vi "Coating Schedule Run Builder.vi"() -> ()   [LabVIEW 2018]
uses:
  <vilib>/Utility/miscctls.llb/LVRowAndColumnTypeDef.ctl
  <vilib>/event_ctls.llb/eventvkey.ctl
  Schedule Control Globals.vi
  <vilib>/Utility/file.llb/Read Delimited Spreadsheet (string).vi
  <vilib>/Utility/file.llb/Write Delimited Spreadsheet (string).vi
panel:
  out "Active File Changed":bool
  out "Transfer was True":bool
  out "Control Cluster was clicked":bool
  out "Track Edit Positions":T1[](array[typedef])
  out "S2 Design # and row":string[](array[string])
  out "S1 Design # and row":string[](array[string])
  out "Part Number Changed":bool
  out "Timer 1 Stpt.":i32=25
  out "Edit Position 2":T1
  out "Return Key was Pressed":bool
  out "Current Table Changed":bool
  out "Substrate Text":string
  out "Coating Que / CTCL (T)?":bool
  out "Reset Substrate Timer Start":u32
  out "Multiple Designs":bool
  out "Lookup Failed":bool
  out "SubstrateStrings":string[](array[string])
  out "Part No Found":bool
  out "Index":i32
  out "Edit Position":T1
  in  "Pick Design was True":bool
  out "Used WO's":string[](array[string])
  out "Sys Select was True":bool
  out "Time Array":string[](array[string])
  out "Part info Row":i32
  out "System No.":string
  out "Worksheet array":string[](array[string])
  out "Wavelengths & Designs":string[][](array[string])
  out "Blank":string
  in  "Diameter":string
  out "Lookup was True":bool
  out "Timer 1":i32
  in  "Tab Control":enum32{"Workcenter Report", "Run Worksheet"}(tab)=enum."Run Worksheet"
  in  "Show Part Info":bool=TRUE
  out "Report Name":string="Coating Que"
  in  "Select Action 2":bool
  in  "Select Action":bool
  out "Total Unused":i32
  out "Un-used WO's":bool caption="Showing Un-used WO's when \"ON\""
  out "last mod":u32 format="%<%m/%d/%Y>T"
  in  "Search Again":bool
  in  "Options":u16(ring) items=["Options", "Sort by Due Date", "Sort By Part Number", "Sort By Part Description", "Un-Sort / Undo", "Show New WO's Only", "Search"]
  in  "Apply to WorkSheet":bool
  out "Converted Data Table":string[][](table)
  in  "Search Text":string caption="Find What"
  in  "System Select Cluster":T2={"Select System"=1, "OK Button"=FALSE, "Cancel Button"=FALSE} {"Select System" items=["10", "20", "25", "120", "100", "41", "61", "90", "70", "160", "140", "150", "180", "190", "130", "200", "210", "220", "230", "240"]}
  in  "Always Sched. w/o OverWrite":bool caption="Always Schedule w/o Overwrite"
  in  "Include WO & PN":bool
  in  "Save Column Widths as Default":bool
  in  "Disable Pop-up":bool caption="Disable \"Design Check\" pop-up"
  in  "Reset Substrate List":bool
  in  "System Cluster 2":T3 {"Select System" items=["190", "190", "190"]}
  in  "Transfer to Schedule":bool
  out "Part Description":string caption="Part Description of Last Searched"
  in  "Control Cluster":T4
  in  "Add to Worksheet":bool
  in  "Pick Design":bool
  in  "Other Options":u16(ring) items=["Other Options", "Update Substrate List", "Print This Worksheet", "Print All Worksheets", "Open New Part Number Designs program"]
  in  "Wavelength":u16(ring) caption="Select Wavelength" items=["-"]
  in  "Substrate":u16(ring) caption="Select Substrate" items=[".55in. Quartz crystals", "AMTIR", "Al", "Aluminum", "Aluminum Tubes", "Amtir#1", "Any", "BK-7", "BK-7 Glass", "BaF2", "Be", "Bk7", "CSI", "CaF2", "CaF4", "CdS", "CdTe", "Copper", "Cu", "Cu Button", "Cu-x", "Diamond", "ER:YAG", "Fused Silica", "Fusedsilica", "GASIR-1", "GaAs", "GaAs Wafer", "Ge", "Ge Doublets", "Ge Wafers", "Glass", "Infrasil", "KBr (Salt)", "KCl", "MgO", "None", "Other", "Quartz", "SF-11", "Sapphire", "Si", "Si OG", "SiC", "Silicon Carbide", "Tool", "YAG", "YSGG", "ZnS", "ZnS (Cleartran)", "ZnS (Multispectral)", "ZnSe"]
  in  "Coating Type":u16(ring) caption="Select Coating Type / Description" items=["5 MHz Cu/Ag Crystals - side 1", "5 MHz Cu/Ag Crystals - side 1 - auto", "5 MHz Cu/Ag Crystals - side 2", "5 MHz Cu/Ag Crystals - side 2 - auto", "6 MHz Au/Ag Crystals - side 2", "6 MHz Cu/Ag Crystals - side 1"]
  in  "Design# Match/es":u16(ring) caption="Select Design#" items=["XTAL5mhzCuAgNiCrS1", "XTAL5mhzCuAgNiCrS1-auto", "Xtal17 -5mhzCuAgNiCrS1Auto"]
  in  "System Select":u16(ring) caption="Select System" items=["10", "20", "25", "120", "100", "41", "61", "90", "70", "160", "140", "150", "180", "190", "130", "200", "210", "220", "230", "240"]
  in  "Run Worksheet":string[][](table)
  out "Work Order":string
  out "Qty":string
  out "Part Number":string
  in  "Not Scheduled":bool caption="Set as Not Scheduled"
  in  "Transfer to Other Worksheet":bool caption="Move Selected Row to Different System"
  out "Coating, Wavel, Design":string[][](array[string])
  out "Build Substr":string
  out "Substrates 2":string[](array[string])
  out "Design No.":string
  in  "Data Trigger":string="f2 "
  out "Wavelength F":string
  out "Possible Designs":string[](array[string])
  out "Substrate 2":string
  out "Wavelength 2":string
  out "Coating Type 2":string
  out "Wavelengths":string[](array[string])
  in  "X-Position Array":string[](array[string])=["336", "1500", "2136", "2976", "3696", "4176", "4896", "6336", "10056", "10896", "12336", "13056", "0", "0", "0", "0", "0", "0", "0", "0", "0"]
  in  "Start Data String":string="Wavelength"
  in  "No of Columns":i32=12
  # "Coating Schedule Run Builder"
  # "Run Worksheet"
  # "Select System to Copy to"
  # "The part number was found on the system's listed.  Select one of the system's designs by selecting the system number.  Then click the desired button."
  # "Insert\n Row"
  # "Delete\nRow"
  # "Move\nUp"
  # "Move\nDown"
  # "New\nRun"
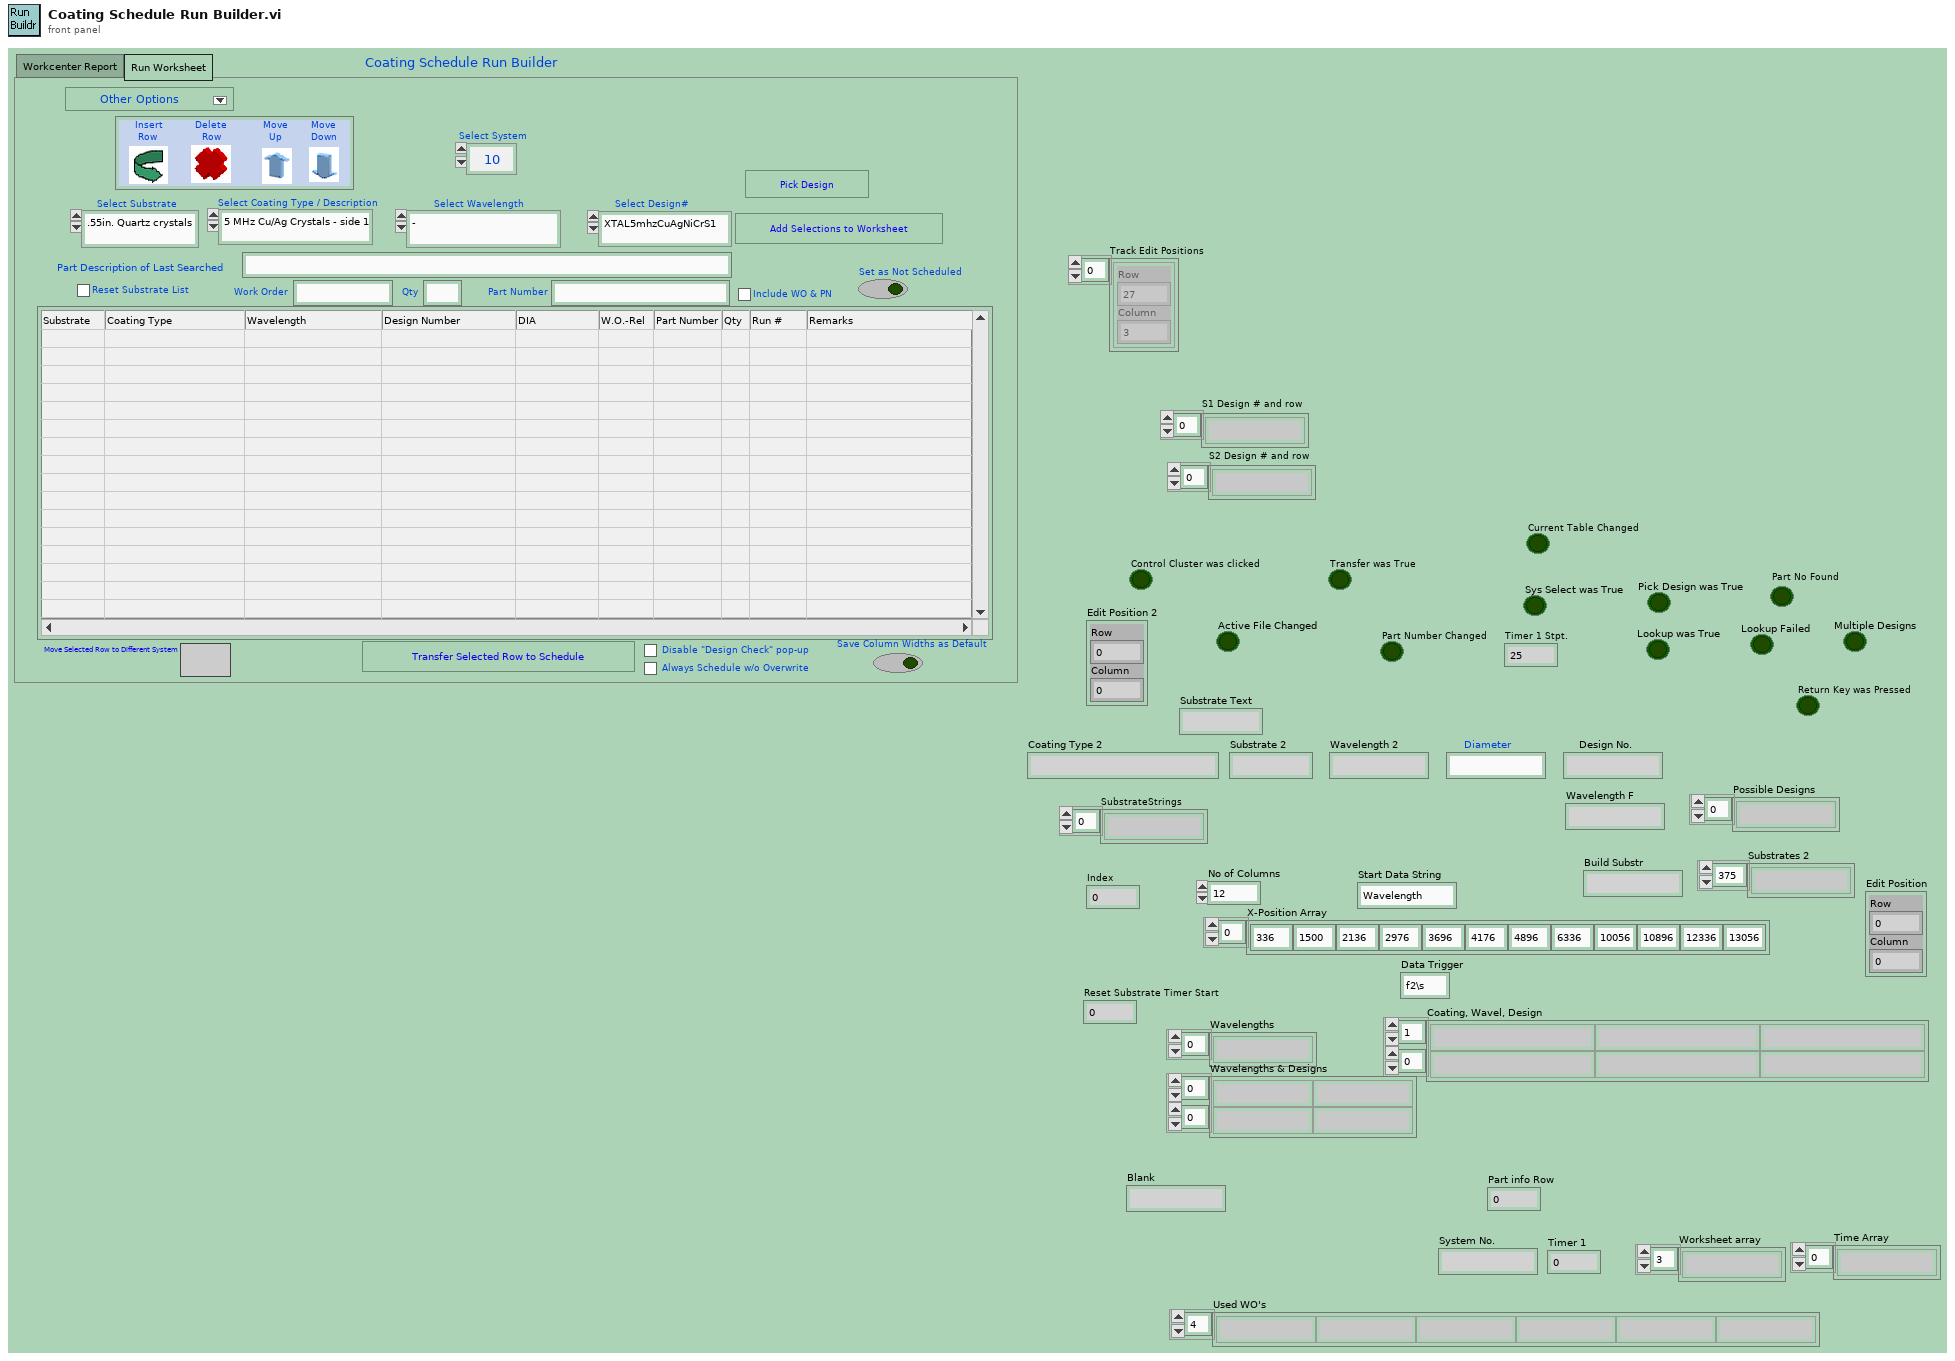
[diagram p1: front panel]
types:
  T1 = typedef "LVRowAndColumnTypeDef.ctl" = cluster{"Row":i32, "Column":i32}
  T2 = cluster{"Select System":u16, "OK Button":bool, "Cancel Button":bool}
  T3 = cluster{"Select System":u16, "OK Button":bool, "Cancel":bool, "Design #":string, "Side#":string}
  T4 = cluster{"Insert Row":bool, "Delete Row":bool, "Move Up":bool, "Move Down":bool, "New Run":bool, "Add Delay":bool}
  T5 = enum8{"Enabled", "Disabled", "Disabled and Grayed Out"}
  T6 = enum16{"Sort by Number", "Sort By Name", "Sort by Date"}
  T7 = typedef "eventvkey.ctl" = enum16{"ASCII", "Enter", "Return", "Shift", "Ctrl", "Alt", "Cmd", "Opt", "Caps", "NumLock", "Clear", "Break", "Up", "Down", "Left", "Right", "Insert", "Delete", "Home", "End", "PageUp", "PageDown", "Escape", "Help", "Pause", "ScrollLock", "F1", "F2", "F3", "F4", "F5", "F6", "F7", "F8", "F9", "F10", "F11", "F12", "F13", "F14", "F15", "F16", "F17", "F18", "F19", "F20", "F21", "F22", "F23", "F24", "Play", "VolumeUp", "VolumeDown", "Mute", "Two Byte Char"}
  T8 = cluster{"Insert Row":bool, "Insert Row":bool, "Insert Row":bool, "Insert Row":bool, "Insert Row":bool, "Insert Row":bool}
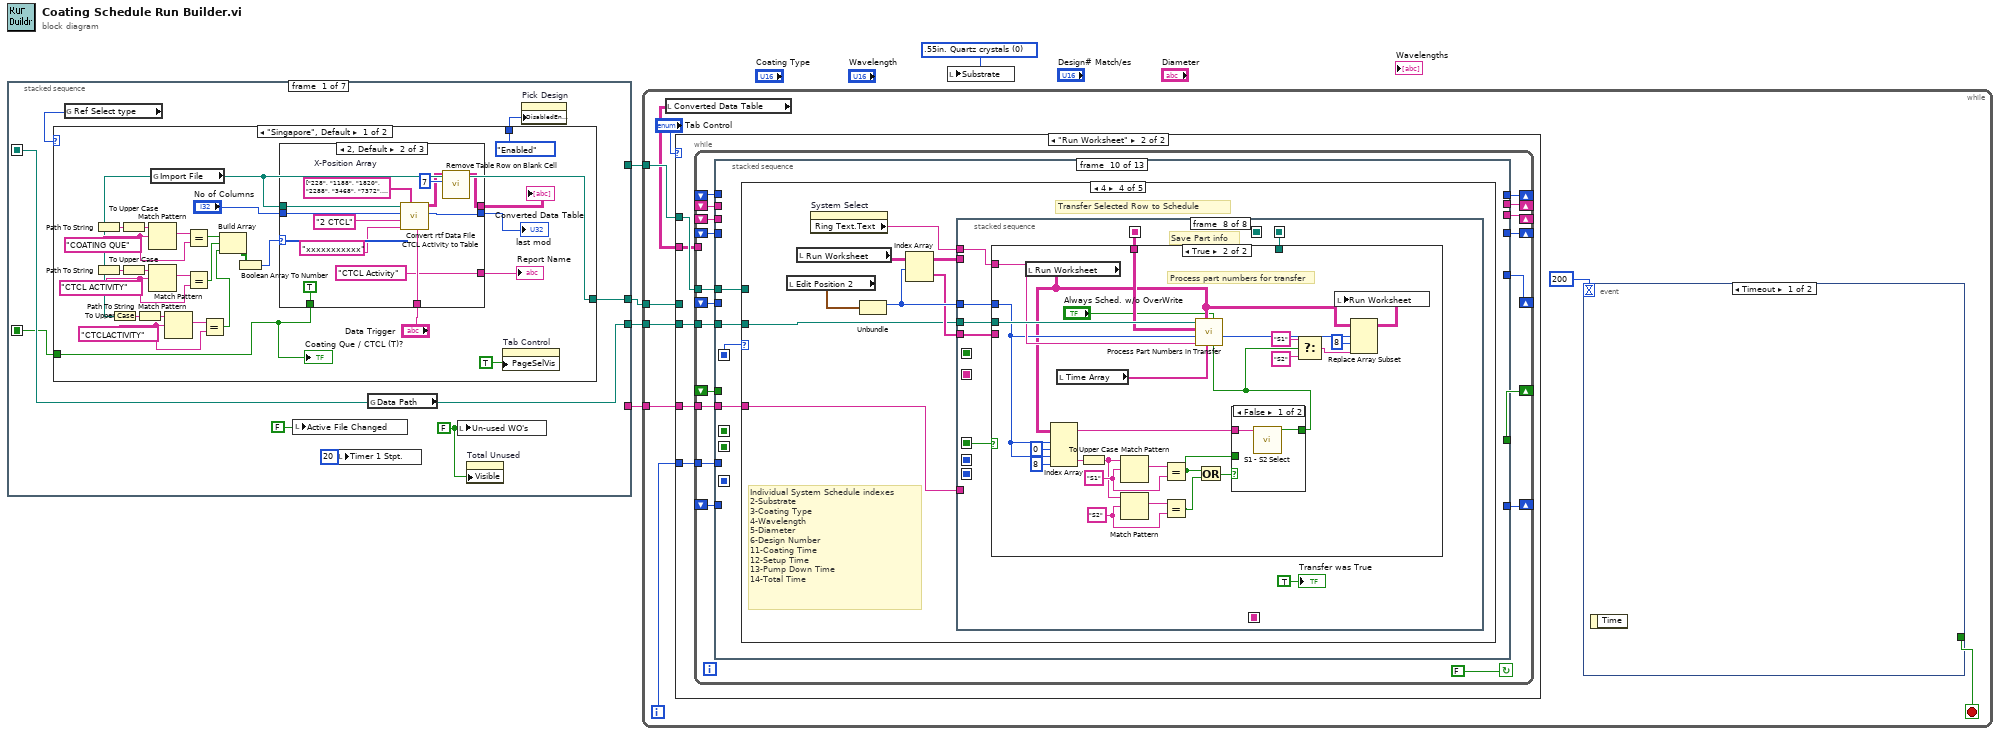
[diagram p0: block diagram]
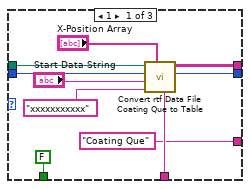
[diagram p2: hidden frame]
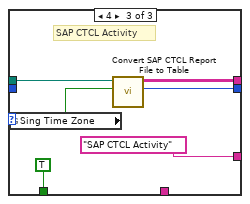
[diagram p3: hidden frame]
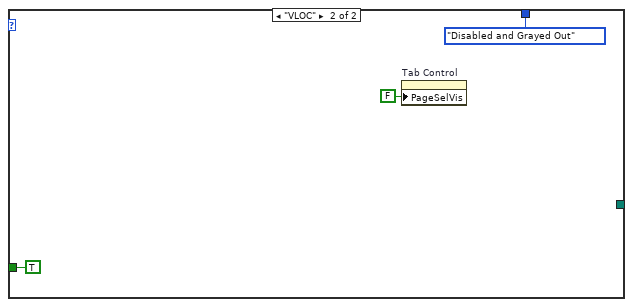
[diagram p4: hidden frame]
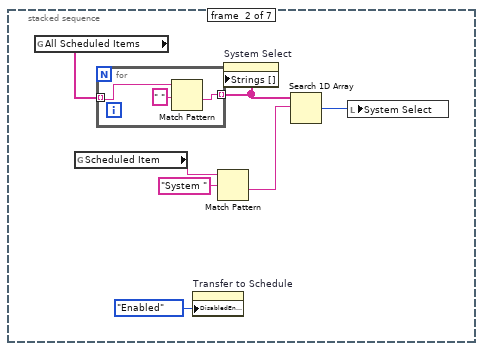
[diagram p5: hidden frame]
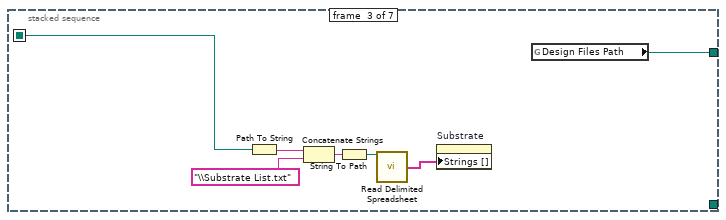
[diagram p6: hidden frame]
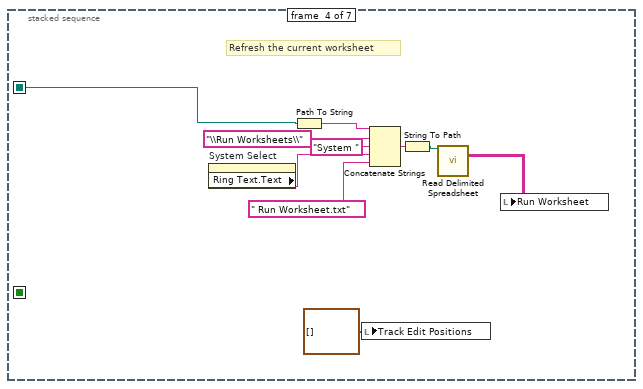
[diagram p7: hidden frame]
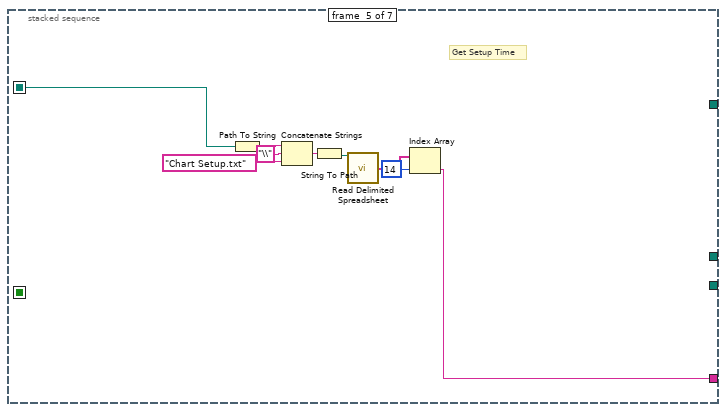
[diagram p8: hidden frame]
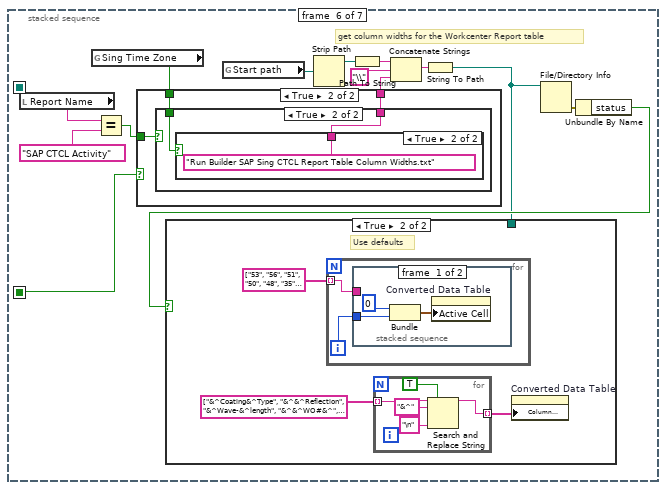
[diagram p9: hidden frame]
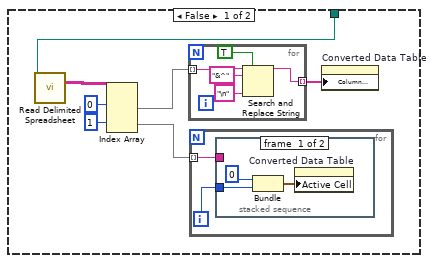
[diagram p10: hidden frame]
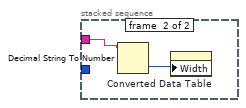
[diagram p11: hidden frame]
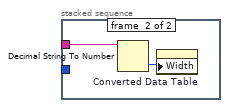
[diagram p12: hidden frame]
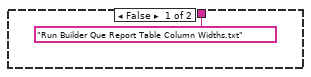
[diagram p13: hidden frame]
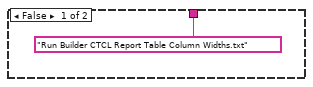
[diagram p14: hidden frame]
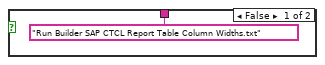
[diagram p15: hidden frame]
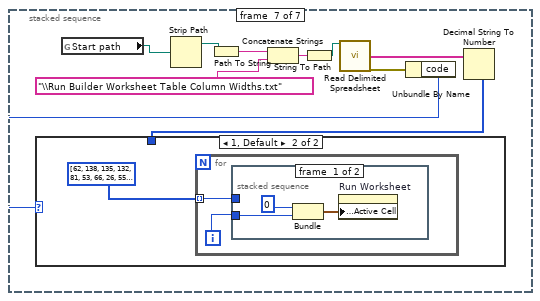
[diagram p16: hidden frame]
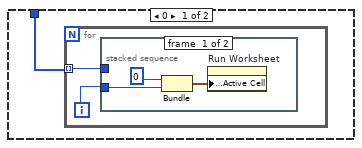
[diagram p17: hidden frame]
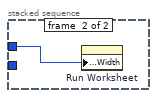
[diagram p18: hidden frame]
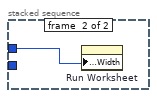
[diagram p19: hidden frame]
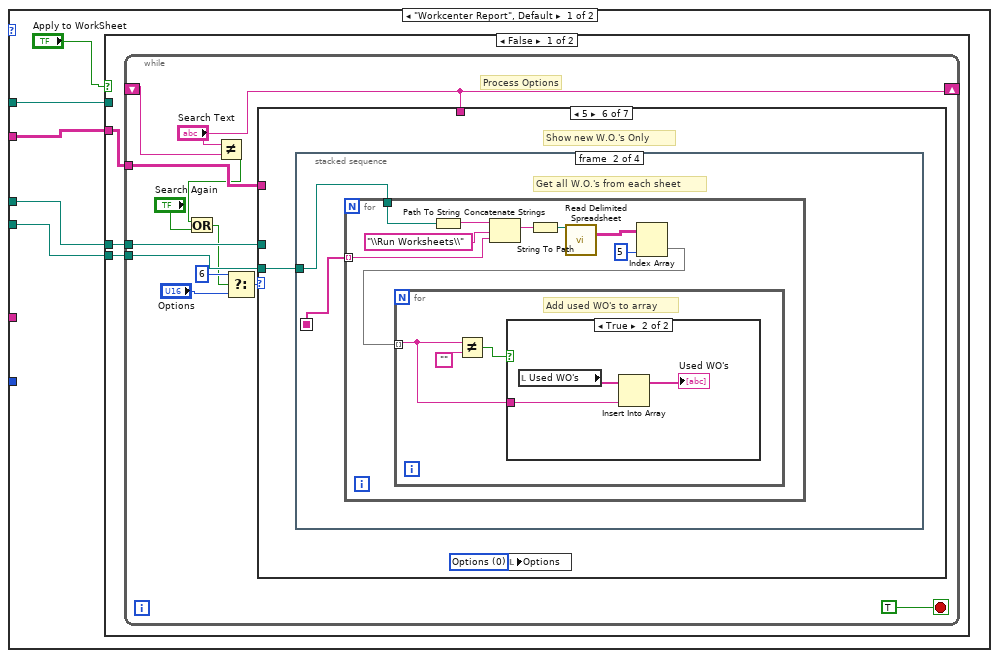
[diagram p20: hidden frame]
diagram:
  w3 = u16 0 items=[".55in. Quartz crystals", "AMTIR", "Al", "Aluminum Tubes", "Amtir#1", "Any", "Any(NT)", "BK-7", "BaF2", "Be", "Bk7", "CSI", "CaF2", "CaF4", "CdS", "CdTe", "Cu", "Diamond", "ER:YAG", "Fused Silica", "GASIR-1", "GLASS", "GaAs", "GaAs Wafer", "Ge", "Ge Doublets", "Ge Wafers", "Glass", "Infrasil", "KBr (Salt)", "KCl", "MgO", "None", "Other", "Quartz", "SF-11", "Sapphire", "Si", "Si OG", "SiC", "Tool", "YAG", "YSGG", "ZnS", "ZnS (Cleartran)", "ZnS (Multispectral)", "ZnSe"] ("Substrate")
  n1 = stacked-sequence {
    seq-local: [w13 _ _ _ _ _ _] -> [_ _ w83 w91 w102 _ _]
    seq-local: [w8 _ _ _ _ _ _] -> [_ _ _ _ _ w111 _]
    tunnel: [w13 _ _ _ _ _ _] -> w5
    tunnel: [_ _ w87 _ _ _ _] -> w4
    tunnel: [w11 _ _ _ _ _ _] -> w2
    tunnel: [_ _ _ _ w100 _ _] -> w1
    frame #0 {
      w12 = FALSE ("Un-used WO's")
      n2 = global read "Schedule Control Globals.vi" "Ref Select type"() -> (w10:enum32{"Singapore", "VLOC"})
      n3 = case shown="\"Singapore\", Default" w10 {
        tunnel: [w20 _] -> w11
        tunnel: [T5."Enabled" ("Disabled") T5."Disabled and Grayed Out" ("Disabled")] -> w9
        tunnel: [w15 TRUE] -> w8
        frame "Singapore", Default {
          w19 = "CTCLACTIVITY" ("regular expression")
          w26 = "CTCL ACTIVITY" ("regular expression")
          w31 = "COATING QUE" ("regular expression")
          n4 = global read "Schedule Control Globals.vi" "Import File"() -> (w20:path)
          n5 = Path To String(path=w20) -> (string=w34:string)
          n6 = Path To String(path=w20) -> (string=w29:string)
          n7 = Path To String(path=w20) -> (string=w23:string)
          n8 = To Upper Case(1:w34) -> (0:w33:string)
          n9 = To Upper Case(1:w29) -> (0:w28:string)
          n10 = To Upper Case(1:w23) -> (0:w22:string)
          n11 = Match Pattern(string=w33, regular expression=w31) -> (match substring=w32:string)  [unwired: 1 in, 3 out]
          n12 = Match Pattern(string=w28, regular expression=w26) -> (match substring=w27:string)  [unwired: 1 in, 3 out]
          n13 = Match Pattern(string=w22, regular expression=w19) -> (match substring=w21:string)  [unwired: 1 in, 3 out]
          n14 = Equal?(x=w32, y=w31) -> (x = y?=w25:bool)
          n15 = Equal?(x=w27, y=w26) -> (x = y?=w24:bool)
          n16 = Equal?(x=w21, y=w19) -> (x = y?=w18:bool)
          n17 = Build Array(w25, w24, w18) -> (w17:bool[])
          n18 = Boolean Array To Number(Boolean array=w17) -> (number=w16:u32)
          n19 = case shown="2, Default" w16 {
            tunnel: "No of Columns" -> [w49 w61 _]
            tunnel: "Data Trigger" -> [w48 w58 _]
            tunnel: [w47 w51 w66] -> w14
            tunnel: [w46 w60 w65] -> w37
            tunnel: w20 -> [w45 w59 w67]
            tunnel: ["Coating Que" ("Report Name") "CTCL Activity" ("Report Name") "SAP CTCL Activity" ("Report Name")] -> w30
            tunnel: [FALSE TRUE TRUE] -> w15
            frame 1 {
              n20 = call "Convert rtf Data File Coating Que to Table.vi"("File Path"=w45, "No of Columns"=w49, "Start Data String"="Start Data String", "End of Data String"="xxxxxxxxxxx", "X-Position Array"="X-Position Array", "Data Trigger"=w48) -> ("Converted Data Table"=w47:string[][], "last mod"=w46:u32)  [unwired: 3 in]
            }
            frame 2, Default {
              w56 = string[] ["228", "1188", "1820", "2288", "3468", "7372", "7788", "8212", "11028", "13668", "0", "0", "0", "0", "0", "0", "0", "0", "0", "0", "0"]  # X-Position Array
              n21 = call "Convert rtf Data File CTCL Activity to Table.vi"("File Path"=w59, "No of Columns"=w61, "Start Data String"="2 CTCL", "End of Data String"="xxxxxxxxxxx", "X-Position Array"=w56, "Data Trigger"=w58) -> ("Converted Data Table"=w52:string[][], "last mod"=w60:u32)  [unwired: 3 in]
              n22 = call "Remove Table Row on Blank Cell.vi"("Column"=7, "Table In"=w52) -> ("Table Out"=w51:string[][])  [unwired: 9 in]
            }
            frame 4 {
              # "SAP CTCL Activity"
              n23 = global read "Schedule Control Globals.vi" "Sing Time Zone"() -> (w62:bool)
              n24 = call "Convert SAP CTCL Report File to Table.vi"("File Path"=w67, "Sing Time Zone"=w62) -> ("Converted Data Table"=w66:string[][], "last mod"=w65:u32)  [unwired: 7 in]
            }
          }
          "last mod" <- w37
          "Report Name" <- w30
          "Coating Que / CTCL (T)?" <- w15
          "Converted Data Table" <- w14
          n25 = property on="Tab Control" class="TabCtl (strict)"("PageSelVis"=TRUE ("Page Selector Visible")) -> ()  [unwired: 2 in, 2 out]
        }
        frame "VLOC" {
          n26 = property on="Tab Control" class="TabCtl (strict)"("PageSelVis"=FALSE ("Page Selector Visible")) -> ()  [unwired: 2 in, 2 out]
        }
      }
      n27 = local write "Active File Changed"(FALSE ("Active File Changed")) -> ()
      n28 = local write "Timer 1 Stpt."(20 ("Timer Stpt.")) -> ()
      n29 = global read "Schedule Control Globals.vi" "Data Path"() -> (w13:path)
      n30 = local write "Un-used WO's"(w12) -> ()
      n31 = property on="Total Unused" class="DigNum (strict)"("Visible"=w12) -> ()  [unwired: 2 in, 2 out]
      n32 = property on="Pick Design" class="Bool"("DisabledEnum"=w9) -> ()  [unwired: 2 in, 2 out]
    }
    frame #1 {
      n33 = global read "Schedule Control Globals.vi" "All Scheduled Items"() -> (w73:string[])
      n34 = global read "Schedule Control Globals.vi" "Scheduled Item"() -> (w72:string)
      n35 = for {
        tunnel: w73 -> [w80] mode=indexing
        tunnel: [w78] -> w77 mode=indexing
        n36 = Match Pattern(string=w80, regular expression=" ") -> (after substring=w78:string)  [unwired: 1 in, 3 out]
      }
      n37 = property on="Transfer to Schedule" class="Bool"("DisabledEnum"=T5."Enabled" ("Disabled")) -> ()  [unwired: 2 in, 2 out]
      n38 = Match Pattern(string=w72, regular expression="System ") -> (after substring=w75:string)  [unwired: 1 in, 3 out]
      n39 = property on="System Select" class="Ring (strict)"("Strings []"=w77) -> ()  [unwired: 2 in, 2 out]
      n40 = Search 1D Array(1D array=w77, element=w75) -> (index of element=w76:i32)  [unwired: 1 in]
      n41 = local write "System Select"(w76) -> ()
    }
    frame #2 {
      n42 = Path To String(path=w83) -> (string=w85:string)
      n43 = Concatenate Strings(w85, "\\Substrate List.txt" ("string")) -> (w86:string)
      n44 = String To Path(string=w86) -> (path=w82:path)
      n45 = call-poly <vilib>:"Read Delimited Spreadsheet.vi"("file path (dialog if empty)"=w82) -> ("first row"=w81:string[])  [unwired: 9 in, 5 out]
      n46 = property on="Substrate" class="Ring (strict)"("Strings []"=w81) -> ()  [unwired: 2 in, 2 out]
      n47 = global read "Schedule Control Globals.vi" "Design Files Path"() -> (w87:path)
    }
    frame #3 {
      # "Refresh the current worksheet"
      n48 = property on="System Select" class="Ring (strict)"() -> ("Ring Text.Text"=w96:string)  [unwired: 2 in, 2 out]
      n49 = Path To String(path=w91) -> (string=w94:string)
      n50 = local write "Track Edit Positions"(T1[] [] ("Track Edit Positions")) -> ()
      n51 = Concatenate Strings(w94, "\\Run Worksheets\\" ("string"), "System " ("string"), w96, " Run Worksheet.txt" ("string")) -> (w92:string)
      n52 = String To Path(string=w92) -> (path=w90:path)
      n53 = call-poly <vilib>:"Read Delimited Spreadsheet.vi"("file path (dialog if empty)"=w90) -> ("all rows"=w89:string[][])  [unwired: 9 in, 5 out]
      n54 = local write "Run Worksheet"(w89) -> ()
    }
    frame #4 {
      # "Get Setup Time"
      n55 = Path To String(path=w102) -> (string=w106:string)
      n56 = Concatenate Strings(w106, "\\" ("string"), "Chart Setup.txt" ("string")) -> (w104:string)
      n57 = String To Path(string=w104) -> (path=w99:path)
      n58 = call-poly <vilib>:"Read Delimited Spreadsheet.vi"("file path (dialog if empty)"=w99) -> ("first row"=w98:string[])  [unwired: 9 in, 5 out]
      n59 = Index Array(array=w98, index=14) -> (element=w100:string)
    }
    frame #5 {
      # "get column widths for the Workcenter Report table"
      n60 = local read "Report Name"() -> (w110:string)
      n61 = global read "Schedule Control Globals.vi" "Sing Time Zone"() -> (w107:bool)
      n62 = Equal?(x=w110, y="SAP CTCL Activity" ("Report Name")) -> (x = y?=w108:bool)
      n63 = case shown="True" w111 {
        tunnel: ["Run Builder Que Report Table Column Widths.txt" ("text") w157] -> w112
        tunnel: w108 -> [_ w158]
        tunnel: w107 -> [_ w156]
        frame False {
        }
        frame True {
          n64 = case shown="True" w158 {
            tunnel: ["Run Builder CTCL Report Table Column Widths.txt" ("text") w161] -> w157
            tunnel: w156 -> [_ w160]
            frame False {
            }
            frame True {
              n65 = case shown="True" w160 {
                tunnel: ["Run Builder SAP CTCL Report Table Column Widths.txt" ("text") "Run Builder SAP Sing CTCL Report Table Column Widths.txt" ("text")] -> w161
                frame False {
                }
                frame True {
                }
              }
            }
          }
        }
      }
      n66 = global read "Schedule Control Globals.vi" "Start path"() -> (w120:path)
      n67 = Strip Path(path=w120) -> (stripped path=w119:path)  [unwired: 1 out]
      n68 = Path To String(path=w119) -> (string=w118:string)
      n69 = Concatenate Strings(w118, "\\" ("string"), w112) -> (w116:string)
      n70 = String To Path(string=w116) -> (path=w113:path)
      n71 = File/Directory Info(path=w113) -> (error out=w115:errorcluster)  [unwired: 1 in, 6 out]
      n72 = Unbundle By Name(w115) -> ("status"=w114:bool)
      n73 = case shown="True" w114 {
        tunnel: w113 -> [w122 _]
        frame False {
          n74 = call-poly <vilib>:"Read Delimited Spreadsheet.vi"("file path (dialog if empty)"=w122) -> ("all rows"=w121:string[][])  [unwired: 9 in, 5 out]
          n75 = Index Array(array=w121, index (row) #1=0 ("index (row)"), index (row) #2=1 ("index (row)")) -> (element #1=w124:string[], element #2=w125:string[])  [unwired: 2 in]
          n76 = for {
            tunnel: w124 -> [w132] mode=indexing
            tunnel: [w128] -> w123 mode=indexing
            n77 = Search and Replace String(replace all?=TRUE ("replace all? (F)"), input string=w132, search string="&^", replace string="\n" ("replace string (\"\")")) -> (result string=w128:string)  [unwired: 4 in, 3 out]
          }
          n78 = for {
            tunnel: w125 -> [w133] mode=indexing
            i -> [w134]
            n79 = stacked-sequence {
              tunnel: w134 -> [w137 _]
              tunnel: w133 -> [_ w139]
              frame #0 {
                n80 = Bundle(0, w137) -> (w135:cluster{i32, i32})  [unwired: 1 in]
                n81 = property on="Converted Data Table" class="Tbl (strict)"("Active Cell"=w135) -> ()  [unwired: 2 in, 2 out]
              }
              frame #1 {
                n82 = Decimal String To Number(string=w139) -> (number=w138:i32)  [unwired: 2 in, 1 out]
                n83 = property on="Converted Data Table" class="Tbl (strict)"("Width"=w138) -> ()  [unwired: 2 in, 2 out]
              }
            }
          }
          n84 = property on="Converted Data Table" class="Tbl (strict)"("Column Headers[]"=w123) -> ()  [unwired: 2 in, 2 out]
        }
        frame True {
          # "Use defaults"
          n85 = for {
            tunnel: string[] ["53", "56", "51", "50", "48", "35", "63", "360", "52", "138", "45", "48", "50", "50", "50", "50", "44", "47", "44", "50", "282"] ("decimal integer string") -> [w148] mode=indexing
            i -> [w149]
            n86 = stacked-sequence {
              tunnel: w149 -> [w152 _]
              tunnel: w148 -> [_ w154]
              frame #0 {
                n87 = Bundle(0, w152) -> (w150:cluster{i32, i32})  [unwired: 1 in]
                n88 = property on="Converted Data Table" class="Tbl (strict)"("Active Cell"=w150) -> ()  [unwired: 2 in, 2 out]
              }
              frame #1 {
                n89 = Decimal String To Number(string=w154) -> (number=w153:i32)  [unwired: 2 in, 1 out]
                n90 = property on="Converted Data Table" class="Tbl (strict)"("Width"=w153) -> ()  [unwired: 2 in, 2 out]
              }
            }
          }
          n91 = for {
            tunnel: string[] ["&^Coating&^Type", "&^&^Reflection", "&^Wave-&^length", "&^&^WO#&^", "&^&^Release", "&^Open&^Qty", "&^Part&^Number", "&^Part&^Description", "&^Due&^Date", "&^&^Customer", "&^&^SO#", "&^Lab&^Hours", "", "", "", "", "", "", "&^&^", "&^&^", "&^&^"] ("Array") -> [w147] mode=indexing
            tunnel: [w143] -> w140 mode=indexing
            n92 = Search and Replace String(replace all?=TRUE ("replace all? (F)"), input string=w147, search string="&^", replace string="\n" ("replace string (\"\")")) -> (result string=w143:string)  [unwired: 4 in, 3 out]
          }
          n93 = property on="Converted Data Table" class="Tbl (strict)"("Column Headers[]"=w140) -> ()  [unwired: 2 in, 2 out]
        }
      }
    }
    frame #6 {
      n94 = global read "Schedule Control Globals.vi" "Start path"() -> (w169:path)
      n95 = Strip Path(path=w169) -> (stripped path=w171:path)  [unwired: 1 out]
      n96 = Path To String(path=w171) -> (string=w170:string)
      n97 = Concatenate Strings(w170, "\\Run Builder Worksheet Table Column Widths.txt" ("string")) -> (w173:string)
      n98 = String To Path(string=w173) -> (path=w167:path)
      n99 = call-poly <vilib>:"Read Delimited Spreadsheet.vi"("file path (dialog if empty)"=w167) -> ("first row"=w166:string[], "error out"=w165:errorcluster)  [unwired: 9 in, 4 out]
      n100 = Unbundle By Name(w165) -> ("code"=w164:i32)
      n101 = Decimal String To Number(string=w166) -> (number=w172:i32[])  [unwired: 2 in, 1 out]
      n102 = case shown="1, Default" w164 {
        tunnel: w172 -> [w174 _]
        frame 0 {
          n103 = for {
            tunnel: w174 -> [w175] mode=indexing
            i -> [w176]
            n104 = stacked-sequence {
              tunnel: w176 -> [w179 _]
              tunnel: w175 -> [_ w180]
              frame #0 {
                n105 = Bundle(0, w179) -> (w177:cluster{i32, i32})  [unwired: 1 in]
                n106 = property on="Run Worksheet" class="Tbl (strict)"("Active Cell:Active Cell"=w177) -> ()  [unwired: 2 in, 2 out]
              }
              frame #1 {
                n107 = property on="Run Worksheet" class="Tbl (strict)"("Active Cell:Cell Size:Width"=w180) -> ()  [unwired: 2 in, 2 out]
              }
            }
          }
        }
        frame 1, Default {
          n108 = for {
            tunnel: u32[] [62, 138, 135, 132, 81, 53, 66, 26, 55, 173, 80, 63] ("Array") -> [w182] mode=indexing
            i -> [w183]
            n109 = stacked-sequence {
              tunnel: w183 -> [w186 _]
              tunnel: w182 -> [_ w187]
              frame #0 {
                n110 = Bundle(0, w186) -> (w184:cluster{i32, i32})  [unwired: 1 in]
                n111 = property on="Run Worksheet" class="Tbl (strict)"("Active Cell:Active Cell"=w184) -> ()  [unwired: 2 in, 2 out]
              }
              frame #1 {
                n112 = property on="Run Worksheet" class="Tbl (strict)"("Active Cell:Cell Size:Width"=w187) -> ()  [unwired: 2 in, 2 out]
              }
            }
          }
        }
      }
    }
  }
  n113 = while {
    tunnel: w5 -> [w196]
    tunnel: w4 -> [w195]
    tunnel: w2 -> [w190]
    tunnel: w1 -> [w189]
    i -> [w191]
    stop <- w193 stop-if-true
    n114 = local read "Converted Data Table"() -> (w188:string[][])
    n115 = case shown="\"Run Worksheet\"" "Tab Control" {
      tunnel: w196 -> [w201 w1124]
      tunnel: w188 -> [w200 w1125]
      tunnel: w195 -> [w199 w1126]
      tunnel: w191 -> [_ w1123]
      tunnel: w190 -> [w198 _]
      tunnel: w189 -> [_ w1122]
      frame "Workcenter Report", Default {
        n116 = case shown="False" "Apply to WorkSheet" {
          tunnel: w201 -> [w203 w434]
          tunnel: w200 -> [w204 w436]
          tunnel: w199 -> [_ w435]
          tunnel: w198 -> [w202 _]
          frame False {
            n117 = while {
              tunnel: w204 -> [w216]
              tunnel: w203 -> [w215]
              tunnel: w202 -> [w214]
              shift-right: ["Search Text"] -> _
              shift-left: _ -> [w212]
              stop <- TRUE stop-if-true
              # "Process Options"
              n118 = Not Equal?(x="Search Text", y=w212) -> (x != y?=w205:bool)
              n119 = Or(x=w205, y="Search Again") -> (x .or. y?=w207:bool)
              n120 = Select(t=u16 6, s=w207, f="Options") -> (s? t:f=w208:u16)
              n121 = case shown="5" w208 {
                tunnel: w216 -> [_ w263 w279 w298 _ _ w423]
                tunnel: w215 -> [_ _ _ _ _ w347 _]
                tunnel: w214 -> [_ _ _ _ w318 _ _]
                tunnel: "Search Text" -> [_ _ _ _ _ _ w419]
                frame 0, Default {
                  n122 = local read "Select Action"() -> (w220:bool)
                  n123 = property on="Converted Data Table" class="Tbl (strict)"() -> ("EditPos"=w222:T1)  [unwired: 2 in, 2 out]
                  n124 = local write "Lookup was True"(FALSE ("Lookup was True")) -> ()
                  n125 = Unbundle(w222) -> ("Row"=w224:i32)  [unwired: 1 out]
                  n126 = local read "Pick Design was True"() -> (w219:bool)
                  n127 = property on="Select Action 2" class="Bool (strict)"("Visible"=w220) -> ()  [unwired: 2 in, 2 out]
                  n128 = Not Equal?(x=w224, y=-2) -> (x != y?=w221:bool)
                  n129 = case shown="True" w221 {
                    tunnel: w222 -> [_ w227]
                    tunnel: "Show Part Info" -> [_ w226]
                    frame False {
                    }
                    frame True {
                      # "Look up Part info for select row"
                      n130 = case shown="True" w226 {
                        tunnel: w227 -> [_ w228]
                        frame False {
                        }
                        frame True {
                          n131 = stacked-sequence {
                            seq-local: [w229 _] -> [_ w235]
                            tunnel: w228 -> [_ w237]
                            frame #0 {
                              n132 = global read "Schedule Control Globals.vi" "Data Path"() -> (w233:path)
                              n133 = Path To String(path=w233) -> (string=w232:string)
                              n134 = Concatenate Strings(w232, "\\Part Number Info.txt" ("string")) -> (w231:string)
                              n135 = String To Path(string=w231) -> (path=w234:path)
                              n136 = call-poly <vilib>:"Read Delimited Spreadsheet.vi"("file path (dialog if empty)"=w234) -> ("all rows"=w229:string[][])  [unwired: 9 in, 5 out]
                            }
                            frame #1 {
                              # "Part Number Info table"
                              n137 = Index Array(array=w235, index (col)=0 ("disabled index (col)")) -> (element=w243:string[])  [unwired: 1 in]
                              n138 = local read "Converted Data Table"() -> (w238:string[][])
                              n139 = Unbundle By Name(w237) -> ("Row"=w239:i32)
                              n140 = Index Array(array=w238, index (row)=w239, index (col)=3 ("disabled index (col)")) -> (element=w242:string)
                              n141 = for {
                                shift-right: [w246] -> w236
                                shift-left: string[][] [] ("Sorted Table") -> [w247]
                                tunnel: w242 -> [w250]
                                tunnel: w243 -> [w249] mode=indexing
                                tunnel: w235 -> [w245] mode=indexing
                                n142 = Equal?(x=w249, y=w250) -> (x = y?=w248:bool)
                                n143 = case shown="True" w248 {
                                tunnel: w247 -> [w251 w256]
                                tunnel: [w251 w255] -> w246
                                tunnel: w245 -> [_ w254]
                                frame False {
                                }
                                frame True {
                                n144 = Array Subset(array=w254, length=10) -> (w252:string[])  [unwired: 1 in]
                                n145 = Insert Into Array(array=w256, new element=w252) -> (w255:string[][])  [unwired: 2 in]
                                }
                                }
                              }
                              n146 = call "Show Part Info.vi"("Part Info"=w236) -> ()  [unwired: 11 in]
                            }
                          }
                        }
                      }
                      "Edit Position" <- w227
                    }
                  }
                  n147 = case shown="True" w219 {
                    frame False {
                    }
                    frame True {
                      # "Reset substate list after pick design."
                      n148 = local read "SubstrateStrings"() -> (w225:string[])
                      n149 = property on="Substrate" class="Ring (strict)"("Strings []"=w225) -> ()  [unwired: 2 in, 2 out]
                    }
                  }
                }
                frame 1 {
                  w258 = FALSE ("Visible")
                  w261 = 8 ("Column to Sort")
                  w264 = u16 0 items=["SORT BY", "Due Date", "No Sort"] ("Sort")
                  # "Sort by Due Date"
                  n150 = for {
                    tunnel: w263 -> [w271] mode=indexing
                    tunnel: w261 -> [w266]
                    tunnel: [w265] -> w260 mode=indexing
                    # "Fill Blanks"
                    n151 = Index Array(array=w271, index=w266) -> (element=w268:string)
                    n152 = Not Equal?(x=w268, y="") -> (x != y?=w269:bool)
                    n153 = case shown="True" w269 {
                      tunnel: w268 -> [_ w273]
                      tunnel: [w272 w273] -> w267
                      frame False {
                        n154 = local read "Blank"() -> (w272:string)
                      }
                      frame True {
                        "Blank" <- w273
                      }
                    }
                    n155 = Replace Array Subset(array=w271, new element=w267, index=w266) -> (w265:string[])
                  }
                  n156 = local write "Options"(w264) -> ()
                  n157 = global read "Schedule Control Globals.vi" "Sing Time Zone"() -> (w257:bool)
                  n158 = call "Sort List - Sched.vi"("Table In"=w260, "Column to Sort"=w261, "Sort Select"=T6."Sort by Date", "Asc (T) - Desc"=w257) -> ("Sorted Table"=w259:string[][])  [unwired: 4 in]
                  n159 = local write "Converted Data Table"(w259) -> ()
                  n160 = property on="Search Text" class="Str"("Visible"=w258) -> ()  [unwired: 2 in, 2 out]
                  n161 = property on="Search Again" class="Bool"("Visible"=w258) -> ()  [unwired: 2 in, 2 out]
                }
                frame 2 {
                  w278 = FALSE ("Visible")
                  w283 = u16 0 items=["Options", "Sort by Due Date", "Sort By Part Number", "Un-Sort / Undo", "Show New WO's Only"] ("Options")
                  # "Sort by Part Number"
                  n162 = local read "Coating Que / CTCL (T)?"() -> (w274:bool)
                  n163 = Select(t=3, s=w274, f=6 ("Column to Sort")) -> (s? t:f=w275:i32)
                  n164 = property on="Search Again" class="Bool"("Visible"=w278) -> ()  [unwired: 2 in, 2 out]
                  n165 = property on="Search Text" class="Str"("Visible"=w278) -> ()  [unwired: 2 in, 2 out]
                  n166 = for {
                    tunnel: w279 -> [w290] mode=indexing
                    tunnel: w275 -> [w285]
                    tunnel: [w284] -> w281 mode=indexing
                    # "Fill Blanks"
                    n167 = Index Array(array=w290, index=w285) -> (element=w287:string)
                    n168 = Not Equal?(x=w287, y="") -> (x != y?=w288:bool)
                    n169 = case shown="True" w288 {
                      tunnel: w287 -> [_ w292]
                      tunnel: [w291 w292] -> w286
                      frame False {
                        n170 = local read "Blank"() -> (w291:string)
                      }
                      frame True {
                        n171 = local write "Blank"(w292) -> ()
                      }
                    }
                    n172 = Replace Array Subset(array=w290, new element=w286, index=w285) -> (w284:string[])
                  }
                  n173 = local write "Options"(w283) -> ()
                  n174 = call "Sort List - Sched.vi"("Table In"=w281, "Column to Sort"=w275, "Sort Select"=T6."Sort by Number") -> ("Sorted Table"=w280:string[][])  [unwired: 5 in]
                  n175 = local write "Converted Data Table"(w280) -> ()
                }
                frame 3 {
                  w297 = FALSE ("Visible")
                  w302 = u16 0 items=["Options", "Sort by Due Date", "Sort By Part Number", "Un-Sort / Undo", "Show New WO's Only"] ("Options")
                  # "Sort by Part Description"
                  n176 = local read "Coating Que / CTCL (T)?"() -> (w295:bool)
                  n177 = Select(t=4, s=w295, f=7 ("Column to Sort")) -> (s? t:f=w293:i32)
                  n178 = property on="Search Again" class="Bool"("Visible"=w297) -> ()  [unwired: 2 in, 2 out]
                  n179 = property on="Search Text" class="Str"("Visible"=w297) -> ()  [unwired: 2 in, 2 out]
                  n180 = for {
                    tunnel: w298 -> [w309] mode=indexing
                    tunnel: w293 -> [w304]
                    tunnel: [w303] -> w300 mode=indexing
                    # "get rid of blank part descriptions"
                    n181 = Index Array(array=w309, index=w304) -> (element=w306:string)
                    n182 = Not Equal?(x=w306, y="") -> (x != y?=w307:bool)
                    n183 = case shown="False" w307 {
                      tunnel: w306 -> [_ w311]
                      tunnel: [w310 w311] -> w305
                      frame False {
                        n184 = local read "Blank"() -> (w310:string)
                      }
                      frame True {
                        n185 = local write "Blank"(w311) -> ()
                      }
                    }
                    n186 = Replace Array Subset(array=w309, new element=w305, index=w304) -> (w303:string[])
                  }
                  n187 = local write "Options"(w302) -> ()
                  n188 = call "Sort List - Sched.vi"("Table In"=w300, "Column to Sort"=w293, "Sort Select"=T6."Sort By Name") -> ("Sorted Table"=w299:string[][])  [unwired: 5 in]
                  n189 = local write "Converted Data Table"(w299) -> ()
                }
                frame 4 {
                  w316 = FALSE ("Visible")
                  w317 = FALSE ("Un-used WO's")
                  w319 = u16 0 items=["SORT BY", "Due Date", "No Sort"] ("Sort")
                  # "Un Sort"
                  n190 = local read "Coating Que / CTCL (T)?"() -> (w315:bool)
                  n191 = local read "No of Columns"() -> (w314:i32)
                  n192 = local write "Options"(w319) -> ()
                  n193 = local read "Data Trigger"() -> (w312:string)
                  n194 = case shown="True" w315 {
                    tunnel: [w325 w332] -> w320
                    tunnel: w318 -> [w324 w337]
                    tunnel: w314 -> [w323 w336]
                    tunnel: "xxxxxxxxxxx" ("End of Data String") -> [w322 w335]
                    tunnel: w312 -> [w321 w334]
                    frame False {
                      n195 = local read "Start Data String"() -> (w326:string)
                      n196 = local read "X-Position Array"() -> (w327:string[])
                      n197 = call "Convert rtf Data File Coating Que to Table.vi"("File Path"=w324, "No of Columns"=w323, "Start Data String"=w326, "End of Data String"=w322, "X-Position Array"=w327, "Data Trigger"=w321) -> ("Converted Data Table"=w325:string[][])  [unwired: 3 in, 1 out]
                    }
                    frame True {
                      # "Show only rows with Qty > 0\nfor column 7"
                      n198 = local read "Report Name"() -> (w330:string)
                      n199 = Equal?(x=w330, y="CTCL Activity" ("Report Name")) -> (x = y?=w328:bool)
                      n200 = case shown="True" w328 {
                        tunnel: w337 -> [w339 w344]
                        tunnel: w336 -> [_ w343]
                        tunnel: w335 -> [_ w342]
                        tunnel: w334 -> [_ w341]
                        tunnel: [w338 w340] -> w333
                        frame False {
                          n201 = call "Convert SAP CTCL Report File to Table.vi"("File Path"=w339) -> ("Converted Data Table"=w338:string[][])  [unwired: 8 in, 1 out]
                        }
                        frame True {
                          w346 = string[] ["228", "1188", "1820", "2288", "3468", "7372", "7788", "8212", "11028", "13668", "0", "0", "0", "0", "0", "0", "0", "0", "0", "0", "0"]  # X-Position Array
                          n202 = call "Convert rtf Data File CTCL Activity to Table.vi"("File Path"=w344, "No of Columns"=w343, "Start Data String"="2 CTCL", "End of Data String"=w342, "X-Position Array"=w346, "Data Trigger"=w341) -> ("Converted Data Table"=w340:string[][])  [unwired: 3 in, 1 out]
                        }
                      }
                      n203 = call "Remove Table Row on Blank Cell.vi"("Column"=7, "Table In"=w333) -> ("Table Out"=w332:string[][])  [unwired: 9 in]
                    }
                  }
                  n204 = property on="Search Again" class="Bool"("Visible"=w316) -> ()  [unwired: 2 in, 2 out]
                  n205 = property on="Search Text" class="Str"("Visible"=w316) -> ()  [unwired: 2 in, 2 out]
                  n206 = local write "Un-used WO's"(w317) -> ()
                  n207 = local write "Converted Data Table"(w320) -> ()
                  n208 = property on="Total Unused" class="DigNum (strict)"("Visible"=w317) -> ()  [unwired: 2 in, 2 out]
                }
                frame 5 {
                  w348 = u16 0 items=["Options", "Sort by Due Date", "Un-Sort", "Show New WO's Only"] ("Options")
                  # "Show new W.O.'s Only"
                  n209 = stacked-sequence {
                    seq-local: [w350 _ _ _] -> [_ w358 _ _]
                    tunnel: w347 -> [w352 w357 _ _]
                    frame #0 {
                      w349 = FALSE ("Visible")
                      # "Read in all used work orders from the worksheets."
                      n210 = Path To String(path=w352) -> (string=w356:string)
                      n211 = Concatenate Strings(w356, "\\Run Worksheets" ("string")) -> (w353:string)
                      n212 = property on="Search Again" class="Bool"("Visible"=w349) -> ()  [unwired: 2 in, 2 out]
                      n213 = property on="Search Text" class="Str"("Visible"=w349) -> ()  [unwired: 2 in, 2 out]
                      n214 = String To Path(string=w353) -> (path=w355:path)
                      n215 = List Folder(path=w355, pattern="* Run Worksheet.txt*") -> (filenames=w350:string[])  [unwired: 2 in, 3 out]
                    }
                    frame #1 {
                      # "Get all W.O.'s from each sheet"
                      n216 = for {
                        tunnel: w358 -> [w363] mode=indexing
                        tunnel: w357 -> [w364]
                        n217 = Path To String(path=w364) -> (string=w367:string)
                        n218 = Concatenate Strings(w367, "\\Run Worksheets\\" ("string"), w363) -> (w366:string)
                        n219 = String To Path(string=w366) -> (path=w360:path)
                        n220 = call-poly <vilib>:"Read Delimited Spreadsheet.vi"("file path (dialog if empty)"=w360) -> ("all rows"=w359:string[][])  [unwired: 9 in, 5 out]
                        n221 = Index Array(array=w359, index (col)=5 ("disabled index (col)")) -> (element=w361:string[])  [unwired: 1 in]
                        n222 = for {
                          tunnel: w361 -> [w368] mode=indexing
                          # "Add used WO's to array"
                          n223 = Not Equal?(x=w368, y="") -> (x != y?=w369:bool)
                          n224 = case shown="True" w369 {
                            tunnel: w368 -> [_ w371]
                            frame False {
                            }
                            frame True {
                              n225 = local read "Used WO's"() -> (w373:string[])
                              n226 = Insert Into Array(array=w373, new element=w371) -> (→"Used WO's":string[])  [unwired: 1 in]
                            }
                          }
                        }
                      }
                    }
                    frame #2 {
                      # "Compare used WO's to Workcenter Report and remove from the Que table"
                      n227 = local read "Used WO's"() -> (w375:string[])
                      n228 = call "Delete Duplicates.vi"("Array In"=w375) -> ("Array w/dup Deleted"=w374:string[])  [unwired: 1 in]
                      n229 = for {
                        tunnel: w374 -> [w385] mode=indexing
                        n230 = local read "Coating Que / CTCL (T)?"() -> (w377:bool)
                        n231 = local read "Converted Data Table"() -> (w380:string[][])
                        n232 = Select(t=1, s=w377, f=3 ("disabled index (col)")) -> (s? t:f=w376:i32)
                        n233 = Index Array(array=w380, index (col)=w376) -> (element=w381:string[])  [unwired: 1 in]
                        n234 = Search 1D Array(1D array=w381, element=w385) -> (index of element=w382:i32)  [unwired: 1 in]
                        n235 = Not Equal?(x=w382, y=-1) -> (x != y?=w384:bool)
                        n236 = case shown="True" w384 {
                          tunnel: w382 -> [_ w391]
                          tunnel: w380 -> [_ w392]
                          tunnel: w376 -> [_ w386]
                          frame False {
                          }
                          frame True {
                            n237 = Increment(x=w391) -> (x+1=w390:i32)
                            n238 = Index Array(array=w392, index (row)=w390, index (col)=w386) -> (element=w389:string)
                            n239 = Equal?(x=w389, y="") -> (x = y?=w387:bool)
                            n240 = stacked-sequence {
                              seq-local: [w393 _ _] -> [_ w398 _]
                              seq-local: [_ w396 _] -> [_ _ w404]
                              tunnel: w392 -> [w395 _ _]
                              tunnel: w391 -> [w394 w397 _]
                              tunnel: w387 -> [_ w399 _]
                              frame #0 {
                                n241 = Delete From Array(array=w395, index (row)=w394) -> (array with subset deleted=w393:string[][])  [unwired: 2 in, 1 out]
                                n242 = local write "Converted Data Table"(w393) -> ()
                              }
                              frame #1 {
                                n243 = case shown="False" w399 {
                                tunnel: w398 -> [_ w403]
                                tunnel: w397 -> [_ w402]
                                tunnel: [w400 w401] -> w396
                                frame False {
                                n244 = local read "Converted Data Table"() -> (w400:string[][])
                                }
                                frame True {
                                # "Delete second row"
                                n245 = Delete From Array(array=w403, index (row)=w402) -> (array with subset deleted=w401:string[][])  [unwired: 2 in, 1 out]
                                }
                                }
                              }
                              frame #2 {
                                n246 = local write "Converted Data Table"(w404) -> ()
                              }
                            }
                          }
                        }
                      }
                      n247 = local write "Used WO's"(w374) -> ()
                    }
                    frame #3 {
                      w412 = TRUE ("Un-used WO's")
                      n248 = local read "Coating Que / CTCL (T)?"() -> (w408:bool)
                      n249 = local read "Converted Data Table"() -> (w411:string[][])
                      n250 = Select(t=1, s=w408, f=3 ("disabled index (col)")) -> (s? t:f=w405:i32)
                      n251 = Index Array(array=w411, index (col)=w405) -> (element=w410:string[])  [unwired: 1 in]
                      n252 = for {
                        tunnel: w410 -> [w415] mode=indexing
                        n253 = Not Equal?(x=w415, y="") -> (x != y?=w413:bool)
                        n254 = case shown="True" w413 {
                          frame False {
                          }
                          frame True {
                            n255 = local read "Total Unused"() -> (w417:i32)
                            n256 = Increment(x=w417) -> (x+1=→"Total Unused":i32)
                          }
                        }
                      }
                      n257 = local write "Total Unused"(0 ("Total Unused")) -> ()
                      n258 = property on="Total Unused" class="DigNum (strict)"("Visible"=w412) -> ()  [unwired: 2 in, 2 out]
                      "Un-used WO's" <- w412
                    }
                  }
                  n259 = local write "Options"(w348) -> ()
                }
                frame 6 {
                  # "Search"
                  n260 = property on="Search Text" class="Str"("Visible"=TRUE) -> ()  [unwired: 2 in, 2 out]
                  n261 = Equal?(x=w419, y="") -> (x = y?=w421:bool)
                  n262 = case shown="False" w421 {
                    tunnel: w423 -> [w429 _]
                    tunnel: w419 -> [w428 _]
                    tunnel: [u16 0 ("Options") u16 6 ("Options")] -> w420
                    frame False {
                      n263 = call "Search Table for Text 2.vi"("Search Table"=w429, "Search Text"=w428, "Search Ctrl"=TRUE) -> ("Row Found"=w426:i32, "Text Found"=w424:bool)  [unwired: 2 out]
                      n264 = case shown="False" w424 {
                        frame False {
                          n265 = One Button Dialog(message="Part Number not Found...") -> ()  [unwired: 1 in, 1 out]
                        }
                        frame True {
                        }
                      }
                      n266 = property on="Search Again" class="Bool"("Visible"=w424) -> ()  [unwired: 2 in, 2 out]
                      n267 = Bundle("Row Found"=w426, "Row Found"=0) -> (w431:cluster{"Row Found":i32, "Row Found":i32})  [unwired: 1 in]
                      n268 = property on="Converted Data Table" class="Tbl (strict)"("Index Values"=w431) -> ()  [unwired: 2 in, 2 out]
                    }
                    frame True {
                    }
                  }
                  n269 = local write "Options"(w420) -> ()
                }
              }
            }
          }
          frame True {
            # "Apply Data to Run Worksheet"
            n270 = stacked-sequence {
              seq-local: [_ w459 _] -> [_ _ w754]
              seq-local: [_ w464 _] -> [_ _ w752]
              seq-local: [_ w457 _] -> [_ _ w751]
              seq-local: [w438 _ _] -> [_ w444 w750]
              tunnel: w436 -> [_ w462 w755]
              tunnel: w435 -> [_ _ w753]
              tunnel: w434 -> [w437 w463 _]
              frame #0 {
                # "Read in Design Info Table"
                n271 = Path To String(path=w437) -> (string=w441:string)
                n272 = Concatenate Strings(w441, "\\" ("string"), "Design Info.txt" ("string")) -> (w442:string)
                n273 = String To Path(string=w442) -> (path=w443:path)
                n274 = call-poly <vilib>:"Read Delimited Spreadsheet.vi"("file path (dialog if empty)"=w443) -> ("all rows"=w438:string[][])  [unwired: 9 in, 5 out]
              }
              frame #1 {
                w451 = TRUE ("replace all? (F)")
                # "Lookup Part # to get info from it."
                n275 = local read "Coating Que / CTCL (T)?"() -> (w457:bool)
                n276 = local read "Edit Position"() -> (w461:T1)
                n277 = Unbundle(w461) -> ("Row"=w459:i32)  [unwired: 1 out]
                n278 = case shown="True" w457 {
                  tunnel: [w477 w482] -> w455
                  tunnel: w462 -> [w476 w483]
                  tunnel: [w474 w481] -> w450
                  tunnel: w459 -> [w473 w479]
                  tunnel: [w471 w480] -> w448
                  frame False {
                    n279 = Index Array(array=w476, index (row) #1=w473, index (col) #1=6 ("disabled index (col)"), index (row) #2=w473, index (col) #2=3 ("disabled index (col)"), index (row) #3=w473, index (col) #3=5 ("disabled index (col)")) -> (element #1=w477:string, element #2=w474:string, element #3=w471:string)
                  }
                  frame True {
                    n280 = Index Array(array=w483, index (row) #1=w479, index (col) #1=3 ("disabled index (col)"), index (row) #2=w479, index (col) #2=1 ("disabled index (col)"), index (row) #3=w479, index (col) #3=7 ("disabled index (col)")) -> (element #1=w482:string, element #2=w481:string, element #3=w480:string)
                  }
                }
                n281 = Path To String(path=w463) -> (string=w470:string)
                n282 = Concatenate Strings(w470, "\\Part Number Info.txt" ("string")) -> (w468:string)
                n283 = Search and Replace String(replace all?=w451, input string=w455, search string=" ") -> (result string=w456:string)  [unwired: 5 in, 3 out]
                "Part Number" <- w456
                n284 = String To Path(string=w468) -> (path=w446:path)
                n285 = call-poly <vilib>:"Read Delimited Spreadsheet.vi"("file path (dialog if empty)"=w446) -> ("all rows"=w445:string[][])  [unwired: 9 in, 5 out]
                n286 = Search and Replace String(replace all?=w451, input string=w450, search string=" ") -> (result string=→"Work Order":string)  [unwired: 5 in, 3 out]
                n287 = Index Array(array=w445, index (col)=0 ("disabled index (col)")) -> (element=w460:string[])  [unwired: 1 in]
                n288 = Search and Replace String(replace all?=w451, input string=w448, search string=" ") -> (result string=→"Qty":string)  [unwired: 5 in, 3 out]
                n289 = Search 1D Array(1D array=w460, element=w456) -> (index of element=w465:i32)  [unwired: 1 in]
                n290 = Not Equal?(x=w465, y=-1) -> (x != y?=w464:bool)
                n291 = case shown="False" w464 {
                  tunnel: w465 -> [_ w489]
                  tunnel: w463 -> [_ w496]
                  tunnel: w445 -> [_ w495]
                  tunnel: w456 -> [_ w494]
                  tunnel: w444 -> [_ w493]
                  tunnel: w462 -> [_ w492]
                  tunnel: w459 -> [_ w491]
                  tunnel: w460 -> [_ w490]
                  tunnel: w457 -> [_ w488]
                  frame False {
                    n292 = One Button Dialog(message="The Part Number was not found in the Part Number Info table and not added to the current worksheet...") -> ()  [unwired: 1 in, 1 out]
                  }
                  frame True {
                    # "Part Number Found"
                    n293 = stacked-sequence {
                      seq-local: [_ _ _ w709 _ _] -> [_ _ _ _ w725 _]
                      seq-local: [_ _ w689 _ _ _] -> [_ _ _ _ _ _]
                      seq-local: [_ _ w691 _ _ _] -> [_ _ _ w704 _ _]
                      seq-local: [_ _ w690 _ _ _] -> [_ _ _ w707 _ _]
                      seq-local: [w501 _ _ _ _ _] -> [_ w541 _ _ _ _]
                      seq-local: [_ w540 _ _ _ _] -> [_ _ w686 w701 w717 _]
                      seq-local: [w504 _ _ _ _ _] -> [_ w538 _ _ _ _]
                      seq-local: [w500 _ _ _ _ _] -> [_ w528 _ _ _ _]
                      seq-local: [_ w527 _ _ _ _] -> [_ _ _ _ w713 _]
                      tunnel: w496 -> [_ _ _ _ _ _]
                      tunnel: w495 -> [w508 _ w700 w708 w720 _]
                      tunnel: w494 -> [w506 _ _ _ _ _]
                      tunnel: w493 -> [_ _ w699 _ _ _]
                      tunnel: w492 -> [_ _ _ _ w726 _]
                      tunnel: w491 -> [_ _ _ _ w721 _]
                      tunnel: w490 -> [w507 _ _ _ _ _]
                      tunnel: w489 -> [_ w539 _ _ _ _]
                      tunnel: w488 -> [_ _ _ _ w718 _]
                      frame #0 {
                        w505 = 0 ("Index")
                        # "Row #\nSide #'\nDesign #\nSys #"
                        # "Get all matching part numbers, side #'s, design numbers, and sys #'s"
                        n294 = property on="System Select" class="Ring (strict)"() -> ("RingText.Text"=w500:string)  [unwired: 2 in, 2 out]
                        n295 = local write "Index"(w505) -> ()
                        n296 = while {
                          tunnel: w508 -> [w525]
                          tunnel: w507 -> [w524]
                          tunnel: w506 -> [w523]
                          tunnel: [w512] -> w499 mode=indexing
                          tunnel: [w515] -> w504 mode=indexing
                          tunnel: w505 -> [_]
                          tunnel: w500 -> [w511]
                          tunnel: [w510] -> w503 mode=indexing
                          stop <- w520 stop-if-true
                          n297 = local read "Index"() -> (w521:i32)
                          n298 = Search 1D Array(1D array=w524, element=w523, start index (0)=w521) -> (index of element=w513:i32)
                          n299 = Increment(x=w513) -> (x+1=→"Index":i32)
                          n300 = Equal?(x=w513, y=-1) -> (x = y?=w520:bool)
                          n301 = Index Array(array=w525, index (row) #1=w513, index (col) #1=6 ("disabled index (col)"), index (row) #2=w513, index (col) #2=3 ("index (col)"), index (row) #3=w513, index (col) #3=1 ("disabled index (col)")) -> (element #1=w512:string, element #2=w516:string, element #3=w517:string)
                          n302 = Number To Decimal String(number=w513) -> (decimal integer string=w509:string)  [unwired: 1 in]
                          n303 = Build Array(w509, w517, w516, w512) -> (w515:string[])
                          n304 = Equal?(x=w512, y=w511) -> (x = y?=w510:bool)
                        }
                        n305 = Delete From Array(array=w499, length=1) -> (array with subset deleted=w498:string[])  [unwired: 1 in, 1 out]
                        n306 = Boolean Array To Number(Boolean array=w503) -> (number=w502:u32)
                        n307 = Greater Than 0?(x=w502) -> (x > 0?=w501:bool)
                        n308 = property on="Select System" class="Ring (strict)"("Strings []"=w498) -> ()  [unwired: 2 in, 2 out]
                      }
                      frame #1 {
                        w531 = string[] [] ("S1 Design # and row")
                        # "Row #"
                        # "Row #\nSide #\nDesign #\nSys #"
                        n309 = local write "S2 Design # and row"(w531) -> ()
                        n310 = local write "S1 Design # and row"(w531) -> ()
                        n311 = Index Array(array=w538, index (col) #1=0 ("disabled index (col)"), index (col) #2=1 ("index (col)"), index (col) #3=2 ("disabled index (col)"), index (col) #4=3 ("index (col)")) -> (element #1=w536:string[], element #2=w532:string[], element #3=w533:string[], element #4=w529:string[])  [unwired: 4 in]
                        n312 = case shown="True" w541 {
                          tunnel: w533 -> [w547 w603]
                          tunnel: [w546 w601] -> w540
                          tunnel: w539 -> [w545 _]
                          tunnel: w536 -> [w544 w602]
                          tunnel: w532 -> [w542 w604]
                          tunnel: w531 -> [_ _]
                          tunnel: w529 -> [_ w600]
                          tunnel: w528 -> [_ w599]
                          tunnel: [w543 w598] -> w527
                          frame False {
                            # "Part number found but used in another system"
                            n313 = stacked-sequence {
                              seq-local: [_ _ w567 _ _] -> [_ _ _ _ w588]
                              seq-local: [w549 _ _ _ _] -> [_ _ w563 _ _]
                              seq-local: [w548 _ _ _ _] -> [_ _ w562 _ _]
                              tunnel: w547 -> [w558 _ w566 _ _]
                              tunnel: [_ _ _ _ w587] -> w546
                              tunnel: w545 -> [_ _ _ _ w586]
                              tunnel: w544 -> [_ _ _ _ w585]
                              tunnel: [_ _ w565 _ _] -> w543
                              tunnel: w542 -> [_ _ w564 _ _]
                              frame #0 {
                                w548 = "\nWorksheet" ("string")
                                w549 = "Put in Sys " ("Boolean Text.Text")
                                # "Initialize cluster indicators"
                                n314 = Index Array(array=w558) -> (element=w557:string)  [unwired: 1 in]
                                n315 = Bundle By Name(cluster="System Cluster 2", "Select System"=u16 0, "Design #"=w557, "OK Button"=FALSE, "Cancel"=FALSE, "Side#"="") -> (w555:T3)
                                n316 = property on="System Select" class="Ring (strict)"() -> ("RingText.Text"=w551:string)  [unwired: 2 in, 2 out]
                                n317 = local write "System Cluster 2"(w555) -> ()
                                n318 = Concatenate Strings(w549, w551, w548) -> (w550:string)
                                n319 = property on="Cancel" class="Bool (strict)"("BoolText.Text"=w550) -> ()  [unwired: 2 in, 2 out]
                              }
                              frame #1 {
                                # "Show cluster on Run Worksheet"
                                n320 = property on="System Cluster 2" class="Clust (strict)"("Visible"=TRUE) -> ()  [unwired: 2 in, 2 out]
                                n321 = local write "Tab Control"(enum32{"Workcenter Report", "Run Worksheet"}."Run Worksheet" ("Tab Control")) -> ()
                              }
                              frame #2 {
                                # "Wait for User"
                                n322 = while {
                                tunnel: [w578] -> w567
                                tunnel: w566 -> [w581]
                                tunnel: [w575] -> w565
                                tunnel: w564 -> [w574]
                                tunnel: w563 -> [w571]
                                tunnel: w562 -> [w570]
                                stop <- w582 stop-if-true
                                n323 = local read "System Cluster 2"() -> (w576:T3)
                                n324 = Unbundle By Name(w576) -> ("Select System"=w573:u16)
                                n325 = Index Array(array=w574, index=w573) -> (element=w572:string)
                                n326 = Wait (ms)(milliseconds to wait=u32 100) -> ()  [unwired: 1 out]
                                n327 = Index Array(array=w581, index=w573) -> (element=w580:string)
                                n328 = property on="Select System" class="Ring (strict)"() -> ("RingText.Text"=w569:string)  [unwired: 2 in, 2 out]
                                n329 = Bundle By Name(cluster=w576, "Side#"=w572, "Design #"=w580) -> (w577:T3)
                                n330 = Unbundle By Name(w577) -> ("OK Button"=w578:bool, "Cancel"=w579:bool, "Side#"=w575:string)
                                n331 = Concatenate Strings(w571, w569, w570) -> (w568:string)
                                n332 = local write "System Cluster 2"(w577) -> ()
                                n333 = property on="OK Button" class="Bool (strict)"("BoolText.Text"=w568) -> ()  [unwired: 2 in, 2 out]
                                n334 = Or(x=w578, y=w579) -> (x .or. y?=w582:bool)
                                }
                              }
                              frame #3 {
                                n335 = property on="System Cluster 2" class="Clust (strict)"("Visible"=FALSE) -> ()  [unwired: 2 in, 2 out]
                              }
                              frame #4 {
                                n336 = case shown="True" w588 {
                                tunnel: [w589 w595] -> w587
                                tunnel: w586 -> [w589 _]
                                tunnel: w585 -> [_ w591]
                                frame False {
                                # "User Cancelled"
                                }
                                frame True {
                                # "Row #"
                                # "Use selected design number"
                                n337 = local read "System Cluster 2"() -> (w597:T3)
                                n338 = property on="System Select" class="Ring (strict)"() -> ("Strings []"=w593:string[])  [unwired: 2 in, 2 out]
                                n339 = Decimal String To Number(string=w591) -> (number=w590:i32[])  [unwired: 2 in, 1 out]
                                n340 = property on="Select System" class="Ring (strict)"() -> ("RingText.Text"=w594:string)  [unwired: 2 in, 2 out]
                                n341 = Unbundle By Name(w597) -> ("Select System"=w596:u16)
                                n342 = Search 1D Array(1D array=w593, element=w594) -> (index of element=w592:i32)  [unwired: 1 in]
                                n343 = Index Array(array=w590, index=w596) -> (element=w595:i32)
                                n344 = local write "System Select"(w592) -> ()
                                }
                                }
                              }
                            }
                          }
                          frame True {
                            # "Part number found for current system selected, prompt user for Side # if S1 and S2 found with different design numbers."
                            n345 = stacked-sequence {
                              seq-local: [w608 _ _ _] -> [_ w635 _ _]
                              seq-local: [_ w633 _ _] -> [_ _ w647 w655]
                              seq-local: [_ _ w646 _] -> [_ _ _ w654]
                              tunnel: w604 -> [w610 _ _ _]
                              tunnel: w603 -> [w609 _ _ _]
                              tunnel: w602 -> [w607 _ _ _]
                              tunnel: [_ _ _ w653] -> w601
                              tunnel: w600 -> [w606 _ _ _]
                              tunnel: w599 -> [w605 _ _ _]
                              tunnel: [_ _ _ w652] -> w598
                              frame #0 {
                                n346 = for {
                                tunnel: w610 -> [w626] mode=indexing
                                tunnel: w609 -> [w621] mode=indexing
                                tunnel: [w620] -> w608 mode=indexing
                                tunnel: w607 -> [w619] mode=indexing
                                tunnel: w606 -> [w617] mode=indexing
                                tunnel: w605 -> [w616]
                                w618 = "S2" ("regular expression")
                                w624 = "S1" ("regular expression")
                                n347 = Equal?(x=w617, y=w616) -> (x = y?=w613:bool)
                                n348 = Match Pattern(string=w626, regular expression=w624) -> (match substring=w625:string)  [unwired: 1 in, 3 out]
                                n349 = Match Pattern(string=w626, regular expression=w618) -> (match substring=w623:string)  [unwired: 1 in, 3 out]
                                n350 = Equal?(x=w623, y=w618) -> (x = y?=w614:bool)
                                n351 = Equal?(x=w625, y=w624) -> (x = y?=w615:bool)
                                n352 = And(x=w614, y=w613) -> (x .and. y?=w612:bool)
                                n353 = And(x=w615, y=w613) -> (x .and. y?=w611:bool)
                                n354 = Build Array(w611, w612) -> (w622:bool[])
                                n355 = Boolean Array To Number(Boolean array=w622) -> (number=w620:u32)
                                n356 = case shown="0, Default" w620 {
                                tunnel: w621 -> [_ w628 w631]
                                tunnel: w619 -> [_ w627 w630]
                                frame 0, Default {
                                }
                                frame 1 {
                                # "Side 1 found, save design #"
                                n357 = Build Array(w628, w627) -> (→"S1 Design # and row":string[])
                                }
                                frame 2 {
                                # "Side 2 found, save design #"
                                n358 = Build Array(w631, w630) -> (→"S2 Design # and row":string[])
                                }
                                }
                                }
                              }
                              frame #1 {
                                n359 = Add Array Elements(numeric array=w635) -> (sum=w634:u32)
                                n360 = case shown="0, Default" w634 {
                                tunnel: [_ w641] -> w633
                                frame 0, Default {
                                # "Only one design and side #"
                                }
                                frame 3 {
                                w638 = 0 ("index")
                                w642 = ""
                                # "S1 and S2 found, compare design numbers"
                                n361 = local read "S1 Design # and row"() -> (w640:string[])
                                n362 = local read "S2 Design # and row"() -> (w639:string[])
                                n363 = Index Array(array=w640, index=w638) -> (element=w637:string)
                                n364 = Index Array(array=w639, index=w638) -> (element=w636:string)
                                n365 = Not Equal?(x=w637, y=w636) -> (x != y?=w645:bool)
                                n366 = Not Equal?(x=w637, y=w642) -> (x != y?=w644:bool)
                                n367 = Not Equal?(x=w636, y=w642) -> (x != y?=w643:bool)
                                n368 = Compound Arithmetic op=AND(w645, w644, w643) -> (w641:bool)
                                }
                                }
                              }
                              frame #2 {
                                n369 = case shown="True" w647 {
                                tunnel: [_ w648] -> w646
                                frame False {
                                # "Only one design and side #"
                                }
                                frame True {
                                n370 = Two Button Dialog(message="The part number found has different design numbers for S1 and S2.  Please select the side number to use for this run build.  If this part number should have the same design number for side 1 and 2, please fix in the part number info table...", 1:"SIDE 2" ("F button name (\"Cancel\")"), 2:"SIDE 1" ("T button name (\"OK\")")) -> (T button?=w648:bool)
                                }
                                }
                              }
                              frame #3 {
                                n371 = case shown="False" w655 {
                                tunnel: w654 -> [_ w680]
                                tunnel: [w666 w676] -> w653
                                tunnel: [w656 w675] -> w652
                                frame False {
                                w663 = ""
                                # "Get row of one of them not blank"
                                n372 = local read "S2 Design # and row"() -> (w664:string[])
                                n373 = local read "S1 Design # and row"() -> (w667:string[])
                                n374 = Index Array(array=w667, index=1) -> (element=w658:string)
                                n375 = Index Array(array=w664, index=1) -> (element=w657:string)
                                n376 = Not Equal?(x=w658, y=w663) -> (x != y?=w661:bool)
                                n377 = Not Equal?(x=w657, y=w663) -> (x != y?=w662:bool)
                                n378 = Build Array(w661, w662) -> (w659:bool[])
                                n379 = Boolean Array To Number(Boolean array=w659) -> (number=w660:u32)
                                n380 = case shown="1, Default" w660 {
                                tunnel: [w671 w674] -> w666
                                tunnel: w658 -> [w670 _]
                                tunnel: w657 -> [_ w673]
                                tunnel: ["S1" ("element") "S2" ("element")] -> w656
                                frame 1, Default {
                                n381 = Decimal String To Number(string=w670) -> (number=w671:i32)  [unwired: 2 in, 1 out]
                                }
                                frame 2 {
                                n382 = Decimal String To Number(string=w673) -> (number=w674:i32)  [unwired: 2 in, 1 out]
                                }
                                }
                                }
                                frame True {
                                # "User selected S1 or S2"
                                n383 = case shown="False" w680 {
                                tunnel: [w682 w684] -> w677
                                tunnel: ["S2" ("element") "S1" ("element")] -> w675
                                frame False {
                                # "S2"
                                n384 = local read "S2 Design # and row"() -> (w682:string[])
                                }
                                frame True {
                                # "S1"
                                n385 = local read "S1 Design # and row"() -> (w684:string[])
                                }
                                }
                                n386 = Index Array(array=w677, index=1) -> (element=w678:string)
                                n387 = Decimal String To Number(string=w678) -> (number=w676:i32)  [unwired: 2 in, 1 out]
                                }
                                }
                              }
                            }
                          }
                        }
                      }
                      frame #2 {
                        # "Design Number"
                        # "Lookup Coating type and wavelength"
                        n388 = Index Array(array=w699, index (col)=3 ("disabled index (col)")) -> (element=w697:string[])  [unwired: 1 in]
                        n389 = Index Array(array=w700, index (row) #1=w686, index (col) #1=3 ("f"), index (row) #2=w686, index (col) #2=6 ("disabled index (col)")) -> (element #1=w696:string, element #2=→"System No.":string)
                        n390 = To Upper Case(1:w696) -> (0:w694:string)
                        n391 = To Upper Case(1:w697) -> (0:w695:string[])
                        n392 = Search 1D Array(1D array=w695, element=w694) -> (index of element=w689:i32)  [unwired: 1 in]
                        n393 = Index Array(array=w699, index (row) #1=w689, index (col) #1=0 ("disabled index (col)"), index (row) #2=w689, index (col) #2=2 ("disabled index (col)")) -> (element #1=w691:string, element #2=w690:string)
                        "Part info Row" <- w686
                      }
                      frame #3 {
                        # "Build transfer array part 1"
                        n394 = Index Array(array=w708, index (row) #1=w701, index (col) #1=3 ("disabled index (col)"), index (row) #2=w701, index (col) #2=4 ("index (col)"), index (row) #3=w701, index (col) #3=5 ("index (col)")) -> (element #1=w703:string, element #2=w705:string, element #3=w702:string)
                        "Design No." <- w703
                        n395 = local write "Diameter"(w702) -> ()
                        n396 = local write "Wavelength 2"(w707) -> ()
                        n397 = local write "Coating Type 2"(w704) -> ()
                        n398 = local write "Substrate 2"(w705) -> ()
                        n399 = Build Array(w705, w704, w707, w703, w702) -> (w709:string[])
                      }
                      frame #4 {
                        # "Opr. Start Date"
                        # "Due Date"
                        # "Side #"
                        # "Engineering notes from Part Info"
                        # "Qty"
                        # "Apply to Worksheet"
                        # "Part Number"
                        # "W.O. #"
                        n400 = case shown="True" w718 {
                          tunnel: w726 -> [w736 w745]
                          tunnel: [w734 w744] -> w724
                          tunnel: [w732 w743] -> w723
                          tunnel: [w730 w742] -> w722
                          tunnel: w721 -> [w729 w739]
                          tunnel: [w728 w740] -> w716
                          tunnel: [w728 w737] -> w712
                          frame False {
                            w728 = ""
                            n401 = Index Array(array=w736, index (row) #1=w729, index (col) #1=3 ("disabled index (col)"), index (row) #2=w729, index (col) #2=6 ("disabled index (col)"), index (row) #3=w729, index (col) #3=5 ("disabled index (col)")) -> (element #1=w734:string, element #2=w732:string, element #3=w730:string)
                          }
                          frame True {
                            n402 = Index Array(array=w745, index (row) #1=w739, index (col) #1=1 ("disabled index (col)"), index (row) #2=w739, index (col) #2=3 ("disabled index (col)"), index (row) #3=w739, index (col) #3=7 ("disabled index (col)"), index (row) #4=w739, index (col) #4=8 ("index (col)"), index (row) #5=w739, index (col) #5=0 ("disabled index (col)")) -> (element #1=w744:string, element #2=w743:string, element #3=w742:string, element #4=w740:string, element #5=w737:string)
                          }
                        }
                        n403 = Index Array(array=w720, index (row)=w717, index (col)=7 ("disabled index (col)")) -> (element=w715:string)
                        n404 = Build Array (concatenate)(w725, w724, w723, w722, w713, w715, "", w716, w712) -> (→"Worksheet array":string[])
                      }
                      frame #5 {
                        w749 = TRUE ("Add to Worksheet")
                        n405 = local write "Add to Worksheet"(w749) -> ()
                        n406 = local write "Lookup was True"(w749) -> ()
                        "Part No Found" <- w749
                      }
                    }
                  }
                }
                n407 = local write "Part No Found"(FALSE ("Part No Found")) -> ()
              }
              frame #2 {
                n408 = case shown="False" w752 {
                  tunnel: w755 -> [w760 w1119]
                  tunnel: w754 -> [w759 w1121]
                  tunnel: w753 -> [w758 _]
                  tunnel: w750 -> [w757 _]
                  tunnel: w751 -> [w756 _]
                  frame False {
                    # "Part Number Not Found on Disk"
                    n409 = stacked-sequence {
                      seq-local: [w773 _ _ _ _ _ _ _ _ _] -> [_ w858 _ _ _ _ _ _ _ _]
                      seq-local: [w762 _ _ _ _ _ _ _ _ _] -> [_ w859 _ _ _ _ _ _ _ _]
                      seq-local: [_ _ _ _ _ _ w1046 _ _ _] -> [_ _ _ _ _ _ _ w1071 _ _]
                      seq-local: [w769 _ _ _ _ _ _ _ _ _] -> [_ _ w955 _ w1021 _ _ _ _ _]
                      seq-local: [_ _ _ _ _ w1038 _ _ _ _] -> [_ _ _ _ _ _ w1045 _ _ _]
                      seq-local: [_ _ _ _ _ w1041 _ _ _ _] -> [_ _ _ _ _ _ _ w1068 _ _]
                      seq-local: [_ _ w953 _ _ _ _ _ _ _] -> [_ _ _ w963 _ _ _ _ _ _]
                      seq-local: [_ _ w952 _ _ _ _ _ _ _] -> [_ _ _ w962 _ _ _ _ _ _]
                      tunnel: w759 -> [w770 _ _ _ _ _ _ _ _ _]
                      tunnel: w760 -> [w772 _ _ _ _ _ _ _ _ _]
                      tunnel: w758 -> [_ _ _ _ _ _ _ _ _ _]
                      tunnel: w757 -> [_ _ _ w965 _ _ _ _ _ _]
                      tunnel: w756 -> [w768 _ w948 _ _ _ _ _ w1082 _]
                      frame #0 {
                        w765 = "\"" ("regular expression")
                        # "Coating type"
                        # "get Coating Type and Substrate"
                        n410 = property on="Substrate" class="Ring (strict)"() -> ("Strings []"=w780:string[])  [unwired: 2 in, 2 out]
                        n411 = To Upper Case(1:w780) -> (0:w774:string[])
                        n412 = case shown="True" w768 {
                          tunnel: [w781 w793] -> w779
                          tunnel: w772 -> [w784 w789]
                          tunnel: [w781 w788] -> w771
                          tunnel: w770 -> [w783 w787]
                          tunnel: [w782 w786] -> w762
                          frame True {
                            w781 = ""
                            n413 = Index Array(array=w784, index (row)=w783, index (col)=4 ("disabled index (col)")) -> (element=w782:string)
                          }
                          frame False {
                            n414 = Index Array(array=w789, index (row) #1=w787, index (col) #1=7 ("disabled index (col)"), index (row) #2=w787, index (col) #2=0 ("disabled index (col)"), index (row) #3=w787, index (col) #3=2 ("disabled index (col)")) -> (element #1=w786:string, element #2=w788:string, element #3=w793:string)
                          }
                        }
                        "Part Description" <- w762
                        n415 = To Upper Case(1:w762) -> (0:w767:string)
                        n416 = To Upper Case(1:w771) -> (0:w769:string)
                        n417 = Match Pattern(string=w767, regular expression=w765) -> (before substring=w764:string, match substring=w766:string)  [unwired: 1 in, 2 out]
                        n418 = Equal?(x=w766, y=w765) -> (x = y?=w763:bool)
                        n419 = Select(t=w764, s=w763, f=w762) -> (s? t:f=w761:string)
                        n420 = stacked-sequence {
                          seq-local: [_ w810 _ _] -> [_ _ w823 _]
                          seq-local: [_ _ w822 _] -> [_ _ _ w830]
                          seq-local: [_ w809 _ _] -> [_ _ w817 w829]
                          tunnel: w761 -> [w795 _ _ _]
                          tunnel: w774 -> [_ w812 _ w831]
                          frame #0 {
                            # "Check for non-substrate text."
                            n421 = for {
                              tunnel: w795 -> [w797]
                              tunnel: string[] ["RWK ", "REWORK ", "RWK CS ", "REWORK CS ", "DT CS "] ("Array") -> [w800] mode=indexing
                              n422 = Match Pattern(string=w797, regular expression=w800) -> (match substring=w801:string, after substring=w798:string)  [unwired: 1 in, 2 out]
                              n423 = Equal?(x=w801, y=w800) -> (x = y?=w799:bool)
                              n424 = case shown="False" w799 {
                                tunnel: w798 -> [_ w806]
                                tunnel: w797 -> [w802 _]
                                frame False {
                                n425 = local write "Substrate Text"(w802) -> ()
                                }
                                frame True {
                                w805 = "CS" ("regular expression")
                                n426 = Match Pattern(string=w806, regular expression=w805) -> (match substring=w807:string, after substring=w803:string)  [unwired: 1 in, 2 out]
                                n427 = Equal?(x=w807, y=w805) -> (x = y?=w804:bool)
                                n428 = case shown="True" w804 {
                                tunnel: w803 -> [_ w808]
                                frame False {
                                }
                                frame True {
                                "Substrate Text" <- w808
                                }
                                }
                                }
                              }
                            }
                            "Substrate 2" <- ""
                          }
                          frame #1 {
                            # "Match Substrate.  If Exact match use that, if not check if partial match"
                            n429 = local read "Substrate Text"() -> (w809:string)
                            n430 = Search 1D Array(1D array=w812, element=w809) -> (index of element=w811:i32)  [unwired: 1 in]
                            n431 = Not Equal?(x=w811, y=-1) -> (x != y?=w810:bool)
                            n432 = case shown="False" w810 {
                              tunnel: w812 -> [_ w816]
                              tunnel: w811 -> [_ w815]
                              frame False {
                              }
                              frame True {
                                n433 = Index Array(array=w816, index=w815) -> (element=w814:string)
                                n434 = local write "Substrate 2"(w814) -> ()
                              }
                            }
                          }
                          frame #2 {
                            # "Check for 2 part substrate"
                            n435 = for {
                              tunnel: string[] ["ALUMINUM TUBES", ".55IN. QUARTZ CRYSTALS", "ZNS (MULTISPECTRAL)", "ZNS (CLEARTRAN)", "FUSED SILICA", "GAAS WAFER", "GE DOUBLETS", "GE WAFERS", "KBR (SALT)", "SI OG"] -> [w825] mode=indexing
                              tunnel: w817 -> [w826]
                              tunnel: [w824] -> w820 mode=indexing
                              n436 = Match Pattern(string=w826, regular expression=w825) -> (match substring=w827:string)  [unwired: 1 in, 3 out]
                              n437 = Equal?(x=w827, y=w825) -> (x = y?=w824:bool)
                              n438 = case shown="False" w824 {
                                tunnel: w825 -> [_ w828]
                                frame False {
                                }
                                frame True {
                                n439 = local write "Substrate 2"(w828) -> ()
                                }
                              }
                            }
                            n440 = Boolean Array To Number(Boolean array=w820) -> (number=w819:u32)
                            n441 = Greater Than 0?(x=w819) -> (x > 0?=w818:bool)
                            n442 = Or(x=w818, y=w823) -> (x .or. y?=w822:bool)
                          }
                          frame #3 {
                            n443 = case shown="False" w830 {
                              tunnel: w831 -> [w832 _]
                              tunnel: w829 -> [w833 _]
                              frame False {
                                # "Match Substrate Partial"
                                n444 = for {
                                tunnel: w833 -> [w838]
                                tunnel: w832 -> [w835] mode=indexing
                                n445 = Search/Split String(string=w838, search string/char (-)=w835) -> (match + rest of string=w836:string)  [unwired: 1 in, 2 out]
                                n446 = Not Equal?(x=w836, y="") -> (x != y?=w837:bool)
                                n447 = case shown="True" w837 {
                                tunnel: w836 -> [_ w852]
                                frame False {
                                }
                                frame True {
                                w847 = "(" ("regular expression")
                                w849 = "/" ("regular expression")
                                n448 = Match Pattern(string=w852, regular expression=" ") -> (before substring=w842:string)  [unwired: 1 in, 3 out]
                                n449 = Match Pattern(string=w842, regular expression=w849) -> (before substring=w841:string, match substring=w850:string)  [unwired: 1 in, 2 out]
                                n450 = Match Pattern(string=w842, regular expression=w847) -> (before substring=w840:string, match substring=w848:string)  [unwired: 1 in, 2 out]
                                n451 = Equal?(x=w850, y=w849) -> (x = y?=w845:bool)
                                n452 = Equal?(x=w848, y=w847) -> (x = y?=w846:bool)
                                n453 = Build Array(w845, w846) -> (w844:bool[])
                                n454 = Boolean Array To Number(Boolean array=w844) -> (number=w843:u32)
                                n455 = case shown="0, Default" w843 {
                                tunnel: w842 -> [w853 _ _]
                                tunnel: w841 -> [_ w854 _]
                                tunnel: w840 -> [_ _ w855]
                                tunnel: [w853 w854 w855] -> w839
                                frame 0, Default {
                                }
                                frame 1 {
                                }
                                frame 2 {
                                }
                                }
                                n456 = local write "Substrate 2"(w839) -> ()
                                }
                                }
                                }
                              }
                              frame True {
                              }
                            }
                          }
                        }
                        n457 = Equal?(x=w779, y="") -> (x = y?=w777:bool)
                        n458 = Equal?(x=w779, y="*") -> (x = y?=w778:bool)
                        n459 = Or(x=w777, y=w778) -> (x .or. y?=w773:bool)
                        n460 = case shown="False" w773 {
                          tunnel: w779 -> [w856 _]
                          frame False {
                            n461 = local write "Wavelength 2"(w856) -> ()
                          }
                          frame True {
                          }
                        }
                      }
                      frame #1 {
                        w867 = "DIA " ("regular expression")
                        # "Get Diameter and Wavelength"
                        n462 = To Upper Case(1:w859) -> (0:w860:string)
                        n463 = Match Pattern(string=w860, regular expression=w867) -> (before substring=w862:string, match substring=w866:string, after substring=w857:string)  [unwired: 1 in, 1 out]
                        n464 = case shown="True" w858 {
                          tunnel: w857 -> [_ w886]
                          frame False {
                            # "Wavelength found in column 2 remove extra zeros if found"
                            n465 = local read "Wavelength 2"() -> (w870:string)
                            n466 = String Length(string=w870) -> (length=w871:i32)
                            n467 = while {
                              shift-right: [w873] -> _
                              shift-left: w871 -> [w874]
                              stop <- w876 continue-if-true
                              n468 = local read "Wavelength 2"() -> (w872:string)
                              n469 = Reverse String(1:w872) -> (0:w875:string)
                              n470 = String Subset(string=w875, offset (0)=0, length (rest)=1 ("length (rest)")) -> (substring=w877:string)
                              n471 = Equal?(x=w877, y="0") -> (x = y?=w876:bool)
                              n472 = case shown="False" w876 {
                                tunnel: w874 -> [w881 w884]
                                tunnel: [w881 w883] -> w873
                                frame False {
                                }
                                frame True {
                                n473 = local read "Wavelength 2"() -> (w885:string)
                                n474 = Decrement(x=w884) -> (x-1=w883:i32)
                                n475 = String Subset(string=w885, length (rest)=w883) -> (substring=w882:string)  [unwired: 1 in]
                                n476 = local write "Wavelength 2"(w882) -> ()
                                }
                              }
                            }
                          }
                          frame True {
                            n477 = stacked-sequence {
                              seq-local: [w893 _] -> [_ w913]
                              tunnel: w886 -> [w901 _]
                              frame #0 {
                                w890 = "ET" ("regular expression")
                                w899 = "DT" ("regular expression")
                                w903 = "CT" ("regular expression")
                                # "Wavelength not found in column 2"
                                n478 = Match Pattern(string=w901, regular expression=" ") -> (after substring=w904:string)  [unwired: 1 in, 3 out]
                                n479 = Match Pattern(string=w904, regular expression="@") -> (after substring=w889:string)  [unwired: 1 in, 3 out]
                                n480 = Match Pattern(string=w889, regular expression=w903) -> (before substring=w894:string, match substring=w902:string)  [unwired: 1 in, 2 out]
                                n481 = Match Pattern(string=w889, regular expression=w899) -> (before substring=w892:string, match substring=w900:string)  [unwired: 1 in, 2 out]
                                n482 = Match Pattern(string=w889, regular expression=w890) -> (before substring=w888:string, match substring=w891:string)  [unwired: 1 in, 2 out]
                                n483 = Equal?(x=w900, y=w899) -> (x = y?=w897:bool)
                                n484 = Equal?(x=w891, y=w890) -> (x = y?=w887:bool)
                                n485 = Equal?(x=w903, y=w902) -> (x = y?=w898:bool)
                                n486 = Build Array(w898, w897, w887) -> (w896:bool[])
                                n487 = Boolean Array To Number(Boolean array=w896) -> (number=w895:u32)
                                n488 = case shown="0, Default" w895 {
                                tunnel: w894 -> [_ w908 _ _]
                                tunnel: [w907 w908 w909 w910] -> w893
                                tunnel: w892 -> [_ _ w909 _]
                                tunnel: w889 -> [w907 _ _ _]
                                tunnel: w888 -> [_ _ _ w910]
                                frame 0, Default {
                                }
                                frame 1 {
                                # "CT Found"
                                }
                                frame 2 {
                                # "DT Found"
                                }
                                frame 4 {
                                # "ET Found"
                                }
                                }
                              }
                              frame #1 {
                                w914 = ""
                                n489 = String Length(string=w913) -> (length=w912:i32)
                                n490 = local write "Wavelength 2"(w914) -> ()
                                n491 = for {
                                N: w912 -> [_]
                                tunnel: w913 -> [w919]
                                tunnel: [w916] -> w911
                                tunnel: w914 -> [_]
                                i -> [w915]
                                w921 = string[] ["0", "1", "2", "3", "4", "5", "6", "7", "8", "9", ".", "-", "+", "A", "N", "D"]
                                n492 = String Subset(string=w919, offset (0)=w915, length (rest)=1 ("length (rest)")) -> (substring=w923:string)
                                n493 = Search 1D Array(1D array=w921, element=w923) -> (index of element=w920:i32)  [unwired: 1 in]
                                n494 = Not Equal?(x=w920, y=-1) -> (x != y?=w918:bool)
                                n495 = Index Array(array=w921, index=w920) -> (element=w917:string)
                                n496 = case shown="True" w918 {
                                tunnel: w917 -> [_ w929]
                                tunnel: [w925 w927] -> w916
                                frame False {
                                n497 = local read "Wavelength 2"() -> (w925:string)
                                }
                                frame True {
                                n498 = local read "Wavelength 2"() -> (w926:string)
                                n499 = To Lower Case(string=w929) -> (all lower case string=w928:string)
                                n500 = Concatenate Strings(w926, w928) -> (w927:string)
                                "Wavelength 2" <- w927
                                }
                                }
                                }
                                n501 = local write "Wavelength 2"(w911) -> ()
                              }
                            }
                          }
                        }
                        n502 = Reverse String(1:w862) -> (0:w863:string)
                        n503 = Equal?(x=w866, y=w867) -> (x = y?=w868:bool)
                        n504 = Match Pattern(string=w863, regular expression=" ") -> (before substring=w865:string, after substring=w869:string)  [unwired: 1 in, 2 out]
                        n505 = Reverse String(1:w865) -> (0:w864:string)
                        n506 = case shown="True" w868 {
                          tunnel: w864 -> [_ w932]
                          tunnel: w869 -> [_ w931]
                          frame False {
                            n507 = local write "Diameter"("") -> ()
                          }
                          frame True {
                            n508 = stacked-sequence {
                              seq-local: [w934 _] -> [_ w944]
                              seq-local: [w933 _] -> [_ w943]
                              tunnel: w932 -> [w937 w945]
                              tunnel: w931 -> [w935 _]
                              frame #0 {
                                n509 = Equal?(x=w937, y="") -> (x = y?=w933:bool)
                                n510 = case shown="False" w933 {
                                tunnel: w935 -> [w938 w941]
                                tunnel: [w938 w939] -> w934
                                frame False {
                                }
                                frame True {
                                n511 = Match Pattern(string=w941, regular expression=" ") -> (before substring=w940:string)  [unwired: 1 in, 3 out]
                                n512 = Reverse String(1:w940) -> (0:w939:string)
                                }
                                }
                              }
                              frame #1 {
                                n513 = case shown="False" w943 {
                                tunnel: w945 -> [w946 _]
                                tunnel: w944 -> [_ w947]
                                frame False {
                                n514 = local write "Diameter"(w946) -> ()
                                }
                                frame True {
                                n515 = local write "Diameter"(w947) -> ()
                                }
                                }
                              }
                            }
                          }
                        }
                      }
                      frame #2 {
                        w956 = "BBHR" ("regular expression")
                        # "BBHR is the same as BBPR"
                        # "If wavelength is blank, default to 10.6"
                        n516 = Match Pattern(string=w955, regular expression=w956) -> (match substring=w957:string)  [unwired: 1 in, 3 out]
                        n517 = Equal?(x=w957, y=w956) -> (x = y?=w952:bool)
                        n518 = Select(t="BBPR", s=w952, f=w955) -> (s? t:f=w953:string)
                        "Coating Type 2" <- w953
                        n519 = local read "Wavelength 2"() -> (w959:string)
                        n520 = Equal?(x=w959, y="") -> (x = y?=w951:bool)
                        n521 = Not(x=w948) -> (.not. x?=w949:bool)
                        n522 = And(x=w949, y=w951) -> (x .and. y?=w950:bool)
                        n523 = case shown="False" w950 {
                          frame False {
                          }
                          frame True {
                            n524 = local write "Wavelength 2"("10.6" ("Wavelength 2")) -> ()
                            n525 = One Button Dialog(message="The wavelength was not found and was set at 10.6 µm as default.  Please check the wavelength...") -> ()  [unwired: 1 in, 1 out]
                          }
                        }
                      }
                      frame #3 {
                        # "Coating Type"
                        # "Get Coating Type, Wavelengths, and Design #'s based on the Substrate from teh design info table"
                        n526 = local read "Wavelength 2"() -> (w964:string)
                        n527 = local write "Coating, Wavel, Design"(string[][] [] ("Coating, Wavel, Design")) -> ()
                        n528 = for {
                          tunnel: w965 -> [w1006] mode=indexing
                          tunnel: w963 -> [w981]
                          tunnel: w964 -> [w974]
                          tunnel: w962 -> [w970]
                          # "If BBPR exclude wavelength"
                          n529 = Index Array(array=w1006, index #1=1 ("disabled index (col)"), index #2=0 ("index (col)"), index #3=2 ("index (col)"), index #4=3 ("index (col)")) -> (element #1=w987:string, element #2=w982:string, element #3=w975:string, element #4=w1007:string)
                          n530 = local read "Substrate 2"() -> (w986:string)
                          n531 = To Upper Case(1:w975) -> (0:w977:string)
                          n532 = To Upper Case(1:w987) -> (0:w985:string)
                          n533 = To Upper Case(1:w982) -> (0:w983:string)
                          n534 = Search/Split String(string=w977, search string/char (-)=w974) -> (match + rest of string=w978:string)  [unwired: 1 in, 2 out]
                          n535 = Search/Split String(string=w985, search string/char (-)=w986) -> (match + rest of string=w1000:string)  [unwired: 1 in, 2 out]
                          n536 = Search/Split String(string=w983, search string/char (-)=w981) -> (match + rest of string=w984:string)  [unwired: 1 in, 2 out]
                          n537 = To Upper Case(1:w986) -> (0:w996:string)
                          n538 = Not Equal?(x=w978, y="") -> (x != y?=w969:bool)
                          n539 = Not Equal?(x=w1000, y="") -> (x != y?=w990:bool)
                          n540 = Not Equal?(x=w984, y="") -> (x != y?=w971:bool)
                          n541 = Equal?(x=w996, y="ZNS") -> (x = y?=w995:bool)
                          n542 = String Subset(string=w1000, offset (0)=3, length (rest)=1 ("length (rest)")) -> (substring=w993:string)
                          n543 = To Upper Case(1:w993) -> (0:w991:string)
                          n544 = Equal?(x=w991, y="E") -> (x = y?=w994:bool)
                          n545 = And(x=w995, y=w994) -> (x .and. y?=w989:bool)
                          n546 = Not(x=w989) -> (.not. x?=w988:bool)
                          n547 = Select(t=TRUE, s=w970, f=w969) -> (s? t:f=w967:bool)
                          n548 = And(x=w988, y=w990) -> (x .and. y?=w979:bool)
                          n549 = And(x=w979, y=w971) -> (x .and. y?=w973:bool)
                          n550 = And(x=w973, y=w967) -> (x .and. y?=w972:bool)
                          n551 = case shown="True" w972 {
                            tunnel: w982 -> [_ w1013]
                            tunnel: w975 -> [_ w1012]
                            tunnel: w1007 -> [_ w1011]
                            frame False {
                            }
                            frame True {
                              n552 = local read "Coating, Wavel, Design"() -> (w1010:string[][])
                              n553 = Build Array(w1013, w1012, w1011) -> (w1009:string[])
                              n554 = Insert Into Array(array=w1010, new element=w1009) -> (w1008:string[][])  [unwired: 2 in]
                              n555 = local write "Coating, Wavel, Design"(w1008) -> ()
                            }
                          }
                        }
                      }
                      frame #4 {
                        # "Coating Type"
                        # "Get available wavelengths"
                        n556 = local write "Wavelengths & Designs"(string[][] [] ("subarray")) -> ()
                        n557 = local read "Coating, Wavel, Design"() -> (w1022:string[][])
                        n558 = Index Array(array=w1022, index (col) #1=0 ("disabled index (col)"), index (col) #2=1 ("index (col)"), index (col) #3=2 ("index (col)")) -> (element #1=w1018:string[], element #2=w1023:string[], element #3=w1015:string[])  [unwired: 3 in]
                        n559 = for {
                          tunnel: w1021 -> [w1029]
                          tunnel: w1018 -> [w1031] mode=indexing
                          tunnel: w1023 -> [w1027] mode=indexing
                          tunnel: w1015 -> [w1026] mode=indexing
                          n560 = Search/Split String(string=w1031, search string/char (-)=w1029) -> (match + rest of string=w1030:string)  [unwired: 1 in, 2 out]
                          n561 = Not Equal?(x=w1030, y="") -> (x != y?=w1032:bool)
                          n562 = case shown="True" w1032 {
                            tunnel: w1027 -> [_ w1035]
                            tunnel: w1026 -> [_ w1034]
                            frame False {
                            }
                            frame True {
                              n563 = Build Array(w1035, w1034) -> (w1033:string[])
                              n564 = local read "Wavelengths & Designs"() -> (w1037:string[][])
                              n565 = Insert Into Array(array=w1037, new element=w1033) -> (→"Wavelengths & Designs":string[][])  [unwired: 2 in]
                            }
                          }
                        }
                        n566 = call "Sort Array.vi"("Sort Select"=T6."Sort By Name", "Array In"=w1018) -> ("Sorted Array"=w1019:string[])  [unwired: 4 in]
                        n567 = call "Delete Duplicates.vi"("Array In"=w1019) -> ("Array w/dup Deleted"=w1017:string[])  [unwired: 1 in]
                        n568 = property on="Coating Type" class="Ring (strict)"("Strings []"=w1017) -> ()  [unwired: 2 in, 2 out]
                      }
                      frame #5 {
                        # "Put wavelengths into list for manual selection"
                        n569 = local read "Wavelengths & Designs"() -> (w1041:string[][])
                        n570 = property on="Design# Match/es" class="Ring (strict)"("Strings []"=string[] []) -> ()  [unwired: 2 in, 2 out]
                        n571 = Index Array(array=w1041, index (col)=0 ("disabled index (col)")) -> (element=w1039:string[])  [unwired: 1 in]
                        n572 = call "Sort Array.vi"("Sort Select"=T6."Sort By Name", "Array In"=w1039) -> ("Sorted Array"=w1042:string[])  [unwired: 4 in]
                        n573 = call "Delete Duplicates.vi"("Array In"=w1042) -> ("Array w/dup Deleted"=w1038:string[])  [unwired: 1 in]
                        n574 = property on="Wavelength" class="Ring (strict)"("Strings []"=w1038) -> ()  [unwired: 2 in, 2 out]
                      }
                      frame #6 {
                        # "Format the wavelength column so it is wavelength numbers only."
                        n575 = To Upper Case(1:w1045) -> (0:w1047:string[])
                        n576 = for {
                          tunnel: w1047 -> [w1050] mode=indexing
                          tunnel: [w1048] -> w1046 mode=indexing
                          w1051 = ""
                          n577 = String Length(string=w1050) -> (length=w1049:i32)
                          n578 = for {
                            N: w1049 -> [_]
                            tunnel: [w1060] -> w1048
                            tunnel: w1051 -> [_]
                            tunnel: w1050 -> [w1059]
                            i -> [w1058]
                            w1054 = string[] ["0", "1", "2", "3", "4", "5", "6", "7", "8", "9", ".", "-", "+", "A", "N", "D"]
                            n579 = String Subset(string=w1059, offset (0)=w1058, length (rest)=1 ("length (rest)")) -> (substring=w1056:string)
                            n580 = Search 1D Array(1D array=w1054, element=w1056) -> (index of element=w1053:i32)  [unwired: 1 in]
                            n581 = Not Equal?(x=w1053, y=-1) -> (x != y?=w1061:bool)
                            n582 = Index Array(array=w1054, index=w1053) -> (element=w1052:string)
                            n583 = case shown="True" w1061 {
                              tunnel: w1052 -> [_ w1064]
                              tunnel: [w1062 w1065] -> w1060
                              frame False {
                                n584 = local read "Wavelength F"() -> (w1062:string)
                              }
                              frame True {
                                n585 = local read "Wavelength F"() -> (w1066:string)
                                n586 = To Lower Case(string=w1064) -> (all lower case string=w1063:string)
                                n587 = Concatenate Strings(w1066, w1063) -> (w1065:string)
                                "Wavelength F" <- w1065
                              }
                            }
                          }
                          n588 = local write "Wavelength F"(w1051) -> ()
                        }
                      }
                      frame #7 {
                        # "Search Wavelength array for matching wavelengths"
                        n589 = local read "Wavelength 2"() -> (w1067:string)
                        n590 = Index Array(array=w1068, index (col)=1 ("disabled index (col)")) -> (element=w1069:string[])  [unwired: 1 in]
                        n591 = local write "Possible Designs"(string[] [] ("Possible Designs")) -> ()
                        n592 = for {
                          tunnel: w1071 -> [w1075] mode=indexing
                          tunnel: w1069 -> [w1078] mode=indexing
                          tunnel: w1067 -> [w1073]
                          n593 = Search/Split String(string=w1075, search string/char (-)=w1073) -> (match + rest of string=w1077:string)  [unwired: 1 in, 2 out]
                          n594 = Not Equal?(x=w1077, y="") -> (x != y?=w1074:bool)
                          n595 = case shown="True" w1074 {
                            tunnel: w1078 -> [_ w1080]
                            frame False {
                            }
                            frame True {
                              n596 = local read "Possible Designs"() -> (w1081:string[])
                              n597 = Insert Into Array(array=w1081, new element=w1080) -> (w1079:string[])  [unwired: 1 in]
                              "Possible Designs" <- w1079
                              n598 = property on="Design# Match/es" class="Ring (strict)"("Strings []"=w1079) -> ()  [unwired: 2 in, 2 out]
                            }
                          }
                        }
                      }
                      frame #8 {
                        # "Set to false 8-23-12\nsince not needed any more."
                        n599 = case shown="False" w1082 {
                          tunnel: [w1084 FALSE ("Add to Worksheet")] -> w1083
                          frame False {
                            w1093 = 1 ("y")
                            n600 = property on="Design# Match/es" class="Ring (strict)"() -> ("Strings []"=w1089:string[])  [unwired: 2 in, 2 out]
                            n601 = Array Size(array=w1089) -> (size(s)=w1094:i32)
                            n602 = Index Array(array=w1089, index=0) -> (element=w1086:string)
                            n603 = Equal?(x=w1086, y="") -> (x = y?=w1085:bool)
                            n604 = Greater?(x=w1094, y=w1093) -> (0:w1095:bool)
                            n605 = Equal?(x=w1094, y=w1093) -> (x = y?=w1092:bool)
                            n606 = Build Array(w1095, w1092, w1085) -> (w1091:bool[])
                            n607 = Boolean Array To Number(Boolean array=w1091) -> (number=w1090:u32)
                            n608 = case shown="0, Default" w1090 {
                              tunnel: [FALSE ("Add to Worksheet") FALSE ("Add to Worksheet") FALSE ("Add to Worksheet")] -> w1084
                              frame 0, Default {
                                # "No Designs Found"
                                n609 = One Button Dialog(message="No Designs were found.  Designs can be found using the \"Pick Design\" option or the drop-down menus. If found click \"Add Selections to Worksheet\" button...") -> ()  [unwired: 1 in, 1 out]
                                "Lookup Failed" <- TRUE ("Lookup Failed")
                              }
                              frame 1 {
                                n610 = One Button Dialog(message="The search found more than one design.  Pick the design as needed...") -> ()  [unwired: 1 in, 1 out]
                                "Multiple Designs" <- TRUE ("Multiple Designs")
                              }
                              frame 2 {
                                # "One design, add to worksheet"
                              }
                            }
                            n611 = local write "Add to Worksheet"(w1084) -> ()
                          }
                          frame True {
                          }
                        }
                        "Lookup was True" <- w1083
                      }
                      frame #9 {
                        n612 = local read "Substrate 2"() -> (w1111:string)
                        n613 = property on="Substrate" class="Ring (strict)"() -> ("Strings []"=w1112:string[])  [unwired: 2 in, 2 out]
                        n614 = To Upper Case(1:w1112) -> (0:w1109:string[])
                        n615 = To Upper Case(1:w1111) -> (0:w1110:string)
                        n616 = Search 1D Array(1D array=w1109, element=w1110) -> (index of element=w1106:i32)  [unwired: 1 in]
                        n617 = Not Equal?(x=w1106, y=-1) -> (x != y?=w1104:bool)
                        n618 = case shown="True" w1104 {
                          tunnel: w1106 -> [_ w1113]
                          frame False {
                          }
                          frame True {
                            n619 = local write "Substrate"(w1113) -> ()
                          }
                        }
                        n620 = local write "Tab Control"(enum32{"Workcenter Report", "Run Worksheet"}."Run Worksheet" ("Tab Control")) -> ()
                        n621 = local write "Design# Match/es"(u16 0) -> ()
                      }
                    }
                  }
                  frame True {
                    # "Part number found"
                    n622 = local read "Coating Que / CTCL (T)?"() -> (w1117:bool)
                    n623 = Select(t=4, s=w1117, f=7 ("disabled index (col)")) -> (s? t:f=w1115:i32)
                    n624 = Index Array(array=w1119, index (row)=w1121, index (col)=w1115) -> (element=w1120:string)
                    n625 = local write "Part Description"(w1120) -> ()
                    n626 = local write "Tab Control"(enum32{"Workcenter Report", "Run Worksheet"}."Run Worksheet" ("Tab Control")) -> ()
                  }
                }
              }
            }
          }
        }
      }
      frame "Run Worksheet" {
        n627 = while {
          tunnel: w1126 -> [w1145]
          shift-right: [w1143] -> _
          shift-left: _ -> [w1142]
          shift-right: [w1141] -> _
          shift-left: _ -> [w1140]
          shift-right: [w1139] -> _
          shift-left: _ -> [w1138]
          tunnel: w1125 -> [_]
          shift-right: [w1137] -> _
          shift-left: _ -> [w1135]
          tunnel: w1124 -> [w1136]
          shift-right: [w1134] -> _
          shift-left: _ -> [w1133]
          tunnel: w1123 -> [w1132]
          tunnel: w1122 -> [w1131]
          shift-right: [w1130] -> _
          shift-left: _ -> [w1129]
          shift-right: [w1128] -> _
          shift-left: _ -> [w1127]
          stop <- FALSE continue-if-true
          n628 = stacked-sequence {
            seq-local: [_ _ _ w1808 _ _ _ _ _ _ _ _ _] -> [_ _ _ _ w1862 _ _ _ _ _ _ _ _]
            seq-local: [_ _ _ _ w1858 _ _ _ _ _ _ _ _] -> [_ _ _ _ _ w1900 _ _ _ _ _ _ _]
            seq-local: [_ _ _ _ _ _ _ _ w1997 _ _ _ _] -> [_ _ _ _ _ _ _ _ _ w2016 _ _ _]
            seq-local: [_ _ _ _ _ _ w1936 _ _ _ _ _ _] -> [_ _ _ _ _ _ _ _ w1995 _ _ _ _]
            tunnel: w1145 -> [_ _ _ _ _ _ _ _ _ w2015 _ _ _]
            tunnel: [_ _ _ "Substrate" _ _ _ _ _ _ _ _ _] -> w1143
            tunnel: w1142 -> [_ _ _ w1817 _ _ _ _ _ _ _ _ _]
            tunnel: [_ _ _ _ w1864 _ _ _ _ _ _ _ _] -> w1141
            tunnel: w1140 -> [_ _ _ _ w1863 _ _ _ _ _ _ _ _]
            tunnel: [_ _ _ _ _ w1899 _ _ _ _ _ _ _] -> w1139
            tunnel: w1138 -> [_ _ _ _ _ w1901 _ _ _ _ _ _ _]
            tunnel: [_ "System Select" _ _ _ _ _ _ _ _ _ _ _] -> w1137
            tunnel: w1136 -> [w1157 w1198 w1602 _ _ _ _ _ _ w2014 _ _ _]
            tunnel: w1135 -> [_ w1197 _ _ _ _ _ _ _ _ _ _ _]
            tunnel: [w1156 _ _ _ _ _ _ _ _ _ _ _ _] -> w1134
            tunnel: w1133 -> [w1155 _ _ _ _ _ _ _ _ _ _ _ _]
            tunnel: w1132 -> [w1151 w1193 _ w1813 _ _ _ _ w1994 _ _ _ _]
            tunnel: w1131 -> [_ _ _ _ _ _ _ _ _ w2013 _ _ _]
            tunnel: [_ _ _ _ _ _ _ _ _ _ "Reset Substrate List" _ _] -> w1130
            tunnel: w1129 -> [_ _ _ _ _ _ _ _ _ _ w2549 _ _]
            tunnel: [_ _ _ _ _ _ _ _ _ _ _ _ w2590] -> w1128
            tunnel: w1127 -> [_ _ _ _ _ _ _ _ _ _ _ _ w2589]
            frame #0 {
              w1149 = FALSE ("Visible")
              # "Monitor if active file changes"
              n629 = property on="Run Worksheet" class="Tbl (strict)"() -> ("EditPos"=w1146:T1)  [unwired: 2 in, 2 out]
              n630 = event shown="[0] Timeout" {
                selector: _ -> [_ _]
                dyn-events: _ -> [_ _]
                timeout: 1 -> [_ _]
                tunnel: w1146 -> [w1172 w1180]
                event Timeout {
                  n631 = event-data() -> ()  [unwired: 1 in, 2 out]
                  n632 = Unbundle(w1172) -> ("Row"=w1175:i32)  [unwired: 1 out]
                  n633 = Not Equal?(x=w1175, y=-2) -> (x != y?=w1173:bool)
                  n634 = case shown="True" w1173 {
                    tunnel: w1172 -> [_ w1177]
                    frame False {
                      n635 = local write "Return Key was Pressed"(FALSE ("Return Key was Pressed")) -> ()
                    }
                    frame True {
                      n636 = local read "Return Key was Pressed"() -> (w1178:bool)
                      n637 = case shown="False" w1178 {
                        tunnel: w1177 -> [w1179 _]
                        frame False {
                          "Edit Position 2" <- w1179
                        }
                        frame True {
                        }
                      }
                    }
                  }
                }
                event "Run Worksheet": Key Down {
                  # "Keep row edit position at the row before the return key is pressed."
                  n638 = event-data() -> ("VKey"=w1183:T7)  [unwired: 1 in, 4 out]
                  n639 = Equal?(x=w1183, y=eventvkey."Return") -> (x = y?=w1181:bool)
                  n640 = case shown="True" w1181 {
                    tunnel: w1180 -> [_ w1188]
                    frame False {
                    }
                    frame True {
                      n641 = Unbundle By Name(w1188) -> ("Row"=w1187:i32, "Column"=w1185:i32)
                      n642 = Decrement(x=w1187) -> (x-1=w1186:i32)
                      n643 = Bundle(w1186, "Column"=w1185) -> (w1184:cluster{i32, "Column":i32})  [unwired: 1 in]
                      n644 = local write "Edit Position 2"(w1184) -> ()
                      "Return Key was Pressed" <- TRUE ("Return Key was Pressed")
                    }
                  }
                }
              }
              n645 = property on="Search Text" class="Str"("Visible"=w1149) -> ()  [unwired: 2 in, 2 out]
              n646 = property on="Search Again" class="Bool"("Visible"=w1149) -> ()  [unwired: 2 in, 2 out]
              n647 = property on="System Select" class="Ring (strict)"() -> ("Ring Text.Text"=w1170:string)  [unwired: 2 in, 2 out]
              n648 = Path To String(path=w1157) -> (string=w1168:string)
              n649 = Concatenate Strings(w1168, "\\Run Worksheets\\" ("string"), "System " ("string"), w1170, " Run Worksheet.txt" ("string")) -> (w1166:string)
              n650 = Greater Than 0?(x=w1151) -> (x > 0?=w1152:bool)
              n651 = String To Path(string=w1166) -> (path=w1159:path)
              n652 = File/Directory Info(path=w1159) -> (last mod=w1150:timestamp, error out=w1160:errorcluster)  [unwired: 1 in, 5 out]
              n653 = To Unsigned Long Integer(number=w1150) -> (unsigned 32bit integer=w1156:u32)
              n654 = Not Equal?(x=w1156, y=w1155) -> (x != y?=w1148:bool)
              n655 = Subtract(x=w1156, y=w1155) -> (x-y=w1164:u32)
              n656 = Unbundle By Name(w1160) -> ("status"=w1165:bool)
              n657 = Greater Or Equal?(x=w1164, y=u32 5) -> (x >= y?=w1161:bool)
              n658 = Not(x=w1165) -> (.not. x?=w1162:bool)
              n659 = And(x=w1161, y=w1162) -> (x .and. y?=w1158:bool)
              n660 = And(x=w1158, y=w1148) -> (x .and. y?=w1153:bool)
              n661 = And(x=w1153, y=w1152) -> (x .and. y?=w1154:bool)
              n662 = case shown="True" w1154 {
                tunnel: w1159 -> [_ w1191]
                frame False {
                }
                frame True {
                  n663 = call-poly <vilib>:"Read Delimited Spreadsheet.vi"("file path (dialog if empty)"=w1191) -> ("all rows"=w1190:string[][])  [unwired: 9 in, 5 out]
                  n664 = local write "Run Worksheet"(w1190) -> ()
                  "Active File Changed" <- TRUE ("Active File Changed")
                }
              }
            }
            frame #1 {
              n665 = Not Equal?(x="System Select", y=w1197) -> (x != y?=w1196:bool)
              n666 = Equal To 0?(x=w1193) -> (x = 0?=w1195:bool)
              n667 = Or(x=w1196, y=w1195) -> (x .or. y?=w1194:bool)
              n668 = case shown="False" w1194 {
                tunnel: w1198 -> [w1200 w1547]
                frame False {
                  n669 = stacked-sequence {
                    tunnel: w1200 -> [_ w1274]
                    frame #0 {
                      n670 = while {
                        shift-right: ["Run Worksheet"] -> _
                        shift-left: _ -> [w1204]
                        stop <- TRUE stop-if-true
                        n671 = local read "Control Cluster was clicked"() -> (w1205:bool)
                        n672 = local read "Sys Select was True"() -> (w1206:bool)
                        n673 = case shown="True" w1206 {
                          frame False {
                          }
                          frame True {
                            n674 = local write "Sys Select was True"(FALSE ("Sys Select was True")) -> ()
                          }
                        }
                        n675 = case shown="True" w1205 {
                          frame False {
                          }
                          frame True {
                            n676 = local write "Control Cluster was clicked"(FALSE ("Control Cluster was clicked")) -> ()
                          }
                        }
                        n677 = local read "Transfer was True"() -> (w1202:bool)
                        n678 = Not Equal?(x="Run Worksheet", y=w1204) -> (x != y?=w1208:bool)
                        n679 = Not(x=w1202) -> (.not. x?=w1203:bool)
                        n680 = Not(x=w1206) -> (.not. x?=w1209:bool)
                        n681 = Compound Arithmetic op=AND(w1203, w1208, w1209) -> (w1207:bool)
                        n682 = case shown="False" w1207 {
                          tunnel: w1205 -> [_ w1252]
                          tunnel: w1202 -> [w1214 _]
                          tunnel: "Run Worksheet" -> [w1213 _]
                          frame False {
                            n683 = case shown="True" w1214 {
                              tunnel: w1213 -> [_ w1215]
                              frame False {
                              }
                              frame True {
                                n684 = stacked-sequence {
                                tunnel: w1215 -> [w1218 w1250]
                                frame #0 {
                                # "Transfer was true.  Do not check for design but\nupdate colors"
                                n685 = local read "Edit Position 2"() -> (w1219:T1)
                                n686 = Unbundle(w1219) -> ("Row"=w1216:i32)  [unwired: 1 out]
                                n687 = for {
                                N: 13 -> [_]
                                tunnel: w1216 -> [w1222]
                                tunnel: w1218 -> [w1221]
                                i -> [w1220]
                                # "Columns"
                                n688 = stacked-sequence {
                                seq-local: [_ w1237 _] -> [_ _ _]
                                seq-local: [w1230 _ _] -> [_ _ w1242]
                                seq-local: [w1223 _ _] -> [_ _ w1241]
                                tunnel: w1222 -> [w1227 w1236 _]
                                tunnel: w1220 -> [_ w1237 _]
                                tunnel: w1221 -> [w1235 _ _]
                                frame #0 {
                                w1224 = ""
                                n689 = Index Array(array=w1235, index (row) #1=w1227, index (col) #1=3 ("index"), index (row) #2=w1227, index (col) #2=6 ("index"), index (row) #3=w1227, index (col) #3=10 ("disabled index (col)")) -> (element #1=w1234:string, element #2=w1233:string, element #3=w1225:string)
                                n690 = Equal?(x=w1234, y=w1224) -> (x = y?=w1232:bool)
                                n691 = Equal?(x=w1233, y=w1224) -> (x = y?=w1231:bool)
                                n692 = And(x=w1232, y=w1231) -> (x .and. y?=w1230:bool)
                                n693 = Not Equal?(x=w1225, y=w1224) -> (x != y?=w1223:bool)
                                }
                                frame #1 {
                                n694 = Bundle("Row"=w1236, w1237) -> (w1238:cluster{"Row":i32, i32})  [unwired: 1 in]
                                n695 = property on="Run Worksheet" class="Tbl (strict)"("Active Cell:Active Cell"=w1238) -> ()  [unwired: 2 in, 2 out]
                                }
                                frame #2 {
                                n696 = Build Array(w1242, w1241) -> (w1240:bool[])
                                n697 = Boolean Array To Number(Boolean array=w1240) -> (number=w1239:u32)
                                n698 = case shown="2" w1239 {
                                tunnel: [u32 15790320 u32 16768430 u32 9371528] -> w1243
                                frame 0, Default {
                                }
                                frame 1 {
                                }
                                frame 2 {
                                }
                                }
                                n699 = property on="Run Worksheet" class="Tbl (strict)"("Active Cell:Cell Background Color"=w1243) -> ()  [unwired: 2 in, 2 out]
                                }
                                }
                                }
                                }
                                frame #1 {
                                # "Re-save to capture the new Run ID"
                                n700 = property on="System Select" class="Ring (strict)"() -> ("RingText.Text"=w1249:string)  [unwired: 2 in, 2 out]
                                n701 = local write "Transfer was True"(FALSE ("Transfer was True")) -> ()
                                n702 = call "Save Run Worksheet to 2 Folders.vi"("Message 1"="From Coating Schedule Run Builder - Transfer Row to Schedule: ", "System Select Text"=w1249, "Run Worksheet IN"=w1250) -> ("Run Worksheet Out"=w1248:string[][])  [unwired: 8 in]
                                n703 = local write "Run Worksheet"(w1248) -> ()
                                }
                                }
                              }
                            }
                          }
                          frame True {
                            # "Track changed rows"
                            n704 = case shown="False" w1252 {
                              frame False {
                                n705 = local read "Track Edit Positions"() -> (w1258:T1[])
                                n706 = local read "Edit Position 2"() -> (w1257:T1)
                                n707 = Insert Into Array(array=w1258, new element=w1257) -> (→"Track Edit Positions":T1[])  [unwired: 1 in]
                              }
                              frame True {
                                # "need at least one row all the time."
                                n708 = local read "Track Edit Positions"() -> (w1260:T1[])
                                n709 = local read "Edit Position 2"() -> (w1259:T1)
                                n710 = Array Size(array=w1260) -> (size(s)=w1263:i32)
                                n711 = Equal To 0?(x=w1263) -> (x = 0?=w1262:bool)
                                n712 = case shown="False" w1262 {
                                tunnel: [w1266 w1267] -> w1261
                                tunnel: w1260 -> [w1265 w1269]
                                tunnel: w1259 -> [w1264 w1268]
                                frame False {
                                n713 = Replace Array Subset(array=w1265, new element=w1264) -> (w1266:T1[])  [unwired: 1 in]
                                }
                                frame True {
                                n714 = Insert Into Array(array=w1269, new element=w1268) -> (w1267:T1[])  [unwired: 1 in]
                                }
                                }
                                n715 = local write "Track Edit Positions"(w1261) -> ()
                              }
                            }
                            n716 = local write "Timer 1"(0 ("Timer 1")) -> ()
                            n717 = property on="System Select" class="Ring (strict)"("DisabledEnum"=T5."Disabled and Grayed Out" ("Disabled")) -> ()  [unwired: 2 in, 2 out]
                            "Current Table Changed" <- TRUE ("Current Table Changed")
                          }
                        }
                      }
                    }
                    frame #1 {
                      # "Monitor if table changes every 5 seconds"
                      n718 = local read "Current Table Changed"() -> (w1273:bool)
                      n719 = local read "Timer 1"() -> (w1276:i32)
                      n720 = local read "Timer 1 Stpt."() -> (w1271:i32)
                      n721 = Increment(x=w1276) -> (x+1=w1272:i32)
                      n722 = Greater Or Equal?(x=w1272, y=w1271) -> (x >= y?=w1275:bool)
                      n723 = case shown="True" w1275 {
                        tunnel: w1274 -> [w1280 w1330]
                        tunnel: w1273 -> [_ w1327]
                        tunnel: w1272 -> [w1278 _]
                        tunnel: string[] ["", "Not Scheduled", "", "", "", "", "", "", "", "", "", "", ""] ("Build Schedule Table") -> [w1277 w1326]
                        frame False {
                          # "Clear table and mark as Not Scheduled."
                          n724 = case shown="True" "Not Scheduled" {
                            tunnel: w1280 -> [_ w1282]
                            tunnel: w1277 -> [_ w1281]
                            frame False {
                            }
                            frame True {
                              n725 = stacked-sequence {
                                seq-local: [_ w1286 _ _ _] -> [_ _ w1298 _ _]
                                seq-local: [w1283 _ _ _ _] -> [_ w1285 w1297 _ w1319]
                                seq-local: [_ _ _ w1313 _] -> [_ _ _ _ w1318]
                                seq-local: [_ _ _ w1306 _] -> [_ _ _ _ w1317]
                                tunnel: w1282 -> [_ w1287 _ _ _]
                                tunnel: w1281 -> [_ _ w1296 _ w1316]
                                frame #0 {
                                n726 = Two Button Dialog(message="Are you sure you want to clear the current worksheet?") -> (T button?=w1283:bool)  [unwired: 2 in]
                                }
                                frame #1 {
                                n727 = case shown="True" w1285 {
                                tunnel: w1287 -> [_ w1295]
                                tunnel: [_ w1294] -> w1286
                                frame False {
                                }
                                frame True {
                                # "blank table, resave as not scheduled"
                                n728 = property on="System Select" class="Ring (strict)"() -> ("RingText.Text"=w1289:string)  [unwired: 2 in, 2 out]
                                n729 = Path To String(path=w1295) -> (string=w1288:string)
                                n730 = Concatenate Strings(w1288, "\\Run Worksheets\\" ("string"), "System ", w1289, " Run Worksheet.txt" ("string")) -> (w1290:string)
                                n731 = String To Path(string=w1290) -> (path=w1294:path)
                                }
                                }
                                }
                                frame #2 {
                                n732 = case shown="True" w1297 {
                                tunnel: w1298 -> [_ w1300]
                                tunnel: w1296 -> [_ w1301]
                                frame False {
                                }
                                frame True {
                                # "blank table, resave as not scheduled"
                                n733 = Insert Into Array(array=string[][] [] ("Run Worksheet"), new element=w1301) -> (w1299:string[][])  [unwired: 2 in]
                                n734 = local write "Run Worksheet"(w1299) -> ()
                                n735 = call-poly <vilib>:"Write Delimited Spreadsheet.vi"("file path (dialog if empty)"=w1300, "2D data"=w1299) -> ()  [unwired: 12 in, 2 out]
                                }
                                }
                                }
                                frame #3 {
                                # "Get View Schedule-public path"
                                n736 = global read "Schedule Control Globals.vi" "Start path"() -> (w1304:path)
                                n737 = property on="System Select" class="Ring (strict)"() -> ("RingText.Text"=w1308:string)  [unwired: 2 in, 2 out]
                                n738 = call-poly <vilib>:"Read Delimited Spreadsheet.vi"("file path (dialog if empty)"=w1304) -> ("first row"=w1303:string[])  [unwired: 9 in, 5 out]
                                n739 = Index Array(array=w1303, index=12) -> (element=w1307:string)
                                n740 = Concatenate Strings(w1307, "\\Run Worksheets\\" ("string"), "System ", w1308, " Run Worksheet.txt" ("string")) -> (w1309:string)
                                n741 = String To Path(string=w1307) -> (path=w1312:path)
                                n742 = String To Path(string=w1309) -> (path=w1306:path)
                                n743 = Not Equal?(x=w1312, y=path "") -> (x != y?=w1313:bool)
                                }
                                frame #4 {
                                n744 = And(x=w1318, y=w1319) -> (x .and. y?=w1320:bool)
                                n745 = case shown="True" w1320 {
                                tunnel: w1317 -> [_ w1322]
                                tunnel: w1316 -> [_ w1323]
                                frame False {
                                }
                                frame True {
                                # "blank table, resave to View Schedule-Public as not scheduled"
                                n746 = Insert Into Array(array=string[][] [] ("Run Worksheet"), new element=w1323) -> (w1321:string[][])  [unwired: 2 in]
                                n747 = local write "Run Worksheet"(w1321) -> ()
                                n748 = call-poly <vilib>:"Write Delimited Spreadsheet.vi"("file path (dialog if empty)"=w1322, "2D data"=w1321) -> ()  [unwired: 12 in, 2 out]
                                }
                                }
                                }
                              }
                            }
                          }
                          "Timer 1" <- w1278
                        }
                        frame True {
                          n749 = local read "Track Edit Positions"() -> (w1325:T1[])
                          n750 = local read "Run Worksheet"() -> (w1328:string[][])
                          n751 = for {
                            tunnel: w1330 -> [w1335]
                            tunnel: w1328 -> [w1334]
                            tunnel: w1327 -> [w1333]
                            tunnel: w1326 -> [w1332]
                            tunnel: w1325 -> [w1331] mode=indexing
                            n752 = case shown="True" w1333 {
                              tunnel: w1335 -> [w1338 w1388]
                              tunnel: w1331 -> [_ w1387]
                              tunnel: w1334 -> [w1337 w1386]
                              tunnel: w1332 -> [w1336 _]
                              frame False {
                                n753 = stacked-sequence {
                                seq-local: [w1340 _ _ _ _] -> [_ w1348 w1359 _ w1381]
                                seq-local: [_ w1346 _ _ _] -> [_ _ w1358 _ _]
                                seq-local: [_ _ _ w1367 _] -> [_ _ _ _ w1380]
                                seq-local: [_ _ _ w1366 _] -> [_ _ _ _ w1378]
                                tunnel: w1338 -> [_ w1347 _ _ _]
                                tunnel: w1337 -> [w1339 _ _ _ _]
                                tunnel: w1336 -> [_ _ w1357 _ w1377]
                                frame #0 {
                                # "Check for blank table"
                                n754 = Array Size(array=w1339) -> (size(s)=w1345:i32[])
                                n755 = Index Array(array=w1345) -> (element #1=w1344:i32, element #2=w1343:i32)  [unwired: 2 in]
                                n756 = Equal To 0?(x=w1344) -> (x = 0?=w1342:bool)
                                n757 = Equal To 0?(x=w1343) -> (x = 0?=w1341:bool)
                                n758 = And(x=w1342, y=w1341) -> (x .and. y?=w1340:bool)
                                }
                                frame #1 {
                                n759 = case shown="True" w1348 {
                                tunnel: w1347 -> [_ w1350]
                                tunnel: [_ w1349] -> w1346
                                frame False {
                                }
                                frame True {
                                # "blank table, resave as not scheduled"
                                n760 = property on="System Select" class="Ring (strict)"() -> ("RingText.Text"=w1352:string)  [unwired: 2 in, 2 out]
                                n761 = Path To String(path=w1350) -> (string=w1351:string)
                                n762 = Concatenate Strings(w1351, "\\Run Worksheets\\" ("string"), "System ", w1352, " Run Worksheet.txt" ("string")) -> (w1353:string)
                                n763 = String To Path(string=w1353) -> (path=w1349:path)
                                }
                                }
                                }
                                frame #2 {
                                n764 = case shown="True" w1359 {
                                tunnel: w1358 -> [_ w1361]
                                tunnel: w1357 -> [_ w1362]
                                frame False {
                                }
                                frame True {
                                # "blank table, resave as not scheduled"
                                n765 = local read "Run Worksheet"() -> (w1363:string[][])
                                n766 = Insert Into Array(array=w1363, new element=w1362) -> (w1360:string[][])  [unwired: 2 in]
                                n767 = local write "Run Worksheet"(w1360) -> ()
                                n768 = call-poly <vilib>:"Write Delimited Spreadsheet.vi"("file path (dialog if empty)"=w1361, "2D data"=w1360) -> ()  [unwired: 12 in, 2 out]
                                }
                                }
                                }
                                frame #3 {
                                # "Get View Schedule-public path"
                                n769 = global read "Schedule Control Globals.vi" "Start path"() -> (w1365:path)
                                n770 = property on="System Select" class="Ring (strict)"() -> ("RingText.Text"=w1370:string)  [unwired: 2 in, 2 out]
                                n771 = call-poly <vilib>:"Read Delimited Spreadsheet.vi"("file path (dialog if empty)"=w1365) -> ("first row"=w1364:string[])  [unwired: 9 in, 5 out]
                                n772 = Index Array(array=w1364, index=12) -> (element=w1369:string)
                                n773 = Concatenate Strings(w1369, "\\Run Worksheets\\" ("string"), "System ", w1370, " Run Worksheet.txt" ("string")) -> (w1371:string)
                                n774 = String To Path(string=w1369) -> (path=w1374:path)
                                n775 = String To Path(string=w1371) -> (path=w1366:path)
                                n776 = Not Equal?(x=w1374, y=path "") -> (x != y?=w1367:bool)
                                }
                                frame #4 {
                                n777 = And(x=w1381, y=w1380) -> (x .and. y?=w1379:bool)
                                n778 = case shown="True" w1379 {
                                tunnel: w1378 -> [_ w1383]
                                tunnel: w1377 -> [_ w1384]
                                frame False {
                                }
                                frame True {
                                # "blank table, resave as not scheduled"
                                n779 = local read "Run Worksheet"() -> (w1385:string[][])
                                n780 = Insert Into Array(array=w1385, new element=w1384) -> (w1382:string[][])  [unwired: 2 in]
                                n781 = local write "Run Worksheet"(w1382) -> ()
                                n782 = call-poly <vilib>:"Write Delimited Spreadsheet.vi"("file path (dialog if empty)"=w1383, "2D data"=w1382) -> ()  [unwired: 12 in, 2 out]
                                }
                                }
                                }
                                }
                              }
                              frame True {
                                n783 = stacked-sequence {
                                seq-local: [_ _ _ _ w1439 _ _ _ _ _ _] -> [_ _ _ _ _ w1447 _ w1478 _ _ _]
                                seq-local: [_ _ _ w1427 _ _ _ _ _ _ _] -> [_ _ _ _ _ _ w1464 w1477 _ _ _]
                                seq-local: [_ _ _ w1431 _ _ _ _ _ _ _] -> [_ _ _ _ _ _ w1465 w1476 _ _ _]
                                seq-local: [_ _ w1417 _ _ _ _ _ _ _ _] -> [_ _ _ _ _ _ _ _ w1513 _ _]
                                seq-local: [_ _ w1416 _ _ _ _ _ _ _ _] -> [_ _ _ _ _ _ _ _ w1512 _ _]
                                seq-local: [_ _ w1414 _ _ _ _ _ _ _ _] -> [_ _ _ _ _ _ _ _ _ w1531 _]
                                seq-local: [w1396 _ _ _ _ _ _ _ _ _ _] -> [_ _ w1421 _ w1440 _ _ _ _ _ _]
                                seq-local: [_ w1404 _ _ _ _ _ _ _ _ _] -> [_ _ w1415 _ _ _ _ _ _ _ _]
                                seq-local: [_ w1401 _ _ _ _ _ _ _ _ _] -> [_ _ w1420 _ _ _ _ _ _ _ _]
                                seq-local: [_ w1402 _ _ _ _ _ _ _ _ _] -> [_ _ w1419 _ _ _ _ _ _ _ _]
                                seq-local: [_ w1403 _ _ _ _ _ _ _ _ _] -> [_ _ w1418 _ _ _ _ _ _ _ _]
                                seq-local: [_ _ w1413 _ _ _ _ _ _ _ _] -> [_ _ _ _ _ _ _ _ w1511 _ _]
                                seq-local: [_ _ w1412 _ _ _ _ _ _ _ _] -> [_ _ _ _ w1441 _ _ _ _ _ _]
                                seq-local: [_ _ _ _ w1438 _ _ _ _ _ _] -> [_ _ _ _ _ _ _ _ _ w1525 _]
                                seq-local: [w1389 _ _ _ _ _ _ _ _ _ _] -> [_ _ w1411 _ _ _ _ _ _ _ _]
                                tunnel: w1388 -> [w1390 w1407 _ _ _ _ _ _ _ _ _]
                                tunnel: w1387 -> [_ w1406 _ w1436 _ _ _ _ _ _ _]
                                tunnel: w1386 -> [_ w1405 w1422 w1424 _ _ _ _ _ _ _]
                                frame #0 {
                                w1400 = T5."Disabled and Grayed Out" ("Disabled")
                                n784 = property on="System Select" class="Ring (strict)"() -> ("RingText.Text"=w1396:string)  [unwired: 2 in, 2 out]
                                n785 = Path To String(path=w1390) -> (string=w1393:string)
                                n786 = local write "Current Table Changed"(FALSE ("Current Table Changed")) -> ()
                                n787 = Concatenate Strings(w1393, "\\" ("string"), "Design Info.txt" ("string")) -> (w1394:string)
                                n788 = String To Path(string=w1394) -> (path=w1395:path)
                                n789 = property on="System Select" class="Ring (strict)"("DisabledEnum"=w1400) -> ()  [unwired: 2 in, 2 out]
                                n790 = property on="Control Cluster" class="Clust (strict)"("DisabledEnum"=w1400) -> ()  [unwired: 2 in, 2 out]
                                n791 = call-poly <vilib>:"Read Delimited Spreadsheet.vi"("file path (dialog if empty)"=w1395) -> ("all rows"=w1389:string[][])  [unwired: 9 in, 5 out]
                                n792 = property on="Run Worksheet" class="Tbl (strict)"("DisabledEnum"=w1400) -> ()  [unwired: 2 in, 2 out]
                                n793 = local write "Sys Select was True"(TRUE ("Sys Select was True")) -> ()
                                n794 = property on="System Select" class="Ring (strict)"("DisabledEnum"=T5."Enabled" ("Disabled")) -> ()  [unwired: 2 in, 2 out]
                                }
                                frame #1 {
                                # "Verify Part Info design numbers"
                                n795 = Path To String(path=w1407) -> (string=w1410:string)
                                n796 = Concatenate Strings(w1410, "\\Part Number Info.txt" ("string")) -> (w1408:string)
                                n797 = String To Path(string=w1408) -> (path=w1402:path)
                                n798 = call-poly <vilib>:"Read Delimited Spreadsheet.vi"("file path (dialog if empty)"=w1402) -> ("all rows"=w1401:string[][])  [unwired: 9 in, 5 out]
                                n799 = call "Group Parts.vi"("Edit Position"=w1406, "Part Info"=w1401, "Run Worksheet"=w1405) -> ("Parts w/Info"=w1404:string[][], "to be scheduled row"=w1403:i32)  [unwired: 6 in, 1 out]
                                }
                                frame #2 {
                                # "Design Info"
                                # "Process Design Number from part info table where the top row design is used for the run.  Get all designs from the part info if any.  If there is not a design from the part info table, prompt to add it to the part info when the user picks the design."
                                n800 = call "Process Design Numbers from Part Info Table New.vi"("to be scheduled row"=w1418, "Design Info"=w1411, "Parts w/Info"=w1415, "Path"=w1419, "Part Info Table In"=w1420, "System #"=w1421, "Run Worksheet"=w1422) -> ("System Mismatch Designs"=w1414:string[][], "Highlight Rows"=w1416:i32[], "Design Error"=w1417:bool, "Run Worksheet Out"=w1412:string[][], "Error String"=w1413:string)
                                n801 = local write "Run Worksheet"(w1412) -> ()
                                }
                                frame #3 {
                                w1429 = 5 ("y")
                                # "total rows"
                                # "Setup rows to re-color.\n# of rows = total - current (10 min - current +-5)\nStarting row = current - 5 (min = 0)"
                                n802 = Array Size(array=w1424) -> (size(s)=w1423:i32[])
                                n803 = Unbundle By Name(w1436) -> ("Row"=w1435:i32)
                                n804 = Index Array(array=w1423) -> (element=w1425:i32)  [unwired: 1 in]
                                n805 = Subtract(x=w1425, y=w1435) -> (x-y=w1430:i32)
                                n806 = Subtract(x=w1435, y=w1429) -> (x-y=w1433:i32)
                                n807 = Less Than 0?(x=w1433) -> (x < 0?=w1434:bool)
                                n808 = Add(x=w1430, y=w1429) -> (x+y=w1426:i32)
                                n809 = Select(t=0, s=w1434, f=w1433) -> (s? t:f=w1431:i32)
                                n810 = Greater Or Equal?(x=w1426, y=w1425) -> (x >= y?=w1428:bool)
                                n811 = Select(t=w1425, s=w1428, f=w1426) -> (s? t:f=w1427:i32)
                                }
                                frame #4 {
                                # "Save Changes"
                                n812 = local read "Active File Changed"() -> (w1438:bool)
                                n813 = case shown="False" w1438 {
                                tunnel: w1441 -> [w1445 w1446]
                                tunnel: w1440 -> [w1444 _]
                                tunnel: [w1443 w1446] -> w1439
                                tunnel: "From Coating Schedule Run Builder - User changed item on worksheet: " ("Message 1") -> [w1442 _]
                                frame False {
                                n814 = call "Save Run Worksheet to 2 Folders.vi"("Message 1"=w1442, "System Select Text"=w1444, "Run Worksheet IN"=w1445) -> ("Run Worksheet Out"=w1443:string[][])  [unwired: 8 in]
                                n815 = local write "Run Worksheet"(w1443) -> ()
                                }
                                frame True {
                                # "Do not re-save if the file changed\ndue another user saving it."
                                }
                                }
                                }
                                frame #5 {
                                n816 = Index Array(array=w1447, index (col)=8 ("disabled index (col)")) -> (element=w1450:string[])  [unwired: 1 in]
                                n817 = call "Check for Duplicates.vi"("Data In"=w1450) -> ("Dup Ctrl"=w1448:bool, "Duplicate Text"=w1449:string)  [unwired: 1 in, 1 out]
                                n818 = case shown="True" w1448 {
                                tunnel: w1449 -> [_ w1455]
                                frame False {
                                }
                                frame True {
                                n819 = Equal?(x=w1455, y="S1") -> (x = y?=w1453:bool)
                                n820 = Equal?(x=w1455, y="S2") -> (x = y?=w1454:bool)
                                n821 = Or(x=w1453, y=w1454) -> (x .or. y?=w1452:bool)
                                n822 = Concatenate Strings("Run # " ("message"), w1455, " is a duplicate please fix..." ("string")) -> (w1458:string)
                                n823 = case shown="False" w1452 {
                                tunnel: w1458 -> [w1461 _]
                                frame False {
                                n824 = One Button Dialog(message=w1461) -> ()  [unwired: 1 in, 1 out]
                                }
                                frame True {
                                }
                                }
                                }
                                }
                                }
                                frame #6 {
                                # "Clear out Colors"
                                n825 = Add(x=20, y=w1464) -> (x+y=w1463:i32)
                                n826 = for {
                                N: w1463 -> [_]
                                tunnel: w1465 -> [w1467]
                                i -> [w1468]
                                # "Only clear from active current row"
                                # "Rows"
                                n827 = Add(x=w1467, y=w1468) -> (x+y=w1466:i32)
                                n828 = for {
                                N: 13 -> [_]
                                tunnel: w1466 -> [w1471]
                                i -> [w1470]
                                # "Columns"
                                n829 = stacked-sequence {
                                seq-local: [w1473 _] -> [_ _]
                                tunnel: w1471 -> [w1472 _]
                                tunnel: w1470 -> [w1473 _]
                                frame #0 {
                                n830 = Bundle(w1472, w1473) -> (w1474:cluster{i32, i32})  [unwired: 1 in]
                                n831 = property on="Run Worksheet" class="Tbl (strict)"("Active Cell:Active Cell"=w1474) -> ()  [unwired: 2 in, 2 out]
                                }
                                frame #1 {
                                n832 = property on="Run Worksheet" class="Tbl (strict)"("Active Cell:Cell Background Color"=u32 15790320) -> ()  [unwired: 2 in, 2 out]
                                }
                                }
                                }
                                }
                                }
                                frame #7 {
                                # "Update color on blank lines"
                                n833 = for {
                                N: w1477 -> [_]
                                tunnel: w1478 -> [w1483]
                                tunnel: w1476 -> [w1481]
                                i -> [w1482]
                                # "Rows"
                                n834 = Add(x=w1481, y=w1482) -> (x+y=w1480:i32)
                                n835 = for {
                                N: 13 -> [_]
                                tunnel: w1480 -> [w1486]
                                tunnel: w1483 -> [w1485]
                                i -> [w1484]
                                # "Columns"
                                n836 = stacked-sequence {
                                seq-local: [_ w1501 _] -> [_ _ _]
                                seq-local: [w1494 _ _] -> [_ _ w1506]
                                seq-local: [w1487 _ _] -> [_ _ w1505]
                                tunnel: w1486 -> [w1491 w1500 _]
                                tunnel: w1484 -> [_ w1501 _]
                                tunnel: w1485 -> [w1499 _ _]
                                frame #0 {
                                w1488 = ""
                                n837 = Index Array(array=w1499, index (row) #1=w1491, index (col) #1=3 ("index"), index (row) #2=w1491, index (col) #2=6 ("index"), index (row) #3=w1491, index (col) #3=10 ("disabled index (col)")) -> (element #1=w1498:string, element #2=w1497:string, element #3=w1489:string)
                                n838 = Equal?(x=w1498, y=w1488) -> (x = y?=w1496:bool)
                                n839 = Equal?(x=w1497, y=w1488) -> (x = y?=w1495:bool)
                                n840 = And(x=w1496, y=w1495) -> (x .and. y?=w1494:bool)
                                n841 = Not Equal?(x=w1489, y=w1488) -> (x != y?=w1487:bool)
                                }
                                frame #1 {
                                n842 = Bundle(w1500, w1501) -> (w1502:cluster{i32, i32})  [unwired: 1 in]
                                n843 = property on="Run Worksheet" class="Tbl (strict)"("Active Cell:Active Cell"=w1502) -> ()  [unwired: 2 in, 2 out]
                                }
                                frame #2 {
                                n844 = Build Array(w1506, w1505) -> (w1504:bool[])
                                n845 = Boolean Array To Number(Boolean array=w1504) -> (number=w1503:u32)
                                n846 = case shown="0, Default" w1503 {
                                tunnel: [u32 15790320 u32 16768430 u32 9371528] -> w1507
                                frame 0, Default {
                                }
                                frame 1 {
                                }
                                frame 2 {
                                }
                                }
                                n847 = property on="Run Worksheet" class="Tbl (strict)"("Active Cell:Cell Background Color"=w1507) -> ()  [unwired: 2 in, 2 out]
                                }
                                }
                                }
                                }
                                }
                                frame #8 {
                                n848 = case shown="True" w1513 {
                                tunnel: w1512 -> [_ w1515]
                                tunnel: w1511 -> [_ w1514]
                                frame False {
                                }
                                frame True {
                                n849 = stacked-sequence {
                                tunnel: w1515 -> [_ w1519]
                                tunnel: w1514 -> [w1516 _]
                                frame #0 {
                                n850 = local read "Disable Pop-up"() -> (w1517:bool)
                                n851 = case shown="False" w1517 {
                                tunnel: w1516 -> [w1518 _]
                                frame False {
                                n852 = One Button Dialog(message=w1518) -> ()  [unwired: 1 in, 1 out]
                                }
                                frame True {
                                }
                                }
                                }
                                frame #1 {
                                # "Highlight part numbers of unmatched designs"
                                n853 = for {
                                tunnel: w1519 -> [w1520] mode=indexing
                                n854 = stacked-sequence {
                                seq-local: [w1521 _] -> [_ _]
                                tunnel: w1520 -> [w1522 _]
                                frame #0 {
                                w1521 = 6
                                n855 = Bundle(w1522, w1521) -> (w1523:cluster{i32, i32})  [unwired: 1 in]
                                n856 = property on="Run Worksheet" class="Tbl (strict)"("Active Cell:Active Cell"=w1523) -> ()  [unwired: 2 in, 2 out]
                                }
                                frame #1 {
                                n857 = property on="Run Worksheet" class="Tbl (strict)"("Active Cell:Cell Background Color"=u32 16746639) -> ()  [unwired: 2 in, 2 out]
                                }
                                }
                                }
                                }
                                }
                                }
                                }
                                }
                                frame #9 {
                                n858 = Array Size(array=w1531) -> (size(s)=w1534:i32[])
                                n859 = Or(x="Disable Pop-up", y=w1525) -> (x .or. y?=w1526:bool)
                                n860 = Not(x=w1526) -> (.not. x?=w1529:bool)
                                n861 = case shown="True" w1525 {
                                frame False {
                                }
                                frame True {
                                n862 = local write "Active File Changed"(FALSE ("Active File Changed")) -> ()
                                }
                                }
                                n863 = Index Array(array=w1534, index=0) -> (element=w1532:i32)
                                n864 = Greater Than 0?(x=w1532) -> (x > 0?=w1530:bool)
                                n865 = And(x=w1530, y=w1529) -> (x .and. y?=w1528:bool)
                                n866 = case shown="True" w1528 {
                                tunnel: w1531 -> [_ w1536]
                                frame False {
                                }
                                frame True {
                                n867 = call "Verify part - Other Systems.vi"("System Mismatch Parts"=w1536) -> ()  [unwired: 11 in]
                                }
                                }
                                }
                                frame #10 {
                                w1543 = T5."Enabled" ("Disabled")
                                n868 = local write "Part Number Changed"(FALSE ("Part Number Changed")) -> ()
                                n869 = local write "Timer 1 Stpt."(20 ("Timer 1 Stpt.")) -> ()
                                n870 = property on="Run Worksheet" class="Tbl (strict)"("DisabledEnum"=w1543) -> ()  [unwired: 2 in, 2 out]
                                n871 = property on="System Select" class="Ring (strict)"("DisabledEnum"=w1543) -> ()  [unwired: 2 in, 2 out]
                                n872 = property on="Control Cluster" class="Clust (strict)"("DisabledEnum"=w1543) -> ()  [unwired: 2 in, 2 out]
                                n873 = local read "Track Edit Positions"() -> (w1540:T1[])
                                n874 = Delete From Array "Delete From Array"(array=w1540, length=1, index=0) -> (array with subset deleted=w1539:T1[])  [unwired: 1 out]
                                n875 = local write "Track Edit Positions"(w1539) -> ()
                                }
                                }
                              }
                            }
                          }
                          n876 = local write "Timer 1"(0 ("Timer 1")) -> ()
                        }
                      }
                    }
                  }
                }
                frame True {
                  # "Read in run worksheet"
                  n877 = stacked-sequence {
                    tunnel: w1547 -> [w1553 _ _]
                    frame #0 {
                      n878 = property on="System Select" class="Ring (strict)"() -> ("Ring Text.Text"=w1551:string)  [unwired: 2 in, 2 out]
                      n879 = Path To String(path=w1553) -> (string=w1554:string)
                      n880 = Concatenate Strings(w1554, "\\Run Worksheets\\" ("string"), "System " ("string"), w1551, " Run Worksheet.txt" ("string")) -> (w1556:string)
                      n881 = String To Path(string=w1556) -> (path=w1549:path)
                      n882 = call-poly <vilib>:"Read Delimited Spreadsheet.vi"("file path (dialog if empty)"=w1549) -> ("all rows"=w1548:string[][])  [unwired: 9 in, 5 out]
                      n883 = local write "Run Worksheet"(w1548) -> ()
                    }
                    frame #1 {
                      # "Clear out Colors"
                      n884 = for {
                        N: 50 -> [_]
                        i -> [w1558]
                        # "Rows"
                        n885 = for {
                          N: 13 -> [_]
                          tunnel: w1558 -> [w1561]
                          i -> [w1560]
                          # "Columns"
                          n886 = stacked-sequence {
                            seq-local: [w1563 _] -> [_ _]
                            tunnel: w1561 -> [w1562 _]
                            tunnel: w1560 -> [w1563 _]
                            frame #0 {
                              n887 = Bundle(w1562, w1563) -> (w1564:cluster{i32, i32})  [unwired: 1 in]
                              n888 = property on="Run Worksheet" class="Tbl (strict)"("Active Cell:Active Cell"=w1564) -> ()  [unwired: 2 in, 2 out]
                            }
                            frame #1 {
                              n889 = property on="Run Worksheet" class="Tbl (strict)"("Active Cell:Cell Background Color"=u32 15790320) -> ()  [unwired: 2 in, 2 out]
                            }
                          }
                        }
                      }
                    }
                    frame #2 {
                      # "Update color on blank lines"
                      n890 = local read "Run Worksheet"() -> (w1566:string[][])
                      n891 = for {
                        tunnel: w1566 -> [w1569] mode=indexing
                        tunnel: FALSE ("Sys was Changed") -> [w1568]
                        i -> [w1570]
                        # "Rows"
                        n892 = for {
                          tunnel: w1569 -> [w1575] mode=indexing
                          tunnel: w1570 -> [w1574]
                          tunnel: w1569 -> [w1572]
                          tunnel: w1568 -> [w1571]
                          i -> [w1573]
                          # "Columns"
                          n893 = stacked-sequence {
                            seq-local: [_ w1592 _] -> [_ _ _]
                            seq-local: [w1587 _ _] -> [_ _ w1596]
                            seq-local: [w1576 _ _] -> [_ _ w1597]
                            tunnel: w1575 -> [_ _ _]
                            tunnel: w1574 -> [_ w1591 _]
                            tunnel: w1573 -> [_ w1592 _]
                            tunnel: w1572 -> [w1590 _ _]
                            tunnel: w1571 -> [w1585 _ _]
                            frame #0 {
                              w1577 = ""
                              n894 = Index Array(array=w1590, index #1=3 ("index"), index #2=6 ("index"), index #3=10 ("index")) -> (element #1=w1588:string, element #2=w1580:string, element #3=w1578:string)
                              n895 = Equal?(x=w1588, y=w1577) -> (x = y?=w1583:bool)
                              n896 = Equal?(x=w1580, y=w1577) -> (x = y?=w1582:bool)
                              n897 = Not Equal?(x=w1578, y=w1577) -> (x != y?=w1576:bool)
                              n898 = And(x=w1583, y=w1582) -> (x .and. y?=w1581:bool)
                              n899 = Not(x=w1585) -> (.not. x?=w1586:bool)
                              n900 = And(x=w1586, y=w1581) -> (x .and. y?=w1587:bool)
                            }
                            frame #1 {
                              n901 = Bundle(w1591, w1592) -> (w1593:cluster{i32, i32})  [unwired: 1 in]
                              n902 = property on="Run Worksheet" class="Tbl (strict)"("Active Cell:Active Cell"=w1593) -> ()  [unwired: 2 in, 2 out]
                            }
                            frame #2 {
                              n903 = Build Array(w1596, w1597) -> (w1595:bool[])
                              n904 = Boolean Array To Number(Boolean array=w1595) -> (number=w1594:u32)
                              n905 = case shown="2" w1594 {
                                tunnel: [u32 15790320 u32 16768430 u32 9371528] -> w1598
                                frame 0, Default {
                                }
                                frame 1 {
                                }
                                frame 2 {
                                }
                              }
                              n906 = property on="Run Worksheet" class="Tbl (strict)"("Active Cell:Cell Background Color"=w1598) -> ()  [unwired: 2 in, 2 out]
                            }
                          }
                        }
                      }
                    }
                  }
                  n907 = local write "Part Number Changed"(FALSE ("Part Number Changed")) -> ()
                  n908 = local write "Timer 1 Stpt."(20 ("Timer 1 Stpt.")) -> ()
                  "Sys Select was True" <- TRUE ("Sys Select was True")
                }
              }
            }
            frame #2 {
              # "Other Options"
              n909 = case shown="3" "Other Options" {
                tunnel: w1602 -> [_ w1604 _ w1762 _]
                frame 0, Default {
                }
                frame 1 {
                  # "Update Substrate List"
                  n910 = stacked-sequence {
                    seq-local: [w1612 _ _ _] -> [_ w1615 _ _]
                    tunnel: w1604 -> [w1605 _ w1718 _]
                    frame #0 {
                      # "Read in Design Info Table"
                      n911 = Path To String(path=w1605) -> (string=w1609:string)
                      n912 = local write "Substrates 2"(string[] [] ("output array")) -> ()
                      n913 = Concatenate Strings(w1609, "\\" ("string"), "Design Info.txt" ("string")) -> (w1610:string)
                      n914 = String To Path(string=w1610) -> (path=w1611:path)
                      n915 = call-poly <vilib>:"Read Delimited Spreadsheet.vi"("file path (dialog if empty)"=w1611) -> ("all rows"=w1606:string[][])  [unwired: 9 in, 5 out]
                      n916 = Index Array(array=w1606, index (col)=1 ("disabled index (col)")) -> (element=w1612:string[])  [unwired: 1 in]
                    }
                    frame #1 {
                      n917 = for {
                        tunnel: w1615 -> [w1616] mode=indexing
                        w1620 = "(" ("regular expression")
                        w1627 = TRUE ("replace all? (F)")
                        w1623 = "*" ("replace string (\"\")")
                        # "Convert list to single substrate items only"
                        n918 = Match Pattern(string=w1616, regular expression=w1620) -> (before substring=w1618:string, match substring=w1621:string)  [unwired: 1 in, 2 out]
                        n919 = Equal?(x=w1621, y=w1620) -> (x = y?=w1619:bool)
                        n920 = Select(t=w1618, s=w1619, f=w1616) -> (s? t:f=w1617:string)
                        n921 = Search and Replace String(input string=w1617, search string="\\", replace string=w1623) -> (result string=w1622:string)  [unwired: 5 in, 3 out]
                        n922 = Search and Replace String(input string=w1622, search string="/", replace string=w1623) -> (result string=w1625:string)  [unwired: 5 in, 3 out]
                        n923 = Search and Replace String(replace all?=w1627, input string=w1625, search string=",", replace string=w1623) -> (result string=w1635:string)  [unwired: 4 in, 3 out]
                        n924 = Search and Replace String(input string=w1635, search string="&", replace string=w1623) -> (result string=w1634:string)  [unwired: 5 in, 3 out]
                        n925 = Search and Replace String(replace all?=w1627, input string=w1634, search string="or", replace string=w1623) -> (result string=w1644:string)  [unwired: 4 in, 3 out]
                        n926 = Search and Replace String(replace all?=w1627, input string=w1644, search string=";", replace string=w1623) -> (result string=w1637:string)  [unwired: 4 in, 3 out]
                        n927 = Search and Replace String(replace all?=w1627, input string=w1637, search string="\"") -> (result string=w1632:string)  [unwired: 5 in, 3 out]
                        n928 = Search and Replace String(replace all?=w1627, input string=w1632, search string="and", replace string=w1623) -> (result string=w1630:string)  [unwired: 4 in, 3 out]
                        n929 = Search and Replace String(replace all?=w1627, input string=w1630, search string=" ") -> (result string=w1628:string)  [unwired: 5 in, 3 out]
                        n930 = Match Pattern(string=w1628, regular expression=w1623) -> (before substring=w1640:string, match substring=w1642:string, after substring=w1639:string)  [unwired: 1 in, 1 out]
                        n931 = local write "Build Substr"("") -> ()
                        n932 = Equal?(x=w1642, y=w1623) -> (x = y?=w1641:bool)
                        n933 = case shown="True" w1641 {
                          tunnel: w1640 -> [_ w1674]
                          tunnel: w1639 -> [_ w1686]
                          tunnel: w1616 -> [w1667 _]
                          tunnel: w1616 -> [_ _]
                          frame False {
                            w1666 = " " ("y")
                            # "Remove leading and trailing spaces and put in array"
                            n934 = String Subset(string=w1667, length (rest)=1 ("length (rest)")) -> (substring=w1669:string)  [unwired: 1 in]
                            n935 = Equal?(x=w1669, y=w1666) -> (x = y?=w1668:bool)
                            n936 = Search and Replace String(input string=w1667, search string=w1666) -> (result string=w1665:string)  [unwired: 6 in, 3 out]
                            n937 = Select(t=w1665, s=w1668, f=w1667) -> (s? t:f=w1664:string)
                            n938 = Reverse String(1:w1664) -> (0:w1656:string)
                            n939 = local read "Substrates 2"() -> (w1672:string[])
                            n940 = String Subset(string=w1656, length (rest)=1 ("length (rest)")) -> (substring=w1662:string)  [unwired: 1 in]
                            n941 = Equal?(x=w1662, y=" ") -> (x = y?=w1659:bool)
                            n942 = Search and Replace String(input string=w1656, search string=" ") -> (result string=w1657:string)  [unwired: 6 in, 3 out]
                            n943 = Select(t=w1657, s=w1659, f=w1656) -> (s? t:f=w1660:string)
                            n944 = Reverse String(1:w1660) -> (0:w1648:string)
                            n945 = Equal?(x=w1648, y="FusedSilica") -> (x = y?=w1654:bool)
                            n946 = Select(t="Fused Silica", s=w1654, f=w1648) -> (s? t:f=w1647:string)
                            n947 = Equal?(x=w1647, y="Gewafers") -> (x = y?=w1652:bool)
                            n948 = Select(t="Ge Wafers", s=w1652, f=w1647) -> (s? t:f=w1649:string)
                            n949 = Insert Into Array(array=w1672, new element=w1649) -> (w1671:string[])  [unwired: 1 in]
                            n950 = local write "Substrates 2"(w1671) -> ()
                          }
                          frame True {
                            n951 = String Length(string=w1686) -> (length=w1683:i32)
                            n952 = Equal?(x=w1674, y="FusedSilica") -> (x = y?=w1680:bool)
                            n953 = Increment(x=w1683) -> (x+1=w1682:i32)
                            n954 = Select(t="Fused Silica", s=w1680, f=w1674) -> (s? t:f=w1673:string)
                            n955 = for {
                              N: w1682 -> [_]
                              tunnel: w1686 -> [w1693]
                              tunnel: w1683 -> [w1691]
                              i -> [w1687]
                              n956 = String Subset(string=w1693, offset (0)=w1687, length (rest)=1 ("length (rest)")) -> (substring=w1692:string)
                              n957 = Greater Or Equal?(x=w1687, y=w1691) -> (x >= y?=w1690:bool)
                              n958 = Equal?(x=w1692, y="*") -> (x = y?=w1688:bool)
                              n959 = Or(x=w1688, y=w1690) -> (x .or. y?=w1689:bool)
                              n960 = case shown="True" w1689 {
                                tunnel: w1692 -> [w1696 _]
                                frame False {
                                n961 = local read "Build Substr"() -> (w1698:string)
                                n962 = Concatenate Strings(w1698, w1696) -> (→"Build Substr":string)
                                }
                                frame True {
                                n963 = stacked-sequence {
                                seq-local: [w1699 _ _ _] -> [_ w1701 _ _]
                                seq-local: [_ w1700 _ _] -> [_ _ w1709 _]
                                frame #0 {
                                n964 = local read "Build Substr"() -> (w1699:string)
                                }
                                frame #1 {
                                n965 = Equal?(x=w1701, y="FusedSilica") -> (x = y?=w1707:bool)
                                n966 = Select(t="Fused Silica", s=w1707, f=w1701) -> (s? t:f=w1702:string)
                                n967 = Equal?(x=w1702, y="Gewafers") -> (x = y?=w1705:bool)
                                n968 = Select(t="Ge Wafers", s=w1705, f=w1702) -> (s? t:f=w1700:string)
                                }
                                frame #2 {
                                n969 = local read "Substrates 2"() -> (w1711:string[])
                                n970 = Insert Into Array(array=w1711, new element=w1709) -> (→"Substrates 2":string[])  [unwired: 1 in]
                                }
                                frame #3 {
                                n971 = local write "Build Substr"("") -> ()
                                }
                                }
                                }
                              }
                            }
                            n972 = Equal?(x=w1673, y="Gewafers") -> (x = y?=w1678:bool)
                            n973 = Select(t="Ge Wafers", s=w1678, f=w1673) -> (s? t:f=w1675:string)
                            n974 = local read "Substrates 2"() -> (w1685:string[])
                            n975 = Insert Into Array(array=w1685, new element=w1675) -> (w1684:string[])  [unwired: 1 in]
                            n976 = local write "Substrates 2"(w1684) -> ()
                          }
                        }
                      }
                    }
                    frame #2 {
                      # "Capitalize First Character"
                      # "Update Substrate List"
                      n977 = local read "Substrates 2"() -> (w1721:string[])
                      n978 = call "Delete Duplicates.vi"("Array In"=w1721) -> ("Array w/dup Deleted"=w1716:string[])  [unwired: 1 in]
                      n979 = for {
                        tunnel: w1716 -> [w1732] mode=indexing
                        tunnel: [w1728] -> w1715 mode=indexing
                        n980 = String Subset(string=w1732, length (rest)=1 ("length (rest)")) -> (substring=w1733:string)  [unwired: 1 in]
                        n981 = String Subset(string=w1732, offset (0)=1) -> (substring=w1729:string)  [unwired: 1 in]
                        n982 = To Upper Case(1:w1733) -> (0:w1730:string)
                        n983 = Concatenate Strings(w1730, w1729) -> (w1728:string)
                      }
                      n984 = Path To String(path=w1718) -> (string=w1719:string)
                      n985 = Concatenate Strings(w1719, "\\Substrate List.txt" ("string")) -> (w1720:string)
                      n986 = String To Path(string=w1720) -> (path=w1714:path)
                      n987 = call "Sort Array.vi"("Sort Select"=T6."Sort By Name", "Array In"=w1715) -> ("Sorted Array"=w1722:string[])  [unwired: 4 in]
                      n988 = Index Array(array=w1722, index=0) -> (element=w1725:string)
                      n989 = Equal?(x=w1725, y="") -> (x = y?=w1723:bool)
                      n990 = case shown="True" w1723 {
                        tunnel: w1722 -> [w1735 w1739]
                        tunnel: [w1735 w1736] -> w1713
                        frame False {
                        }
                        frame True {
                          n991 = Delete From Array(array=w1739, length=1, index=0) -> (array with subset deleted=w1736:string[])  [unwired: 1 out]
                        }
                      }
                      n992 = call-poly <vilib>:"Write Delimited Spreadsheet.vi"("file path (dialog if empty)"=w1714, "1D data"=w1713) -> ()  [unwired: 12 in, 2 out]
                      n993 = property on="Substrate" class="Ring (strict)"("Strings []"=w1713) -> ()  [unwired: 2 in, 2 out]
                    }
                    frame #3 {
                      w1740 = u16 0 items=["Other Options", "Update Substrate List"] ("Other Options")
                      n994 = local write "Other Options"(w1740) -> ()
                    }
                  }
                }
                frame 2 {
                  # "Print this worksheet"
                  n995 = stacked-sequence {
                    seq-local: [w1741 _] -> [_ _]
                    frame #0 {
                      # "Get Table info"
                      n996 = for {
                        N: 13 -> [_]
                        tunnel: [w1743] -> w1741 mode=indexing
                        i -> [w1744]
                        n997 = stacked-sequence {
                          tunnel: w1744 -> [w1747 _]
                          tunnel: [_ w1748] -> w1743
                          frame #0 {
                            n998 = Bundle(0, w1747) -> (w1745:cluster{i32, i32})  [unwired: 1 in]
                            n999 = property on="Run Worksheet" class="Tbl (strict)"("Active Cell:Active Cell"=w1745) -> ()  [unwired: 2 in, 2 out]
                          }
                          frame #1 {
                            n1000 = property on="Run Worksheet" class="Tbl (strict)"() -> ("Active Cell:Cell Size:Width"=w1748:u32)  [unwired: 2 in, 2 out]
                          }
                        }
                      }
                    }
                    frame #1 {
                      w1759 = u16 0 items=["Other Options", "Update Substrate List", "Print This Worksheet", "Print All Worksheets"] ("Other Options")
                      n1001 = property on="System Select" class="Ring (strict)"() -> ("Ring Text.Text"=w1757:string)  [unwired: 2 in, 2 out]
                      n1002 = local read "Run Worksheet"() -> (w1760:string[][])
                      n1003 = property on="Run Worksheet" class="Tbl (strict)"() -> ("Column Header Strings[]"=w1761:string[])  [unwired: 2 in, 2 out]
                      n1004 = Get Date/Time String() -> (date string=w1754:string, time string=w1752:string)  [unwired: 3 in]
                      n1005 = Concatenate Strings("System " ("string"), w1757, " Coating Schedule  " ("Heading"), w1754, "  " ("string"), w1752) -> (w1755:string)
                      n1006 = call "Print List (Landscape) color.vi"("Heading"=w1755, "Column Headers[]"=w1761, "Table In"=w1760, "Column Widths"=u32[] [62, 146, 159, 165, 81, 53, 90, 26, 55, 190, 57, 58, 55] ("Array"), "Use Default Printer?"=TRUE, "Hide Page Prompt"=TRUE) -> ()  [unwired: 2 in]
                      n1007 = local write "Other Options"(w1759) -> ()
                    }
                  }
                }
                frame 3 {
                  # "Print all worksheets"
                  n1008 = property on="System Select" class="Ring (strict)"() -> ("Strings []"=w1763:string[])  [unwired: 2 in, 2 out]
                  n1009 = for {
                    tunnel: w1763 -> [w1765] mode=indexing
                    tunnel: w1762 -> [w1764]
                    n1010 = stacked-sequence {
                      seq-local: [_ w1775 _] -> [_ _ w1794]
                      seq-local: [w1766 _ _] -> [_ _ w1785]
                      tunnel: w1765 -> [w1768 _ w1786]
                      tunnel: w1764 -> [w1769 _ _]
                      frame #0 {
                        n1011 = Path To String(path=w1769) -> (string=w1771:string)
                        n1012 = Concatenate Strings(w1771, "\\Run Worksheets\\" ("string"), "System ", w1768, " Run Worksheet.txt" ("string")) -> (w1770:string)
                        n1013 = String To Path(string=w1770) -> (path=w1767:path)
                        n1014 = call-poly <vilib>:"Read Delimited Spreadsheet.vi"("file path (dialog if empty)"=w1767) -> ("all rows"=w1766:string[][])  [unwired: 9 in, 5 out]
                      }
                      frame #1 {
                        # "Get Table info"
                        n1015 = for {
                          N: 13 -> [_]
                          tunnel: [w1777] -> w1775 mode=indexing
                          i -> [w1778]
                          n1016 = stacked-sequence {
                            tunnel: w1778 -> [w1781 _]
                            tunnel: [_ w1782] -> w1777
                            frame #0 {
                              n1017 = Bundle(0, w1781) -> (w1779:cluster{i32, i32})  [unwired: 1 in]
                              n1018 = property on="Run Worksheet" class="Tbl (strict)"("Active Cell:Active Cell"=w1779) -> ()  [unwired: 2 in, 2 out]
                            }
                            frame #1 {
                              n1019 = property on="Run Worksheet" class="Tbl (strict)"() -> ("Active Cell:Cell Size:Width"=w1782:u32)  [unwired: 2 in, 2 out]
                            }
                          }
                        }
                      }
                      frame #2 {
                        w1793 = u16 0 items=["Other Options", "Update Substrate List", "Print This Worksheet", "Print All Worksheets"] ("Other Options")
                        n1020 = property on="Run Worksheet" class="Tbl (strict)"() -> ("Column Header Strings[]"=w1795:string[])  [unwired: 2 in, 2 out]
                        n1021 = Get Date/Time String() -> (date string=w1789:string, time string=w1787:string)  [unwired: 3 in]
                        n1022 = Concatenate Strings("System " ("string"), w1786, " Coating Schedule  " ("Heading"), w1789, "  " ("string"), w1787) -> (w1790:string)
                        n1023 = call "Print List (Landscape) color.vi"("Heading"=w1790, "Column Headers[]"=w1795, "Table In"=w1785, "Column Widths"=w1794, "Use Default Printer?"=TRUE, "Hide Page Prompt"=TRUE) -> ()  [unwired: 2 in]
                        n1024 = local write "Other Options"(w1793) -> ()
                      }
                    }
                  }
                }
                frame 4 {
                  w1796 = u16 0 items=["Other Options", "Update Substrate List", "Print This Worksheet", "Print All Worksheets", "Open New Part Number Designs program"] ("Other Options")
                  # "Open new Part Number designs File"
                  n1025 = global read "Schedule Control Globals.vi" "New Part # File"() -> (w1801:path)
                  n1026 = Strip Path(path=w1801) -> (stripped path=w1803:path, name=w1802:string)
                  n1027 = local write "Other Options"(w1796) -> ()
                  n1028 = Concatenate Strings("Explorer " ("string"), w1802) -> (w1798:string)
                  n1029 = call <vilib>:"System Exec.vi"("wait until completion? (T)"=FALSE, "working directory"=w1803, "command line"=w1798) -> ("error out"=w1800:errorcluster)  [unwired: 5 in, 3 out]
                  n1030 = call <vilib>:"Simple Error Handler.vi"("error in (no error)"=w1800) -> ()  [unwired: 4 in, 5 out]
                }
              }
            }
            frame #3 {
              # "Substrate"
              n1031 = local read "Lookup Failed"() -> (w1810:bool)
              n1032 = local read "Lookup was True"() -> (w1816:bool)
              n1033 = local read "Multiple Designs"() -> (w1805:bool)
              n1034 = Equal To 0?(x=w1813) -> (x = 0?=w1812:bool)
              n1035 = Not(x=w1816) -> (.not. x?=w1815:bool)
              n1036 = Not(x=w1805) -> (.not. x?=w1804:bool)
              n1037 = Not Equal?(x="Substrate", y=w1817) -> (x != y?=w1814:bool)
              n1038 = Or(x=w1814, y=w1812) -> (x .or. y?=w1809:bool)
              n1039 = Or(x=w1810, y=w1809) -> (x .or. y?=w1808:bool)
              n1040 = And(x=w1809, y=w1815) -> (x .and. y?=w1811:bool)
              n1041 = Or(x=w1811, y=w1810) -> (x .or. y?=w1806:bool)
              n1042 = And(x=w1806, y=w1804) -> (x .and. y?=w1807:bool)
              n1043 = case shown="True" w1807 {
                frame False {
                  n1044 = local write "Multiple Designs"(FALSE ("Multiple Designs")) -> ()
                }
                frame True {
                  # "Update Coating Type List For Selected Substrate"
                  n1045 = local read "Pick Design was True"() -> (w1821:bool)
                  n1046 = case shown="False" w1821 {
                    frame False {
                      n1047 = stacked-sequence {
                        seq-local: [w1823 _ _ _] -> [_ w1831 _ _]
                        frame #0 {
                          # "Read in Design Info Table"
                          n1048 = global read "Schedule Control Globals.vi" "Data Path"() -> (w1822:path)
                          n1049 = Path To String(path=w1822) -> (string=w1826:string)
                          n1050 = local write "Coating, Wavel, Design"(string[][] [] ("Coating, Wavel, Design")) -> ()
                          n1051 = Concatenate Strings(w1826, "\\" ("string"), "Design Info.txt" ("string")) -> (w1827:string)
                          n1052 = String To Path(string=w1827) -> (path=w1828:path)
                          n1053 = call-poly <vilib>:"Read Delimited Spreadsheet.vi"("file path (dialog if empty)"=w1828) -> ("all rows"=w1823:string[][])  [unwired: 9 in, 5 out]
                          n1054 = property on="Coating Type" class="Ring (strict)"("Blinking"=TRUE) -> ()  [unwired: 2 in, 2 out]
                        }
                        frame #1 {
                          # "Get Coating Type, Wavelengths, and Design #'s based on the Substrate"
                          n1055 = for {
                            tunnel: w1831 -> [w1840] mode=indexing
                            n1056 = Index Array(array=w1840, index #1=1 ("disabled index (col)"), index #2=0 ("index (col)"), index #3=2 ("index (col)"), index #4=3 ("index (col)")) -> (element #1=w1833:string, element #2=w1842:string, element #3=w1841:string, element #4=w1835:string)
                            n1057 = property on="Substrate" class="Ring (strict)"() -> ("Ring Text.Text"=w1834:string)  [unwired: 2 in, 2 out]
                            n1058 = call "Substrate Search Criteria.vi"("Search String"=w1833, "Substrate"=w1834) -> ("Substrate Found"=w1832:bool)  [unwired: 9 in]
                            n1059 = case shown="True" w1832 {
                              tunnel: w1842 -> [_ w1848]
                              tunnel: w1841 -> [_ w1847]
                              tunnel: w1835 -> [_ w1846]
                              frame False {
                              }
                              frame True {
                                n1060 = local read "Coating, Wavel, Design"() -> (w1844:string[][])
                                n1061 = Build Array(w1848, w1847, w1846) -> (w1843:string[])
                                n1062 = Insert Into Array(array=w1844, new element=w1843) -> (→"Coating, Wavel, Design":string[][])  [unwired: 2 in]
                              }
                            }
                          }
                        }
                        frame #2 {
                          n1063 = local read "Coating, Wavel, Design"() -> (w1853:string[][])
                          n1064 = property on="Substrate" class="Ring (strict)"() -> ("Ring Text.Text"=w1850:string)  [unwired: 2 in, 2 out]
                          n1065 = Index Array(array=w1853, index (col)=0 ("disabled index (col)")) -> (element=w1852:string[])  [unwired: 1 in]
                          n1066 = local write "Substrate 2"(w1850) -> ()
                          n1067 = call "Sort Array.vi"("Sort Select"=T6."Sort By Name", "Array In"=w1852) -> ("Sorted Array"=w1855:string[])  [unwired: 4 in]
                          n1068 = call "Delete Duplicates.vi"("Array In"=w1855) -> ("Array w/dup Deleted"=w1854:string[])  [unwired: 1 in]
                          n1069 = local write "Coating Type"(u16 0) -> ()
                          n1070 = property on="Coating Type" class="Ring (strict)"("Strings []"=w1854) -> ()  [unwired: 2 in, 2 out]
                        }
                        frame #3 {
                          n1071 = property on="Coating Type" class="Ring (strict)"("Blinking"=FALSE) -> ()  [unwired: 2 in, 2 out]
                        }
                      }
                    }
                    frame True {
                      # "Pick Design was True"
                    }
                  }
                  n1072 = local write "Lookup Failed"(FALSE ("Lookup Failed")) -> ()
                }
              }
            }
            frame #4 {
              n1073 = local read "Lookup was True"() -> (w1861:bool)
              n1074 = property on="Coating Type" class="Ring (strict)"() -> ("Ring Text.Text"=w1864:string)  [unwired: 2 in, 2 out]
              n1075 = Not Equal?(x=w1864, y=w1863) -> (x != y?=w1865:bool)
              n1076 = Or(x=w1865, y=w1862) -> (x .or. y?=w1858:bool)
              n1077 = Not(x=w1861) -> (.not. x?=w1859:bool)
              n1078 = And(x=w1858, y=w1859) -> (x .and. y?=w1860:bool)
              n1079 = case shown="False" w1860 {
                tunnel: w1864 -> [_ _]
                tunnel: w1864 -> [_ w1867]
                frame False {
                }
                frame True {
                  n1080 = case shown="False" "Pick Design was True" {
                    tunnel: w1867 -> [w1868 _]
                    frame False {
                      n1081 = stacked-sequence {
                        tunnel: w1868 -> [_ w1870 w1889 _]
                        frame #0 {
                          n1082 = property on="Wavelength" class="Ring (strict)"("Blinking"=TRUE) -> ()  [unwired: 2 in, 2 out]
                        }
                        frame #1 {
                          # "Coating Type"
                          n1083 = local write "Wavelengths"(string[] [] ("subarray")) -> ()
                          n1084 = local read "Coating, Wavel, Design"() -> (w1871:string[][])
                          n1085 = Index Array(array=w1871, index (col) #1=0 ("disabled index (col)"), index (col) #2=1 ("index (col)")) -> (element #1=w1873:string[], element #2=w1872:string[])  [unwired: 2 in]
                          n1086 = for {
                            tunnel: w1870 -> [w1878]
                            tunnel: w1873 -> [w1880] mode=indexing
                            tunnel: w1872 -> [w1882]
                            i -> [w1883]
                            n1087 = Search/Split String(string=w1880, search string/char (-)=w1878) -> (match + rest of string=w1879:string)  [unwired: 1 in, 2 out]
                            n1088 = Index Array(array=w1882, index=w1883) -> (element=w1881:string)
                            n1089 = Not Equal?(x=w1879, y="") -> (x != y?=w1884:bool)
                            n1090 = case shown="True" w1884 {
                              tunnel: w1881 -> [_ w1885]
                              frame False {
                              }
                              frame True {
                                n1091 = local read "Wavelengths"() -> (w1886:string[])
                                n1092 = Insert Into Array(array=w1886, new element=w1885) -> (w1887:string[])  [unwired: 1 in]
                                n1093 = local write "Wavelengths"(w1887) -> ()
                              }
                            }
                          }
                        }
                        frame #2 {
                          n1094 = local read "Wavelengths"() -> (w1892:string[])
                          n1095 = local write "Coating Type 2"(w1889) -> ()
                          n1096 = call "Sort Array.vi"("Sort Select"=T6."Sort By Name", "Array In"=w1892) -> ("Sorted Array"=w1891:string[])  [unwired: 4 in]
                          n1097 = call "Delete Duplicates.vi"("Array In"=w1891) -> ("Array w/dup Deleted"=w1890:string[])  [unwired: 1 in]
                          n1098 = property on="Wavelength" class="Ring (strict)"("Strings []"=w1890) -> ()  [unwired: 2 in, 2 out]
                          n1099 = local write "Wavelength"(u16 0) -> ()
                        }
                        frame #3 {
                          n1100 = property on="Wavelength" class="Ring (strict)"("Blinking"=FALSE) -> ()  [unwired: 2 in, 2 out]
                        }
                      }
                    }
                    frame True {
                      # "Pick Design was True"
                    }
                  }
                }
              }
            }
            frame #5 {
              n1101 = property on="Wavelength" class="Ring (strict)"() -> ("Ring Text.Text"=w1899:string)  [unwired: 2 in, 2 out]
              n1102 = Not Equal?(x=w1899, y=w1901) -> (x != y?=w1902:bool)
              n1103 = Or(x=w1902, y=w1900) -> (x .or. y?=w1895:bool)
              n1104 = local read "Lookup was True"() -> (w1896:bool)
              n1105 = Not(x=w1896) -> (.not. x?=w1898:bool)
              n1106 = And(x=w1898, y=w1895) -> (x .and. y?=w1897:bool)
              n1107 = case shown="True" w1897 {
                tunnel: w1899 -> [_ _]
                tunnel: w1899 -> [_ w1904]
                tunnel: w1896 -> [_ _]
                frame False {
                }
                frame True {
                  n1108 = local read "Pick Design was True"() -> (w1903:bool)
                  n1109 = case shown="False" w1903 {
                    tunnel: w1904 -> [w1905 _]
                    frame False {
                      n1110 = stacked-sequence {
                        tunnel: w1905 -> [_ w1909 w1930 _]
                        frame #0 {
                          n1111 = property on="Design# Match/es" class="Ring (strict)"("Blinking"=TRUE) -> ()  [unwired: 2 in, 2 out]
                        }
                        frame #1 {
                          # "wavelength"
                          n1112 = local write "Possible Designs"(string[] [] ("subarray")) -> ()
                          n1113 = property on="Coating Type" class="Ring (strict)"() -> ("Ring Text.Text"=w1908:string)  [unwired: 2 in, 2 out]
                          n1114 = local read "Coating, Wavel, Design"() -> (w1907:string[][])
                          n1115 = for {
                            tunnel: w1909 -> [w1915]
                            tunnel: w1908 -> [w1912]
                            tunnel: w1907 -> [w1922] mode=indexing
                            w1914 = ""
                            n1116 = Index Array(array=w1922, index #1=1 ("disabled index (col)"), index #2=0 ("index (col)"), index #3=2 ("index (col)")) -> (element #1=w1916:string, element #2=w1913:string, element #3=w1918:string)
                            n1117 = Search/Split String(string=w1913, search string/char (-)=w1912) -> (match + rest of string=w1911:string)  [unwired: 1 in, 2 out]
                            n1118 = Search/Split String(string=w1916, search string/char (-)=w1915) -> (match + rest of string=w1917:string)  [unwired: 1 in, 2 out]
                            n1119 = Not Equal?(x=w1917, y=w1914) -> (x != y?=w1924:bool)
                            n1120 = Not Equal?(x=w1911, y=w1914) -> (x != y?=w1925:bool)
                            n1121 = And(x=w1924, y=w1925) -> (x .and. y?=w1923:bool)
                            n1122 = case shown="False" w1923 {
                              tunnel: w1918 -> [_ w1926]
                              frame False {
                              }
                              frame True {
                                n1123 = local read "Possible Designs"() -> (w1927:string[])
                                n1124 = Insert Into Array(array=w1927, new element=w1926) -> (w1928:string[])  [unwired: 1 in]
                                n1125 = local write "Possible Designs"(w1928) -> ()
                              }
                            }
                          }
                        }
                        frame #2 {
                          n1126 = local write "Wavelength 2"(w1930) -> ()
                          n1127 = local read "Possible Designs"() -> (w1933:string[])
                          n1128 = call "Sort Array.vi"("Sort Select"=T6."Sort By Name", "Array In"=w1933) -> ("Sorted Array"=w1932:string[])  [unwired: 4 in]
                          n1129 = call "Delete Duplicates.vi"("Array In"=w1932) -> ("Array w/dup Deleted"=w1931:string[])  [unwired: 1 in]
                          n1130 = local write "Design# Match/es"(u16 0) -> ()
                          n1131 = property on="Design# Match/es" class="Ring (strict)"("Strings []"=w1931) -> ()  [unwired: 2 in, 2 out]
                        }
                        frame #3 {
                          n1132 = property on="Design# Match/es" class="Ring (strict)"("Blinking"=FALSE) -> ()  [unwired: 2 in, 2 out]
                        }
                      }
                    }
                    frame True {
                    }
                  }
                }
              }
            }
            frame #6 {
              n1133 = while {
                tunnel: [w1937] -> w1936
                stop <- TRUE stop-if-true
                n1134 = Cluster To Array(cluster="Control Cluster") -> (array=w1940:bool[])
                n1135 = Boolean Array To Number(Boolean array=w1940) -> (number=w1937:u32)
                n1136 = case shown="2" w1937 {
                  frame 0, Default {
                  }
                  frame 1 {
                    w1944 = FALSE ("Insert Row")
                    # "Insert Row"
                    n1137 = local read "Edit Position 2"() -> (w1942:T1)
                    n1138 = local read "Run Worksheet"() -> (w1947:string[][])
                    n1139 = Unbundle(w1942) -> ("Row"=w1946:i32)  [unwired: 1 out]
                    n1140 = Bundle("Insert Row"=w1944, "Insert Row"=w1944, "Insert Row"=w1944, "Insert Row"=w1944, "Insert Row"=w1944, "Insert Row"=w1944) -> (w1943:T8)  [unwired: 1 in]
                    n1141 = Insert Into Array(array=w1947, index (row)=w1946, new element=string[] ["", "", "", "", "", "", "", "", "", "", "", ""] ("Build Schedule Table")) -> (w1945:string[][])  [unwired: 1 in]
                    n1142 = local write "Control Cluster"(w1943) -> ()
                    n1143 = local write "Run Worksheet"(w1945) -> ()
                  }
                  frame 2 {
                    w1953 = FALSE ("Insert Row")
                    # "Delete Row"
                    n1144 = local read "Edit Position 2"() -> (w1948:T1)
                    n1145 = local read "Run Worksheet"() -> (w1951:string[][])
                    n1146 = Unbundle(w1948) -> ("Row"=w1949:i32)  [unwired: 1 out]
                    n1147 = Bundle("Insert Row"=w1953, "Insert Row"=w1953, "Insert Row"=w1953, "Insert Row"=w1953, "Insert Row"=w1953, "Insert Row"=w1953) -> (w1952:T8)  [unwired: 1 in]
                    n1148 = Delete From Array(array=w1951, index (row)=w1949) -> (array with subset deleted=w1950:string[][])  [unwired: 2 in, 1 out]
                    n1149 = local write "Control Cluster"(w1952) -> ()
                    n1150 = local write "Run Worksheet"(w1950) -> ()
                  }
                  frame 4 {
                    w1959 = FALSE ("Insert Row")
                    # "Move selected row data up"
                    n1151 = local read "Edit Position 2"() -> (w1954:T1)
                    n1152 = local read "Run Worksheet"() -> (w1960:string[][])
                    n1153 = Bundle("Insert Row"=w1959, "Insert Row"=w1959, "Insert Row"=w1959, "Insert Row"=w1959, "Insert Row"=w1959, "Insert Row"=w1959) -> (w1958:T8)  [unwired: 1 in]
                    n1154 = Unbundle(w1954) -> ("Row"=w1955:i32, "Column"=w1957:i32)
                    n1155 = local write "Control Cluster"(w1958) -> ()
                    n1156 = Greater Than 0?(x=w1955) -> (x > 0?=w1956:bool)
                    n1157 = case shown="True" w1956 {
                      tunnel: w1960 -> [_ w1969]
                      tunnel: w1955 -> [_ w1965]
                      tunnel: w1957 -> [_ w1961]
                      frame False {
                      }
                      frame True {
                        n1158 = Decrement(x=w1965) -> (x-1=w1963:i32)
                        n1159 = Index Array(array=w1969, index (row) #1=w1963, index (row) #2=w1965) -> (element #1=w1967:string[], element #2=w1968:string[])  [unwired: 2 in]
                        n1160 = Bundle(w1963, "Column"=w1961) -> (w1964:cluster{i32, "Column":i32})  [unwired: 1 in]
                        n1161 = property on="Run Worksheet" class="Tbl (strict)"("EditPos"=w1964) -> ()  [unwired: 2 in, 2 out]
                        n1162 = Replace Array Subset(array=w1969, new element #1=w1968, index (row) #1=w1963, new element #2=w1967, index (row) #2=w1965) -> (w1966:string[][])  [unwired: 2 in]
                        n1163 = Bundle(w1963, "Column"=w1961) -> (w1962:cluster{i32, "Column":i32})  [unwired: 1 in]
                        n1164 = property on="Run Worksheet" class="Tbl (strict)"("Active Cell"=w1962) -> ()  [unwired: 2 in, 2 out]
                        n1165 = local write "Edit Position 2"(w1964) -> ()
                        n1166 = local write "Run Worksheet"(w1966) -> ()
                        n1167 = property on="Run Worksheet" class="Tbl (strict)"("Selection Start"=w1962) -> ()  [unwired: 2 in, 2 out]
                      }
                    }
                  }
                  frame 8 {
                    w1980 = FALSE ("Insert Row")
                    # "Move selected row data Down"
                    n1168 = local read "Edit Position 2"() -> (w1970:T1)
                    n1169 = local read "Run Worksheet"() -> (w1977:string[][])
                    n1170 = Unbundle(w1970) -> ("Row"=w1973:i32, "Column"=w1978:i32)
                    n1171 = Bundle("Insert Row"=w1980, "Insert Row"=w1980, "Insert Row"=w1980, "Insert Row"=w1980, "Insert Row"=w1980, "Insert Row"=w1980) -> (w1979:T8)  [unwired: 1 in]
                    n1172 = local write "Control Cluster"(w1979) -> ()
                    n1173 = Array Size(array=w1977) -> (size(s)=w1976:i32[])
                    n1174 = Index Array(array=w1976, index=0) -> (element=w1972:i32)
                    n1175 = Decrement(x=w1972) -> (x-1=w1971:i32)
                    n1176 = Greater Or Equal?(x=w1973, y=w1971) -> (x >= y?=w1974:bool)
                    n1177 = case shown="False" w1974 {
                      tunnel: w1977 -> [w1989 _]
                      tunnel: w1978 -> [w1981 _]
                      tunnel: w1973 -> [w1988 _]
                      frame False {
                        n1178 = Increment(x=w1988) -> (x+1=w1982:i32)
                        n1179 = Index Array(array=w1989, index (row) #1=w1982, index (row) #2=w1988) -> (element #1=w1986:string[], element #2=w1987:string[])  [unwired: 2 in]
                        n1180 = Bundle(w1982, "Column"=w1981) -> (w1984:cluster{i32, "Column":i32})  [unwired: 1 in]
                        n1181 = property on="Run Worksheet" class="Tbl (strict)"("EditPos"=w1984) -> ()  [unwired: 2 in, 2 out]
                        n1182 = Replace Array Subset(array=w1989, new element #1=w1987, index (row) #1=w1982, new element #2=w1986, index (row) #2=w1988) -> (w1985:string[][])  [unwired: 2 in]
                        n1183 = Bundle(w1982, "Column"=w1981) -> (w1983:cluster{i32, "Column":i32})  [unwired: 1 in]
                        n1184 = local write "Edit Position 2"(w1984) -> ()
                        n1185 = local write "Run Worksheet"(w1985) -> ()
                        n1186 = property on="Run Worksheet" class="Tbl (strict)"("Active Cell"=w1983) -> ()  [unwired: 2 in, 2 out]
                        n1187 = property on="Run Worksheet" class="Tbl (strict)"("Selection Start"=w1983) -> ()  [unwired: 2 in, 2 out]
                      }
                      frame True {
                      }
                    }
                  }
                }
              }
            }
            frame #7 {
              # "Prevent control cluster clicks from triggering the \"Track Edits\" action."
              n1188 = event shown="[1] \"Control Cluster\": Mouse Down" {
                selector: _ -> [_ _]
                dyn-events: _ -> [_ _]
                timeout: 1 -> [_ _]
                event Timeout {
                  n1189 = event-data() -> ()  [unwired: 1 in, 2 out]
                }
                event "Control Cluster": Mouse Down {
                  n1190 = event-data() -> ()  [unwired: 1 in, 7 out]
                  "Control Cluster was clicked" <- TRUE ("Control Cluster was clicked")
                }
              }
            }
            frame #8 {
              # "Change timer 1 from 20 to 2 when only the part number changes"
              n1191 = Build Array("Pick Design", "Add to Worksheet", "Transfer to Schedule", "Transfer to Other Worksheet") -> (w1998:bool[])
              n1192 = Boolean Array To Number(Boolean array=w1998) -> (number=w1997:u32)
              n1193 = Not Equal To 0?(x=w1994) -> (x != 0?=w1993:bool)
              n1194 = while {
                shift-right: [w2006] -> _
                shift-left: _ -> [w2008]
                tunnel: w1995 -> [w2004]
                tunnel: w1993 -> [w2001]
                stop <- TRUE stop-if-true
                n1195 = local read "Run Worksheet"() -> (w2009:string[][])
                n1196 = Index Array(array=w2009, index (col)=6 ("disabled index (col)")) -> (element=w2006:string[])  [unwired: 1 in]
                n1197 = Equal To 0?(x=w2004) -> (x = 0?=w2002:bool)
                n1198 = Not Equal?(x=w2006, y=w2008) -> (x != y?=w2005:bool)
                n1199 = Compound Arithmetic op=AND(w2005, w2001, w2002) -> (w2003:bool)
                n1200 = case shown="True" w2003 {
                  frame False {
                  }
                  frame True {
                    "Part Number Changed" <- TRUE ("Part Number Changed")
                    "Timer 1 Stpt." <- 2 ("Timer 1 Stpt.")
                  }
                }
              }
            }
            frame #9 {
              n1201 = case shown="4" w2016 {
                tunnel: w2015 -> [_ w2034 _ _ _]
                tunnel: w2014 -> [_ _ _ w2242 w2468]
                tunnel: w2013 -> [_ _ _ w2240 _]
                frame 0, Default {
                  n1202 = global read "Schedule Control Globals.vi" "Apply to Schedule Saved"() -> (w2017:bool)
                  n1203 = case shown="True" w2017 {
                    frame False {
                    }
                    frame True {
                      n1204 = global write "Schedule Control Globals.vi" "Apply to Schedule Saved"(FALSE ("Apply to Schedule Saved")) -> ()
                      n1205 = property on="Transfer to Schedule" class="Bool"("DisabledEnum"=T5."Enabled" ("Disabled")) -> ()  [unwired: 2 in, 2 out]
                    }
                  }
                }
                frame 1 {
                  w2025 = string[] [] ("Strings []")
                  # "Start timer so reset is delayed so that the\nadd selections to worksheet can be clicked\nmultiple times."
                  # "Pick Design"
                  n1206 = local read "Coating Type 2"() -> (w2035:string)
                  n1207 = property on="Design# Match/es" class="Ring (strict)"() -> ("RingText.Text"=w2033:string)  [unwired: 2 in, 2 out]
                  n1208 = local read "Wavelength 2"() -> (w2037:string)
                  n1209 = local read "Substrate 2"() -> (w2036:string)
                  n1210 = call "Pick Thin Film Design.vi"("Design from Builder"=w2033, "Wavelength"=w2037, "Substrate"=w2036, "Coating Type"=w2035, "Read Path"=w2034) -> ("Cancel Out"=w2022:bool, "Substrate Picked"=w2024:string, "Coating Type Picked"=w2032:string, "Design Number"=w2040:string, "Wavelength Picked"=w2031:string)  [unwired: 1 in]
                  n1211 = property on="Design# Match/es" class="Ring (strict)"() -> ("Strings []"=w2038:string[])  [unwired: 2 in, 2 out]
                  n1212 = property on="Substrate" class="Ring (strict)"() -> ("Strings []"=w2021:string[])  [unwired: 2 in, 2 out]
                  n1213 = case shown="False" w2022 {
                    tunnel: w2040 -> [w2050 _]
                    tunnel: [w2049 w2056] -> w2039
                    tunnel: w2038 -> [w2048 w2056]
                    tunnel: w2032 -> [w2047 _]
                    tunnel: [w2047 w2055] -> w2029
                    tunnel: w2031 -> [w2046 _]
                    tunnel: [w2046 w2054] -> w2028
                    tunnel: w2024 -> [w2045 _]
                    tunnel: [w2045 w2053] -> w2023
                    tunnel: w2021 -> [w2043 _]
                    tunnel: [TRUE ("Pick Design was true") FALSE ("Pick Design was true")] -> w2020
                    frame False {
                      w2044 = u16 0 ("y")
                      n1214 = local write "Design# Match/es"(w2044) -> ()
                      n1215 = local write "Coating Type"(w2044) -> ()
                      n1216 = local write "Wavelength"(w2044) -> ()
                      n1217 = local write "Substrate"(w2044) -> ()
                      n1218 = Insert Into Array(array=w2048, index=0, new element=w2050) -> (w2049:string[])
                      "SubstrateStrings" <- w2043
                    }
                    frame True {
                      # "User cancelled"
                      n1219 = property on="Substrate" class="Ring (strict)"() -> ("RingText.Text"=w2053:string)  [unwired: 2 in, 2 out]
                      n1220 = property on="Coating Type" class="Ring (strict)"() -> ("RingText.Text"=w2055:string)  [unwired: 2 in, 2 out]
                      n1221 = property on="Wavelength" class="Ring (strict)"() -> ("RingText.Text"=w2054:string)  [unwired: 2 in, 2 out]
                    }
                  }
                  n1222 = local write "Pick Design was True"(w2020) -> ()
                  n1223 = case shown="True" w2020 {
                    frame False {
                    }
                    frame True {
                      # "Reset substate list after pick design."
                      n1224 = Tick Count (ms)() -> (millisecond timer value=→"Reset Substrate Timer Start":u32)
                    }
                  }
                  n1225 = property on="Design# Match/es" class="Ring (strict)"("Strings []"=w2039) -> ()  [unwired: 2 in, 2 out]
                  n1226 = Insert Into Array(array=w2025, new element=w2029) -> (w2030:string[])  [unwired: 1 in]
                  n1227 = Insert Into Array(array=w2025, new element=w2023) -> (w2026:string[])  [unwired: 1 in]
                  n1228 = Insert Into Array(array=w2025, new element=w2028) -> (w2027:string[])  [unwired: 1 in]
                  n1229 = property on="Coating Type" class="Ring (strict)"("Strings []"=w2030) -> ()  [unwired: 2 in, 2 out]
                  n1230 = property on="Substrate" class="Ring (strict)"("Strings []"=w2026) -> ()  [unwired: 2 in, 2 out]
                  n1231 = property on="Wavelength" class="Ring (strict)"("Strings []"=w2027) -> ()  [unwired: 2 in, 2 out]
                }
                frame 2 {
                  # "Add to Worksheet"
                  n1232 = local read "Lookup was True"() -> (w2066:bool)
                  n1233 = local read "Part No Found"() -> (w2067:bool)
                  n1234 = local read "Part Number"() -> (w2059:string)
                  n1235 = local read "Work Order"() -> (w2060:string)
                  n1236 = local read "Pick Design was True"() -> (w2062:bool)
                  n1237 = local read "Diameter"() -> (w2061:string)
                  n1238 = local read "Qty"() -> (w2058:string)
                  n1239 = property on="Substrate" class="Ring (strict)"() -> ("Ring Text.Text"=w2068:string)  [unwired: 2 in, 2 out]
                  n1240 = property on="Coating Type" class="Ring (strict)"() -> ("Ring Text.Text"=w2069:string)  [unwired: 2 in, 2 out]
                  n1241 = property on="Wavelength" class="Ring (strict)"() -> ("Ring Text.Text"=w2071:string)  [unwired: 2 in, 2 out]
                  n1242 = property on="Design# Match/es" class="Ring (strict)"() -> ("Ring Text.Text"=w2070:string)  [unwired: 2 in, 2 out]
                  n1243 = Build Array(w2066, w2067, "Select Action") -> (w2065:bool[])
                  n1244 = Build Array(w2061, w2060, w2059, w2058) -> (w2057:string[])
                  n1245 = Boolean Array To Number(Boolean array=w2065) -> (number=w2064:u32)
                  n1246 = case shown="6, 7" w2064 {
                    tunnel: w2068 -> [w2077 w2140 _ w2160 w2205]
                    tunnel: w2069 -> [w2076 w2139 _ w2159 w2204]
                    tunnel: w2070 -> [w2075 w2138 _ w2158 w2203]
                    tunnel: w2071 -> [w2074 _ _ _ _]
                    tunnel: w2062 -> [_ w2136 _ w2156 _]
                    tunnel: w2057 -> [w2073 w2135 _ w2155 _]
                    frame 0, Default {
                      # "Lookup not true, just use manual inputs and replace the selected row"
                      n1247 = stacked-sequence {
                        seq-local: [w2084 _] -> [_ w2103]
                        seq-local: [w2087 _] -> [_ w2102]
                        seq-local: [w2088 _] -> [_ w2101]
                        tunnel: w2077 -> [_ w2107]
                        tunnel: w2076 -> [_ w2106]
                        tunnel: w2075 -> [_ w2105]
                        tunnel: w2074 -> [_ w2104]
                        tunnel: w2073 -> [_ w2100]
                        frame #0 {
                          # "Check if row blank"
                          n1248 = local read "Edit Position 2"() -> (w2078:T1)
                          n1249 = local read "Run Worksheet"() -> (w2087:string[][])
                          n1250 = Array Size(array=w2087) -> (size(s)=w2086:i32[])
                          n1251 = Unbundle(w2078) -> ("Row"=w2084:i32)  [unwired: 1 out]
                          n1252 = Index Array(array=w2086, index=0) -> (element=w2083:i32)
                          n1253 = Index Array(array=w2087, index (row)=w2084) -> (element=w2091:string[])  [unwired: 1 in]
                          n1254 = Greater Or Equal?(x=w2084, y=w2083) -> (x >= y?=w2081:bool)
                          n1255 = Index Array(array=w2091, index=1) -> (element=w2089:string)
                          n1256 = Not Equal?(x=w2089, y="") -> (x != y?=w2082:bool)
                          n1257 = Build Array(w2082, w2081) -> (w2080:bool[])
                          n1258 = Boolean Array To Number(Boolean array=w2080) -> (number=w2079:u32)
                          n1259 = case shown="0, Default" w2079 {
                            tunnel: [TRUE ("T button?") w2094 w2096] -> w2088
                            frame 0, Default {
                            }
                            frame 1 {
                              n1260 = Two Button Dialog(message="Data Exists at this row.  Do you want to over-write?") -> (T button?=w2094:bool)  [unwired: 2 in]
                            }
                            frame 2 {
                              n1261 = One Button Dialog(message="The selected row is past the end of the sheet.  To put data there, insert a new row or rows first...") -> (true=w2097:bool)  [unwired: 1 in]
                              n1262 = Not(x=w2097) -> (.not. x?=w2096:bool)
                            }
                          }
                        }
                        frame #1 {
                          # "Add new selections to the worksheet"
                          n1263 = case shown="True" w2101 {
                            tunnel: w2107 -> [_ w2128]
                            tunnel: w2106 -> [_ w2127]
                            tunnel: w2105 -> [_ w2126]
                            tunnel: w2104 -> [_ w2125]
                            tunnel: w2103 -> [_ w2110]
                            tunnel: w2102 -> [_ w2120]
                            tunnel: w2100 -> [_ w2122]
                            tunnel: "Include WO & PN" -> [_ w2123]
                            frame False {
                              # "User Cancelled or end of sheet error"
                            }
                            frame True {
                              w2124 = ""
                              # "Side #"
                              n1264 = Index Array(array=w2120, index (row) #1=w2110, index (col) #1=4 ("disabled index (col)"), index (row) #2=w2110, index (col) #2=5 ("disabled index (col)"), index (row) #3=w2110, index (col) #3=6 ("disabled index (col)"), index (row) #4=w2110, index (col) #4=7 ("disabled index (col)"), index (row) #5=w2110, index (col) #5=8 ("disabled index (col)")) -> (element #1=w2115:string, element #2=w2114:string, element #3=w2113:string, element #4=w2112:string, element #5=w2108:string)
                              n1265 = Build Array(w2115, w2114, w2113, w2112) -> (w2111:string[])
                              n1266 = case shown="True" w2123 {
                                tunnel: w2122 -> [_ w2133]
                                tunnel: [w2131 w2133] -> w2121
                                tunnel: w2111 -> [w2131 _]
                                frame False {
                                }
                                frame True {
                                n1267 = local write "Include WO & PN"(FALSE ("Include WO & PN")) -> ()
                                }
                              }
                              n1268 = Build Array (concatenate)(w2128, w2127, w2125, w2126, w2121, w2108, w2124, w2124, w2124) -> (w2129:string[])
                              n1269 = Replace Array Subset(array=w2120, new element=w2129, index (row)=w2110) -> (w2130:string[][])  [unwired: 1 in]
                              n1270 = local write "Run Worksheet"(w2130) -> ()
                            }
                          }
                        }
                      }
                    }
                    frame 1 {
                      w2134 = ""
                      # "Lookup was true but part number not found.  Take whatever data can be used from the Workcenter Report and insert at the end of the worksheet."
                      n1271 = local read "Wavelength 2"() -> (w2144:string)
                      n1272 = Concatenate Strings(w2144, " µm" ("string")) -> (w2145:string)
                      n1273 = local write "Lookup was True"(FALSE ("Lookup was True")) -> ()
                      n1274 = Build Array (concatenate)(w2140, w2139, w2145, w2138, w2135, w2134, w2134, w2134, w2134) -> (w2141:string[])
                      n1275 = case shown="True" w2136 {
                        frame False {
                        }
                        frame True {
                          # "Reset substate list after pick design."
                          n1276 = local read "SubstrateStrings"() -> (w2148:string[])
                          n1277 = local write "Pick Design was True"(FALSE ("Pick Design was true")) -> ()
                          n1278 = property on="Substrate" class="Ring (strict)"("Strings []"=w2148) -> ()  [unwired: 2 in, 2 out]
                        }
                      }
                      n1279 = local read "Run Worksheet"() -> (w2142:string[][])
                      n1280 = Insert Into Array(array=w2142, new element=w2141) -> (w2143:string[][])  [unwired: 2 in]
                      n1281 = local write "Run Worksheet"(w2143) -> ()
                    }
                    frame 2, 3 {
                      w2152 = FALSE ("Lookup was True")
                      # "Part number was found, lookup Don't care.  get part history data and add to the worksheet at the end"
                      n1282 = local read "Worksheet array"() -> (w2151:string[])
                      n1283 = Array Subset(array=w2151, length=13) -> (w2149:string[])  [unwired: 1 in]
                      n1284 = local read "Run Worksheet"() -> (w2154:string[][])
                      n1285 = local write "Lookup was True"(w2152) -> ()
                      n1286 = local write "Part No Found"(w2152) -> ()
                      n1287 = Insert Into Array(array=w2154, new element=w2149) -> (w2153:string[][])  [unwired: 2 in]
                      n1288 = local write "Run Worksheet"(w2153) -> ()
                    }
                    frame 5 {
                      # "Lookup was true but part number not found.  Select Action = True.  Take whatever data can be used from the Workcenter Report and insert one row down from the current edit position."
                      n1289 = stacked-sequence {
                        seq-local: [_ _ w2177 _] -> [_ _ _ w2189]
                        seq-local: [w2163 _ _ _] -> [_ w2172 w2175 _]
                        seq-local: [w2162 _ _ _] -> [_ w2171 _ _]
                        tunnel: w2160 -> [_ _ _ w2184]
                        tunnel: w2159 -> [_ _ _ w2186]
                        tunnel: w2158 -> [_ _ _ w2188]
                        tunnel: w2156 -> [_ _ _ w2181]
                        tunnel: w2155 -> [_ _ _ w2180]
                        frame #0 {
                          # "Check if valid row"
                          n1290 = local read "Run Worksheet"() -> (w2162:string[][])
                          n1291 = local read "Edit Position 2"() -> (w2164:T1)
                          n1292 = Array Size(array=w2162) -> (size(s)=w2167:i32[])
                          n1293 = Unbundle(w2164) -> ("Row"=w2163:i32)  [unwired: 1 out]
                          n1294 = Index Array(array=w2167, index=0) -> (element=w2165:i32)
                          n1295 = Greater Or Equal?(x=w2163, y=w2165) -> (x >= y?=w2161:bool)
                          n1296 = case shown="True" w2161 {
                            frame False {
                            }
                            frame True {
                              n1297 = stacked-sequence {
                                frame #0 {
                                n1298 = One Button Dialog(message="The selected row is past the end of the sheet.  To put data there, uncheck the \"Select Action\" box on the Workcenter Report tab.") -> ()  [unwired: 1 in, 1 out]
                                }
                                frame #1 {
                                n1299 = local write "Tab Control"(enum32{"Workcenter Report", "Run Worksheet"}."Workcenter Report" ("Tab Control")) -> ()
                                }
                              }
                            }
                          }
                        }
                        frame #1 {
                          # "insert a row after the current edit position"
                          n1300 = Increment(x=w2172) -> (x+1=w2173:i32)
                          n1301 = Insert Into Array(array=w2171, index (row)=w2173, new element=string[] ["", "", "", "", "", "", "", "", "", "", "", ""] ("Build Schedule Table")) -> (w2174:string[][])  [unwired: 1 in]
                          n1302 = local write "Run Worksheet"(w2174) -> ()
                        }
                        frame #2 {
                          # "increment Edit Position"
                          n1303 = Increment(x=w2175) -> (x+1=w2177:i32)
                          n1304 = Bundle(w2177, "x+1"=3) -> (w2176:cluster{i32, "x+1":i32})  [unwired: 1 in]
                          n1305 = local write "Edit Position 2"(w2176) -> ()
                          n1306 = property on="Run Worksheet" class="Tbl (strict)"("EditPos"=w2176) -> ()  [unwired: 2 in, 2 out]
                        }
                        frame #3 {
                          w2179 = ""
                          # "Place data one row down"
                          n1307 = local read "Select Action 2"() -> (w2182:bool)
                          n1308 = case shown="True" w2182 {
                            tunnel: [w2199 w2201] -> w2193
                            tunnel: w2188 -> [w2197 _]
                            tunnel: [w2197 w2201] -> w2187
                            tunnel: w2186 -> [w2196 _]
                            tunnel: [w2196 w2201] -> w2185
                            tunnel: w2184 -> [w2195 _]
                            tunnel: [w2195 w2201] -> w2183
                            frame False {
                              n1309 = local read "Wavelength 2"() -> (w2198:string)
                              n1310 = Concatenate Strings(w2198, " µm" ("string")) -> (w2199:string)
                            }
                            frame True {
                              w2201 = ""
                            }
                          }
                          n1311 = Build Array (concatenate)(w2183, w2185, w2193, w2187, w2180, w2179, w2179, w2179) -> (w2190:string[])
                          n1312 = case shown="True" w2181 {
                            frame False {
                            }
                            frame True {
                              # "Reset substate list after pick design."
                              n1313 = local read "SubstrateStrings"() -> (w2194:string[])
                              n1314 = property on="Substrate" class="Ring (strict)"("Strings []"=w2194) -> ()  [unwired: 2 in, 2 out]
                            }
                          }
                          n1315 = local read "Run Worksheet"() -> (w2191:string[][])
                          n1316 = Replace Array Subset(array=w2191, new element=w2190, index (row)=w2189) -> (w2192:string[][])  [unwired: 1 in]
                          n1317 = local write "Run Worksheet"(w2192) -> ()
                        }
                      }
                      n1318 = local write "Lookup was True"(FALSE ("Lookup was True")) -> ()
                    }
                    frame 6, 7 {
                      # "Part number found. Lookup don't care. Select Action true.  Take data from the Workcenter Report and insert one row down from the current edit position."
                      n1319 = stacked-sequence {
                        seq-local: [_ _ w2222 _] -> [_ _ _ w2227]
                        seq-local: [w2208 _ _ _] -> [_ w2217 w2220 _]
                        seq-local: [w2207 _ _ _] -> [_ w2216 _ _]
                        tunnel: w2205 -> [_ _ _ _]
                        tunnel: w2204 -> [_ _ _ _]
                        tunnel: w2203 -> [_ _ _ _]
                        frame #0 {
                          # "Check if valid row"
                          n1320 = local read "Run Worksheet"() -> (w2207:string[][])
                          n1321 = local read "Edit Position 2"() -> (w2209:T1)
                          n1322 = Array Size(array=w2207) -> (size(s)=w2212:i32[])
                          n1323 = Unbundle(w2209) -> ("Row"=w2208:i32)  [unwired: 1 out]
                          n1324 = Index Array(array=w2212, index=0) -> (element=w2210:i32)
                          n1325 = Greater Or Equal?(x=w2208, y=w2210) -> (x >= y?=w2206:bool)
                          n1326 = case shown="True" w2206 {
                            frame False {
                            }
                            frame True {
                              n1327 = stacked-sequence {
                                frame #0 {
                                n1328 = One Button Dialog(message="The selected row is past the end of the sheet.  To put data there, uncheck the \"Select Action\" box on the Workcenter Report tab.") -> ()  [unwired: 1 in, 1 out]
                                }
                                frame #1 {
                                n1329 = local write "Tab Control"(enum32{"Workcenter Report", "Run Worksheet"}."Workcenter Report" ("Tab Control")) -> ()
                                }
                              }
                            }
                          }
                        }
                        frame #1 {
                          # "insert a row after the current edit position"
                          n1330 = Increment(x=w2217) -> (x+1=w2218:i32)
                          n1331 = Insert Into Array(array=w2216, index (row)=w2218, new element=string[] ["", "", "", "", "", "", "", "", "", "", "", ""] ("Build Schedule Table")) -> (w2219:string[][])  [unwired: 1 in]
                          n1332 = local write "Run Worksheet"(w2219) -> ()
                        }
                        frame #2 {
                          # "increment Edit Position"
                          n1333 = Increment(x=w2220) -> (x+1=w2222:i32)
                          n1334 = Bundle(w2222, "x+1"=3) -> (w2221:cluster{i32, "x+1":i32})  [unwired: 1 in]
                          n1335 = local write "Edit Position 2"(w2221) -> ()
                          n1336 = property on="Run Worksheet" class="Tbl (strict)"("EditPos"=w2221) -> ()  [unwired: 2 in, 2 out]
                        }
                        frame #3 {
                          # "Place data one row down"
                          n1337 = local read "Worksheet array"() -> (w2226:string[])
                          n1338 = case shown="True" "Select Action 2" {
                            tunnel: [w2231 w2235] -> w2224
                            tunnel: w2226 -> [w2230 w2239]
                            frame False {
                              # "Add all Data"
                              n1339 = Array Subset(array=w2230, length=13) -> (w2231:string[])  [unwired: 1 in]
                            }
                            frame True {
                              # "Add partial data"
                              n1340 = Array Subset(array=w2239, index=4, length=4) -> (w2236:string[])
                              n1341 = Insert Into Array(array=w2236, index=0, new element=string[] ["", "", "", ""] ("new element/subarray")) -> (w2235:string[])
                            }
                          }
                          n1342 = local read "Run Worksheet"() -> (w2228:string[][])
                          n1343 = Replace Array Subset(array=w2228, new element=w2224, index (row)=w2227) -> (w2229:string[][])  [unwired: 1 in]
                          n1344 = local write "Run Worksheet"(w2229) -> ()
                        }
                      }
                      n1345 = local write "Lookup was True"(FALSE ("Lookup was True")) -> ()
                    }
                  }
                  n1346 = local write "Add to Worksheet"(FALSE ("Add to Worksheet")) -> ()
                }
                frame 4 {
                  # "Individual System Schedule indexes\n2-Substrate\n3-Coating Type\n4-Wavelength\n5-Diameter\n6-Design Number\n11-Coating Time\n12-Setup Time\n13-Pump Down Time\n14-Total Time"
                  # "Transfer Selected Row to Schedule"
                  n1347 = local read "Edit Position 2"() -> (w2241:T1)
                  n1348 = local read "Run Worksheet"() -> (w2244:string[][])
                  n1349 = property on="System Select" class="Ring (strict)"() -> ("Ring Text.Text"=w2246:string)  [unwired: 2 in, 2 out]
                  n1350 = Unbundle(w2241) -> ("Row"=w2245:i32)  [unwired: 1 out]
                  n1351 = Index Array(array=w2244, index (row)=w2245) -> (element=w2243:string[])  [unwired: 1 in]
                  n1352 = stacked-sequence {
                    seq-local: [w2249 _ _ _ _ _ _ _] -> [_ _ _ _ w2410 _ _ _]
                    seq-local: [w2248 _ _ _ _ _ _ _] -> [_ w2280 w2300 _ _ _ _ _]
                    seq-local: [_ _ _ _ _ _ w2424 _] -> [_ _ _ _ _ _ _ w2438]
                    seq-local: [_ w2267 _ _ _ _ _ _] -> [_ _ w2298 _ _ _ _ _]
                    seq-local: [_ _ _ w2369 _ _ _ _] -> [_ _ _ _ w2404 _ _ _]
                    seq-local: [_ _ _ w2368 _ _ _ _] -> [_ _ _ _ w2407 _ _ _]
                    seq-local: [_ _ w2299 _ _ _ _ _] -> [_ _ _ _ _ _ _ _]
                    seq-local: [_ _ _ _ _ w2415 _ _] -> [_ _ _ _ _ _ w2423 w2436]
                    seq-local: [_ _ _ _ _ _ w2422 _] -> [_ _ _ _ _ _ _ w2435]
                    tunnel: w2243 -> [w2254 _ w2294 _ w2401 _ _ w2437]
                    tunnel: w2242 -> [_ w2286 w2295 w2376 _ _ w2425 w2439]
                    tunnel: w2245 -> [_ _ _ _ w2408 w2417 _ w2434]
                    tunnel: w2244 -> [_ _ _ _ w2413 w2419 _ _]
                    tunnel: w2246 -> [_ w2284 _ w2374 _ _ _ w2433]
                    tunnel: w2240 -> [_ w2261 _ _ _ _ _ _]
                    frame #0 {
                      # "Substrate\nCoating type\nWavelength\nDesign number\nDiameter"
                      # "Put info from Run Worksheet to Selected row global"
                      n1353 = Index Array(array=w2254) -> (element #1=w2253:string, element #2=w2252:string, element #3=w2251:string, element #4=w2248:string, element #5=w2250:string)  [unwired: 5 in]
                      n1354 = property on="Transfer to Schedule" class="Bool"("DisabledEnum"=T5."Disabled and Grayed Out" ("Disabled")) -> ()  [unwired: 2 in, 2 out]
                      n1355 = Build Array(w2253, w2252, w2251, w2250, w2248) -> (w2249:string[])
                    }
                    frame #1 {
                      w2263 = i16 2 ("precision (6)")
                      # "Setup Time"
                      # "Design Number"
                      # "Coating Time"
                      # "Total Time"
                      # "Pump Time"
                      # "Get times from system data first.  If not found, try complete design info table."
                      # "Coating Time\nSetup Time\nPump Down Time\nTotal Time"
                      n1356 = Path To String(path=w2286) -> (string=w2287:string)
                      n1357 = Fract/Exp String To Number(string=w2261) -> (number=w2258:dbl)  [unwired: 3 in, 1 out]
                      n1358 = Multiply(x=w2258, y=60.0) -> (x*y=w2257:dbl)
                      n1359 = Concatenate Strings(w2287, "\\Designs by System" ("string"), "\\" ("string"), "Sys " ("string"), w2284, " Run Times.txt" ("string")) -> (w2289:string)
                      n1360 = String To Path(string=w2289) -> (path=w2256:path)
                      n1361 = call-poly <vilib>:"Read Delimited Spreadsheet.vi"("file path (dialog if empty)"=w2256) -> ("all rows"=w2255:string[][])  [unwired: 9 in, 5 out]
                      n1362 = Number To Fractional String(number=w2257) -> (F-format string=w2259:string)  [unwired: 3 in]
                      n1363 = Index Array(array=w2255, index (col)=0 ("disabled index (col)")) -> (element=w2281:string[])  [unwired: 1 in]
                      n1364 = To Upper Case(1:w2281) -> (0:w2279:string[])
                      n1365 = To Upper Case(1:w2280) -> (0:w2278:string)
                      n1366 = Search 1D Array(1D array=w2279, element=w2278) -> (index of element=w2269:i32)  [unwired: 1 in]
                      n1367 = Equal?(x=w2269, y=-1) -> (x = y?=w2267:bool)
                      n1368 = Index Array(array=w2255, index (row) #1=w2269, index (col) #1=1 ("disabled index (col)"), index (row) #2=w2269, index (col) #2=2 ("disabled index (col)")) -> (element #1=w2272:string, element #2=w2266:string)
                      n1369 = Fract/Exp String To Number(string=w2272) -> (number=w2275:dbl)  [unwired: 3 in, 1 out]
                      n1370 = Fract/Exp String To Number(string=w2266) -> (number=w2265:dbl)  [unwired: 3 in, 1 out]
                      n1371 = Subtract(x=w2265, y=w2275) -> (x-y=w2274:dbl)
                      n1372 = Add(x=w2265, y=w2257) -> (x+y=w2264:dbl)
                      n1373 = Number To Fractional String(number=w2274, precision (6)=w2263) -> (F-format string=w2273:string)  [unwired: 2 in]
                      n1374 = Number To Fractional String(number=w2264, precision (6)=w2263) -> (F-format string=w2262:string)  [unwired: 2 in]
                      n1375 = Build Array(w2273, w2259, w2272, w2262) -> (w2271:string[])
                      n1376 = for {
                        tunnel: w2271 -> [w2293] mode=indexing
                        tunnel: [w2291] -> w2270 mode=indexing
                        n1377 = Fract/Exp String To Number(string=w2293) -> (number=w2292:dbl)  [unwired: 3 in, 1 out]
                        n1378 = call "Minutes to Hour - Min.vi"("Minutes"=w2292) -> ("H:M"=w2291:string)
                      }
                      "Time Array" <- w2270
                    }
                    frame #2 {
                      n1379 = global read "Schedule Control Globals.vi" "Ref Select"() -> (w2296:bool)
                      n1380 = Or(x=w2296, y=w2298) -> (x .or. y?=w2297:bool)
                      n1381 = case shown="True" w2297 {
                        tunnel: w2300 -> [_ w2304]
                        tunnel: [_ w2303] -> w2299
                        tunnel: w2295 -> [_ w2302]
                        tunnel: w2294 -> [_ w2301]
                        frame False {
                          # "Design found by system or a design reference sheet is being used."
                        }
                        frame True {
                          n1382 = stacked-sequence {
                            seq-local: [_ w2314 _] -> [_ _ w2340]
                            seq-local: [_ w2313 _] -> [_ _ w2338]
                            seq-local: [w2305 _ _] -> [_ w2312 _]
                            tunnel: w2304 -> [_ w2324 _]
                            tunnel: [_ w2323 _] -> w2303
                            tunnel: w2302 -> [w2306 _ w2337]
                            tunnel: w2301 -> [_ _ w2336]
                            frame #0 {
                              # "Read in Design Info Table"
                              n1383 = Path To String(path=w2306) -> (string=w2309:string)
                              n1384 = Concatenate Strings(w2309, "\\" ("string"), "Design Info.txt" ("string")) -> (w2310:string)
                              n1385 = String To Path(string=w2310) -> (path=w2311:path)
                              n1386 = call-poly <vilib>:"Read Delimited Spreadsheet.vi"("file path (dialog if empty)"=w2311) -> ("all rows"=w2305:string[][])  [unwired: 9 in, 5 out]
                            }
                            frame #1 {
                              # "Design not found by system look in the Design info table for the times"
                              # "Coating Time\nSetup Time\nPump Down Time\nTotal Time"
                              n1387 = Index Array(array=w2312, index (col)=3 ("disabled index (col)")) -> (element=w2329:string[])  [unwired: 1 in]
                              n1388 = Search 1D Array(1D array=w2329, element=w2324) -> (index of element=w2323:i32)  [unwired: 1 in]
                              n1389 = Index Array(array=w2312, index (row) #1=w2323, index (col) #1=4 ("disabled index (col)"), index (row) #2=w2323, index (col) #2=5 ("disabled index (col)"), index (row) #3=w2323, index (col) #3=6 ("disabled index (col)"), index (row) #4=w2323, index (col) #4=7 ("disabled index (col)")) -> (element #1=w2319:string, element #2=w2320:string, element #3=w2321:string, element #4=w2322:string)
                              n1390 = Build Array(w2319, w2320, w2321, w2322) -> (w2318:string[])
                              n1391 = for {
                                tunnel: w2318 -> [w2333] mode=indexing
                                tunnel: [w2332] -> w2313 mode=indexing
                                tunnel: [w2331] -> w2317 mode=indexing
                                n1392 = Fract/Exp String To Number(string=w2333) -> (number=w2335:dbl)  [unwired: 3 in, 1 out]
                                n1393 = Multiply(x=w2335, y=60.0) -> (x*y=w2331:dbl)
                                n1394 = call "Minutes to Hour - Min.vi"("Minutes"=w2331) -> ("H:M"=w2332:string)
                              }
                              n1395 = Add Array Elements(numeric array=w2317) -> (sum=w2316:dbl)
                              n1396 = Less Or Equal?(x=w2316, y=1.0) -> (x <= y?=w2314:bool)
                            }
                            frame #2 {
                              n1397 = case shown="True" w2340 {
                                tunnel: [w2341 w2347] -> w2339
                                tunnel: w2338 -> [w2341 w2349]
                                tunnel: w2337 -> [_ w2359]
                                tunnel: w2336 -> [_ w2358]
                                frame False {
                                }
                                frame True {
                                # "Total Time"
                                # "Part number of transfer row"
                                # "No time info, get from part info"
                                n1398 = Index Array(array=w2358, index=6) -> (element=w2354:string)
                                n1399 = Path To String(path=w2359) -> (string=w2362:string)
                                n1400 = Concatenate Strings(w2362, "\\Part Number Info.txt" ("string")) -> (w2360:string)
                                n1401 = String To Path(string=w2360) -> (path=w2343:path)
                                n1402 = call-poly <vilib>:"Read Delimited Spreadsheet.vi"("file path (dialog if empty)"=w2343) -> ("all rows"=w2342:string[][])  [unwired: 9 in, 5 out]
                                n1403 = To Upper Case(1:w2354) -> (0:w2353:string)
                                n1404 = Index Array(array=w2342, index (col) #1=0 ("disabled index (col)"), index (col) #2=2 ("index (col)")) -> (element #1=w2355:string[], element #2=w2350:string[])  [unwired: 2 in]
                                n1405 = To Upper Case(1:w2355) -> (0:w2352:string[])
                                n1406 = Search 1D Array(1D array=w2352, element=w2353) -> (index of element=w2346:i32)  [unwired: 1 in]
                                n1407 = Not Equal?(x=w2346, y=-1) -> (x != y?=w2344:bool)
                                n1408 = Index Array(array=w2350, index=w2346) -> (element=w2348:string)
                                n1409 = case shown="True" w2344 {
                                tunnel: w2349 -> [w2363 w2367]
                                tunnel: w2348 -> [_ w2366]
                                tunnel: [w2363 w2365] -> w2347
                                frame False {
                                }
                                frame True {
                                n1410 = Replace Array Subset(array=w2367, new element=w2366, index=3) -> (w2365:string[])
                                }
                                }
                                }
                              }
                              n1411 = local write "Time Array"(w2339) -> ()
                            }
                          }
                        }
                      }
                    }
                    frame #3 {
                      # "Get Run ID, if no file create new"
                      n1412 = Path To String(path=w2376) -> (string=w2377:string)
                      n1413 = Concatenate Strings(w2377, "\\Run Worksheets\\Run ID Tracking\\" ("string"), w2374, "\\" ("string"), "Run ID #.txt" ("string")) -> (w2378:string)
                      n1414 = String To Path(string=w2378) -> (path=w2368:path)
                      n1415 = File/Directory Info(path=w2368) -> (error out=w2371:errorcluster)  [unwired: 1 in, 6 out]
                      n1416 = Unbundle By Name(w2371) -> ("code"=w2370:i32)
                      n1417 = case shown="0" w2370 {
                        tunnel: w2368 -> [w2382 _ w2385]
                        tunnel: [w2379 1 w2384] -> w2369
                        frame 0 {
                          n1418 = call <vilib>:"Read Characters From File.vi"("file path (dialog if empty)"=w2382) -> ("character string"=w2380:string)  [unwired: 5 in, 3 out]
                          n1419 = Decimal String To Number(string=w2380) -> (number=w2381:i32)  [unwired: 2 in, 1 out]
                          n1420 = Increment(x=w2381) -> (x+1=w2379:i32)
                        }
                        frame 1, Default {
                          # "Unknown Error"
                        }
                        frame 7 {
                          # "No File, Create new"
                          n1421 = stacked-sequence {
                            tunnel: w2385 -> [w2388 w2390 w2392]
                            tunnel: [_ _ 1] -> w2384
                            frame #0 {
                              n1422 = Strip Path(path=w2388) -> (stripped path=w2387:path)  [unwired: 1 out]
                              n1423 = Strip Path(path=w2387) -> (stripped path=w2386:path)  [unwired: 1 out]
                              n1424 = Create Folder(path (use dialog)=w2386) -> ()  [unwired: 2 in, 3 out]
                            }
                            frame #1 {
                              n1425 = Strip Path(path=w2390) -> (stripped path=w2389:path)  [unwired: 1 out]
                              n1426 = Create Folder(path (use dialog)=w2389) -> ()  [unwired: 2 in, 3 out]
                            }
                            frame #2 {
                              n1427 = Write to Text File(file (use dialog)=w2392, text="0" ("character string")) -> ()  [unwired: 2 in, 3 out]
                            }
                          }
                        }
                      }
                    }
                    frame #4 {
                      # "Run ID (Row#)"
                      n1428 = Greater?(x=w2404, y=999) -> (0:w2405:bool)
                      n1429 = Select(t=1, s=w2405, f=w2404) -> (s? t:f=w2402:i32)
                      n1430 = Number To Decimal String(number=w2402) -> (decimal integer string=w2396:string)  [unwired: 1 in]
                      n1431 = Replace Array Subset(array=w2413, new element=w2396, index (row)=w2408, index (col)=10 ("disabled index (col)")) -> (w2411:string[][])
                      n1432 = Write to Text File(file (use dialog)=w2407, text=w2396) -> ()  [unwired: 2 in, 3 out]
                      n1433 = local write "Run Worksheet"(w2411) -> ()
                      n1434 = local read "Time Array"() -> (w2409:string[])
                      n1435 = Index Array(array=w2401, index #1=9 ("index"), index #2=11 ("index"), index #3=12 ("index")) -> (element #1=w2399:string, element #2=w2397:string, element #3=w2394:string)
                      n1436 = Build Array (concatenate)(w2410, w2409, w2396, w2399, w2397, w2394) -> (w2414:string[])
                      n1437 = global write "Schedule Control Globals.vi" "Transfer Array"(w2414) -> ()
                    }
                    frame #5 {
                      # "Check if required data exits for part number tracking update"
                      # "Substrate"
                      n1438 = Index Array(array=w2419, index (row)=w2417, index (col)=0 ("index")) -> (element=w2420:string)
                      n1439 = Not Equal?(x=w2420, y="") -> (x != y?=w2415:bool)
                      n1440 = global write "Schedule Control Globals.vi" "Apply to Schedule"(TRUE ("Apply to Schedule")) -> ()
                    }
                    frame #6 {
                      n1441 = case shown="True" w2423 {
                        tunnel: w2425 -> [_ w2428]
                        tunnel: [_ w2426] -> w2424
                        tunnel: [_ w2427] -> w2422
                        frame False {
                          # "Blank Substrate"
                        }
                        frame True {
                          # "get part number info"
                          n1442 = Path To String(path=w2428) -> (string=w2431:string)
                          n1443 = Concatenate Strings(w2431, "\\Part Number Info.txt" ("string")) -> (w2429:string)
                          n1444 = String To Path(string=w2429) -> (path=w2427:path)
                          n1445 = call-poly <vilib>:"Read Delimited Spreadsheet.vi"("file path (dialog if empty)"=w2427) -> ("all rows"=w2426:string[][])  [unwired: 9 in, 5 out]
                        }
                      }
                    }
                    frame #7 {
                      # "Save Part info"
                      n1446 = case shown="True" w2436 {
                        tunnel: w2439 -> [_ w2464]
                        tunnel: w2438 -> [_ w2463]
                        tunnel: w2437 -> [_ _]
                        tunnel: w2435 -> [_ _]
                        tunnel: w2434 -> [_ w2445]
                        tunnel: w2433 -> [_ w2461]
                        frame False {
                          # "Blank Substrate"
                        }
                        frame True {
                          w2455 = "S2" ("regular expression")
                          w2456 = "S1" ("regular expression")
                          # "Process part numbers for transfer"
                          n1447 = local read "Run Worksheet"() -> (w2442:string[][])
                          n1448 = Index Array(array=w2442, index (row) #1=w2445, index (col) #1=0 ("disabled index (col)"), index (row) #2=w2445, index (col) #2=8 ("index (col)")) -> (element #1=w2459:string, element #2=w2454:string)
                          n1449 = local read "Time Array"() -> (w2462:string[])
                          n1450 = To Upper Case(1:w2454) -> (0:w2440:string)
                          n1451 = Match Pattern(string=w2440, regular expression=w2456) -> (match substring=w2457:string)  [unwired: 1 in, 3 out]
                          n1452 = Match Pattern(string=w2440, regular expression=w2455) -> (match substring=w2453:string)  [unwired: 1 in, 3 out]
                          n1453 = Equal?(x=w2457, y=w2456) -> (x = y?=w2450:bool)
                          n1454 = Equal?(x=w2453, y=w2455) -> (x = y?=w2452:bool)
                          n1455 = Or(x=w2450, y=w2452) -> (x .or. y?=w2451:bool)
                          n1456 = case shown="False" w2451 {
                            tunnel: w2459 -> [w2466 _]
                            tunnel: [w2465 w2467] -> w2446
                            tunnel: w2450 -> [_ w2467]
                            frame False {
                              n1457 = call "S1 - S2 Select.vi"("Substrate"=w2466) -> ("S1 (T) or S2?"=w2465:bool)  [unwired: 9 in, 1 out]
                            }
                            frame True {
                            }
                          }
                          n1458 = call "Process Part Numbers in Transfer.vi"("S1 (T) or S2?"=w2446, "Always Sched. w/o OverWrite"="Always Sched. w/o OverWrite", "Time Array"=w2462, "Run Worksheet"=w2442, "System No."=w2461, "Edit Row"=w2445, "Part No Info"=w2463, "Data Path"=w2464) -> ()  [unwired: 4 in]
                          n1459 = Select(t="S1" ("regular expression"), s=w2446, f="S2" ("regular expression")) -> (s? t:f=w2443:string)
                          n1460 = Replace Array Subset(array=w2442, new element=w2443, index (row)=w2445, index (col)=8 ("disabled index (col)")) -> (w2449:string[][])
                          n1461 = local write "Run Worksheet"(w2449) -> ()
                        }
                      }
                      "Transfer was True" <- TRUE ("Transfer was True")
                    }
                  }
                }
                frame 8 {
                  # "move selected row to a different system's worksheet"
                  n1462 = stacked-sequence {
                    seq-local: [w2471 _ _ _ _] -> [_ _ _ _ w2512]
                    seq-local: [w2470 _ _ _ _] -> [_ w2477 w2492 _ _]
                    seq-local: [w2469 _ _ _ _] -> [_ w2475 w2491 _ w2510]
                    seq-local: [_ w2473 _ _ _] -> [_ _ w2493 w2499 _]
                    seq-local: [_ _ _ w2498 _] -> [_ _ _ _ w2514]
                    seq-local: [_ _ _ w2497 _] -> [_ _ _ _ w2511]
                    tunnel: w2468 -> [_ _ _ _ w2513]
                    frame #0 {
                      # "get selected row"
                      n1463 = local read "Edit Position 2"() -> (w2472:T1)
                      n1464 = local read "Run Worksheet"() -> (w2470:string[][])
                      n1465 = Unbundle(w2472) -> ("Row"=w2469:i32)  [unwired: 1 out]
                      n1466 = Index Array(array=w2470, index (row)=w2469) -> (element=w2471:string[])  [unwired: 1 in]
                    }
                    frame #1 {
                      # "Check if below \"to be scheduled\""
                      n1467 = Index Array(array=w2477, index (col)=1 ("disabled index (col)")) -> (element=w2478:string[])  [unwired: 1 in]
                      n1468 = To Upper Case(1:w2478) -> (0:w2476:string[])
                      n1469 = for {
                        tunnel: w2476 -> [w2488] mode=indexing
                        tunnel: "SCHEDULED" ("element") -> [w2486]
                        shift-right: [w2483] -> w2474
                        shift-left: -1 ("to be scheduled row") -> [w2484]
                        i -> [w2482]
                        n1470 = Match Pattern(string=w2488, regular expression=w2486) -> (match substring=w2487:string)  [unwired: 1 in, 3 out]
                        n1471 = Equal?(x=w2487, y=w2486) -> (x = y?=w2485:bool)
                        n1472 = case shown="False" w2485 {
                          tunnel: [w2489 w2490] -> w2483
                          tunnel: w2484 -> [w2489 _]
                          tunnel: w2482 -> [_ w2490]
                          frame False {
                          }
                          frame True {
                          }
                        }
                      }
                      n1473 = Greater?(x=w2475, y=w2474) -> (0:w2473:bool)
                    }
                    frame #2 {
                      n1474 = case shown="True" w2493 {
                        tunnel: w2492 -> [_ _]
                        tunnel: w2491 -> [_ _]
                        frame False {
                          n1475 = One Button Dialog(message="Please select a row below \"To Be Scheduled\" and try again...") -> ()  [unwired: 1 in, 1 out]
                        }
                        frame True {
                          w2495 = TRUE ("Visible")
                          n1476 = property on="System Select" class="Ring (strict)"() -> ("Strings []"=w2496:string[])  [unwired: 2 in, 2 out]
                          n1477 = property on="System Select Cluster" class="Clust"("Visible"=w2495) -> ()  [unwired: 2 in, 2 out]
                          n1478 = property on="Select System" class="Ring (strict)"("Strings []"=w2496) -> ()  [unwired: 2 in, 2 out]
                          n1479 = property on="Select System" class="Ring (strict)"("Blinking"=w2495) -> ()  [unwired: 2 in, 2 out]
                        }
                      }
                    }
                    frame #3 {
                      # "Get system number form user"
                      n1480 = case shown="True" w2499 {
                        tunnel: [_ w2502] -> w2498
                        tunnel: [_ w2501] -> w2497
                        frame False {
                        }
                        frame True {
                          n1481 = while {
                            tunnel: [w2507] -> w2502
                            tunnel: [w2505] -> w2501
                            tunnel: [w2504] -> w2500
                            stop <- w2504 stop-if-true
                            n1482 = Unbundle By Name("System Select Cluster") -> ("Select System"=w2507:u16, "OK Button"=w2505:bool, "Cancel Button"=w2506:bool)
                            n1483 = Or(x=w2505, y=w2506) -> (x .or. y?=w2504:bool)
                            n1484 = Wait (ms)(milliseconds to wait=u32 200) -> ()  [unwired: 1 out]
                          }
                          n1485 = flat-sequence {
                            tunnel: w2500 -> [_]
                            frame #0 {
                              w2503 = FALSE ("Visible")
                              n1486 = property on="System Select Cluster" class="Clust"("Visible"=w2503) -> ()  [unwired: 2 in, 2 out]
                              n1487 = property on="Select System" class="Ring (strict)"("Blinking"=w2503) -> ()  [unwired: 2 in, 2 out]
                            }
                          }
                        }
                      }
                    }
                    frame #4 {
                      # "open the \"move to\" worksheet and add the row to the bottom, save, and open the \"move to\" sheet"
                      n1488 = case shown="True" w2511 {
                        tunnel: w2514 -> [_ w2518]
                        tunnel: w2513 -> [_ w2516]
                        tunnel: w2512 -> [_ w2521]
                        tunnel: w2510 -> [_ w2517]
                        frame False {
                        }
                        frame True {
                          n1489 = property on="System Select" class="Ring (strict)"() -> ("Strings []"=w2523:string[])  [unwired: 2 in, 2 out]
                          n1490 = Index Array(array=w2523, index=w2518) -> (element=w2515:string)
                          n1491 = Path To String(path=w2516) -> (string=w2527:string)
                          n1492 = Concatenate Strings(w2527, "\\Run Worksheets\\" ("string"), "System " ("string"), w2515, " Run Worksheet.txt" ("string")) -> (w2528:string)
                          n1493 = String To Path(string=w2528) -> (path=w2519:path)
                          n1494 = call-poly <vilib>:"Read Delimited Spreadsheet.vi"("file path (dialog if empty)"=w2519) -> ("all rows"=w2522:string[][])  [unwired: 9 in, 5 out]
                          n1495 = Insert Into Array(array=w2522, new element=w2521) -> (w2520:string[][])  [unwired: 2 in]
                          n1496 = stacked-sequence {
                            tunnel: w2520 -> [_ _ w2535 _ _ _ _ _]
                            tunnel: w2518 -> [_ _ _ _ _ _ _ w2545]
                            tunnel: w2517 -> [_ _ _ _ w2537 _ _ _]
                            tunnel: w2515 -> [_ _ w2534 _ _ _ _ _]
                            frame #0 {
                              n1497 = call "Message Sched.vi"("Message 2"="Moving selected row to the new worksheet.  Please wait...", "Message Control"=TRUE, "Show Abort"=FALSE) -> ()  [unwired: 2 in, 1 out]
                            }
                            frame #1 {
                              n1498 = Wait (ms)(milliseconds to wait=u32 500) -> ()  [unwired: 1 out]
                            }
                            frame #2 {
                              # "Save the \"move to\" worksheet"
                              n1499 = call "Save Run Worksheet to 2 Folders.vi"("Message 1"="Coating Schedule Run Builder - Save Worksheet after User \"Copy to\":", "System Select Text"=w2534, "Run Worksheet IN"=w2535) -> ()  [unwired: 8 in, 1 out]
                            }
                            frame #3 {
                              n1500 = Wait (ms)(milliseconds to wait=u32 500) -> ()  [unwired: 1 out]
                            }
                            frame #4 {
                              # "Delete the row from the \"copy from\" worksheet"
                              n1501 = local read "Run Worksheet"() -> (w2538:string[][])
                              n1502 = Delete From Array(array=w2538, index (row)=w2537) -> (array with subset deleted=w2539:string[][])  [unwired: 2 in, 1 out]
                              n1503 = local write "Run Worksheet"(w2539) -> ()
                            }
                            frame #5 {
                              # "Save \"copy from\" with row removed"
                              n1504 = property on="System Select" class="Ring (strict)"() -> ("RingText.Text"=w2541:string)  [unwired: 2 in, 2 out]
                              n1505 = local read "Run Worksheet"() -> (w2542:string[][])
                              n1506 = call "Save Run Worksheet to 2 Folders.vi"("Message 1"="Coating Schedule Run Builder - Save Worksheet after User \"Copy From\":", "System Select Text"=w2541, "Run Worksheet IN"=w2542) -> ()  [unwired: 8 in, 1 out]
                            }
                            frame #6 {
                              n1507 = Wait (ms)(milliseconds to wait=u32 500) -> ()  [unwired: 1 out]
                            }
                            frame #7 {
                              # "Go to the \"move to\" worksheet"
                              n1508 = local write "System Select"(w2545) -> ()
                              n1509 = call "Message Sched.vi"("Message Control"=FALSE) -> ()  [unwired: 4 in, 1 out]
                            }
                          }
                        }
                      }
                    }
                  }
                }
              }
            }
            frame #10 {
              n1510 = local read "Pick Design was True"() -> (w2550:bool)
              n1511 = Not Equal?(x="Reset Substrate List", y=w2549) -> (x != y?=w2548:bool)
              n1512 = And(x=w2550, y="Reset Substrate List") -> (x .and. y?=w2551:bool)
              n1513 = And(x="Reset Substrate List", y=w2548) -> (x .and. y?=w2546:bool)
              n1514 = case shown="False" w2551 {
                tunnel: "Reset Substrate List" -> [w2556 _]
                tunnel: w2550 -> [w2554 _]
                frame False {
                  n1515 = Not(x=w2556) -> (.not. x?=w2555:bool)
                  n1516 = And(x=w2554, y=w2555) -> (x .and. y?=w2553:bool)
                  n1517 = case shown="False" w2553 {
                    frame False {
                    }
                    frame True {
                      n1518 = local read "Reset Substrate Timer Start"() -> (w2561:u32)
                      n1519 = Tick Count (ms)() -> (millisecond timer value=w2558:u32)
                      n1520 = Subtract(x=w2558, y=w2561) -> (x-y=w2560:u32)
                      n1521 = Greater?(x=w2560, y=u32 20000) -> (0:w2557:bool)
                      n1522 = case shown="True" w2557 {
                        frame False {
                        }
                        frame True {
                          n1523 = local write "Pick Design was True"(FALSE ("Pick Design was True")) -> ()
                        }
                      }
                    }
                  }
                }
                frame True {
                  # "Reset Substrate list after time delay"
                  n1524 = local read "Reset Substrate Timer Start"() -> (w2566:u32)
                  n1525 = Tick Count (ms)() -> (millisecond timer value=w2567:u32)
                  n1526 = Subtract(x=w2567, y=w2566) -> (x-y=w2565:u32)
                  n1527 = Greater?(x=w2565, y=u32 20000) -> (0:w2563:bool)
                  n1528 = case shown="True" w2563 {
                    frame False {
                    }
                    frame True {
                      n1529 = local read "SubstrateStrings"() -> (w2569:string[])
                      n1530 = local write "Pick Design was True"(FALSE ("Pick Design was true")) -> ()
                      n1531 = property on="Substrate" class="Ring (strict)"("Strings []"=w2569) -> ()  [unwired: 2 in, 2 out]
                    }
                  }
                }
              }
              n1532 = case shown="False" w2546 {
                frame False {
                }
                frame True {
                  n1533 = local read "SubstrateStrings"() -> (w2552:string[])
                  n1534 = property on="Substrate" class="Ring (strict)"("Strings []"=w2552) -> ()  [unwired: 2 in, 2 out]
                }
              }
            }
            frame #11 {
              n1535 = case shown="True" "Save Column Widths as Default" {
                frame False {
                }
                frame True {
                  n1536 = local read "Run Worksheet"() -> (w2582:string[][])
                  n1537 = local write "Save Column Widths as Default"(FALSE ("Set Column Widths as Default")) -> ()
                  n1538 = Index Array(array=w2582, index (row)=0) -> (element=w2580:string[])  [unwired: 1 in]
                  n1539 = for {
                    tunnel: w2580 -> [_] mode=indexing
                    tunnel: [w2583] -> w2575 mode=indexing
                    i -> [w2584]
                    n1540 = stacked-sequence {
                      tunnel: w2584 -> [w2587 _]
                      tunnel: [_ w2588] -> w2583
                      frame #0 {
                        n1541 = Bundle(0, w2587) -> (w2585:cluster{i32, i32})  [unwired: 1 in]
                        n1542 = property on="Run Worksheet" class="Tbl (strict)"("Active Cell:Active Cell"=w2585) -> ()  [unwired: 2 in, 2 out]
                      }
                      frame #1 {
                        n1543 = property on="Run Worksheet" class="Tbl (strict)"() -> ("Active Cell:Cell Size:Width"=w2588:u32)  [unwired: 2 in, 2 out]
                      }
                    }
                  }
                  n1544 = global read "Schedule Control Globals.vi" "Start path"() -> (w2573:path)
                  n1545 = Strip Path(path=w2573) -> (stripped path=w2577:path)  [unwired: 1 out]
                  n1546 = Path To String(path=w2577) -> (string=w2576:string)
                  n1547 = Concatenate Strings(w2576, "\\Run Builder Worksheet Table Column Widths.txt" ("string")) -> (w2579:string)
                  n1548 = Number To Decimal String(number=w2575) -> (decimal integer string=w2571:string[])  [unwired: 1 in]
                  n1549 = String To Path(string=w2579) -> (path=w2572:path)
                  n1550 = call-poly <vilib>:"Write Delimited Spreadsheet.vi"("file path (dialog if empty)"=w2572, "1D data"=w2571) -> ()  [unwired: 12 in, 2 out]
                }
              }
            }
            frame #12 {
              n1551 = property on="Transfer to Schedule" class="Bool"() -> ("DisabledEnum"=w2590:T5)  [unwired: 2 in, 2 out]
              n1552 = Not Equal?(x=w2590, y=w2589) -> (x != y?=w2591:bool)
              n1553 = case shown="True" w2591 {
                tunnel: w2590 -> [_ w2593]
                frame False {
                }
                frame True {
                  n1554 = case shown="\"Disabled and Grayed Out\"" w2593 {
                    tunnel: ["Transfers to the active sheet on the coating schedule program." ("Tip Strip") "The data transfer did not save if control remains grayed out.  Check schedule and close and re-open the run builder to reset." ("Tip Strip")] -> w2592
                    frame "Enabled", Default {
                    }
                    frame "Disabled and Grayed Out" {
                    }
                  }
                  n1555 = property on="Transfer to Schedule" class="Bool"("TipStrip"=w2592) -> ()  [unwired: 2 in, 2 out]
                }
              }
            }
          }
        }
      }
    }
    n1556 = event shown="[0] Timeout" {
      selector: _ -> [_ _]
      dyn-events: _ -> [_ _]
      timeout: 200 -> [_ _]
      tunnel: [_ TRUE ("Discard?")] -> w193
      event Timeout {
        n1557 = event-data() -> ()  [unwired: 1 in, 1 out]
      }
      event Panel Close? {
        n1558 = event-data() -> ()  [unwired: 1 in, 3 out]
        n1559 = global read "Schedule Control Globals.vi" "Sing Time Zone"() -> (w2597:bool)
        n1560 = stacked-sequence {
          seq-local: [w2600 _ _] -> [_ _ w2624]
          seq-local: [w2599 _ _] -> [_ w2608 _]
          seq-local: [_ w2607 _] -> [_ _ w2622]
          tunnel: w2597 -> [_ _ w2616]
          frame #0 {
            n1561 = property on="Converted Data Table" class="Tbl (strict)"() -> ("Column Headers[]"=w2599:string[])  [unwired: 2 in, 2 out]
            n1562 = for {
              tunnel: w2599 -> [_] mode=indexing
              tunnel: [w2602] -> w2600 mode=indexing
              i -> [w2601]
              n1563 = stacked-sequence {
                tunnel: [_ w2606] -> w2602
                tunnel: w2601 -> [w2605 _]
                frame #0 {
                  n1564 = Bundle(0, w2605) -> (w2603:cluster{i32, i32})  [unwired: 1 in]
                  n1565 = property on="Converted Data Table" class="Tbl (strict)"("Active Cell"=w2603) -> ()  [unwired: 2 in, 2 out]
                }
                frame #1 {
                  n1566 = property on="Converted Data Table" class="Tbl (strict)"() -> ("Width"=w2606:u32)  [unwired: 2 in, 2 out]
                }
              }
            }
          }
          frame #1 {
            # "Replace Carriage Returns"
            n1567 = for {
              tunnel: w2608 -> [w2613] mode=indexing
              tunnel: [w2611] -> w2607 mode=indexing
              n1568 = Search and Replace String(replace all?=TRUE ("replace all? (F)"), input string=w2613, search string="\n", replace string="&^" ("replace string (\"\")")) -> (result string=w2611:string)  [unwired: 4 in, 3 out]
            }
          }
          frame #2 {
            n1569 = local read "Coating Que / CTCL (T)?"() -> (w2620:bool)
            n1570 = global read "Schedule Control Globals.vi" "Start path"() -> (w2629:path)
            n1571 = local read "Report Name"() -> (w2619:string)
            n1572 = Number To Decimal String(number=w2624) -> (decimal integer string=w2623:string[])  [unwired: 1 in]
            n1573 = Strip Path(path=w2629) -> (stripped path=w2628:path)  [unwired: 1 out]
            n1574 = Equal?(x=w2619, y="SAP CTCL Activity" ("Report Name")) -> (x = y?=w2617:bool)
            n1575 = case shown="True" w2620 {
              tunnel: ["Run Builder Que Report Table Column Widths.txt" ("text") w2633] -> w2621
              tunnel: w2617 -> [_ w2632]
              tunnel: w2616 -> [_ w2631]
              frame False {
              }
              frame True {
                n1576 = case shown="True" w2632 {
                  tunnel: ["Run Builder CTCL Report Table Column Widths.txt" ("text") w2636] -> w2633
                  tunnel: w2631 -> [_ w2635]
                  frame False {
                  }
                  frame True {
                    n1577 = case shown="True" w2635 {
                      tunnel: ["Run Builder SAP CTCL Report Table Column Widths.txt" ("text") "Run Builder SAP Sing CTCL Report Table Column Widths.txt" ("text")] -> w2636
                      frame False {
                      }
                      frame True {
                      }
                    }
                  }
                }
              }
            }
            n1578 = Path To String(path=w2628) -> (string=w2627:string)
            n1579 = Build Array(w2622, w2623) -> (w2614:string[][])
            n1580 = Concatenate Strings(w2627, "\\" ("string"), w2621) -> (w2625:string)
            n1581 = String To Path(string=w2625) -> (path=w2615:path)
            n1582 = call-poly <vilib>:"Write Delimited Spreadsheet.vi"("file path (dialog if empty)"=w2615, "2D data"=w2614) -> ()  [unwired: 12 in, 2 out]
          }
        }
        n1583 = event-data("Discard?"=FALSE) -> ()  [unwired: 1 in, 1 out]
      }
    }
  }
  n1584 = local write "Substrate"(w3) -> ()
